vi "Beampointing_Multi_Pico3_upstairs01.vi"() -> ()   [LabVIEW 2020]
uses:
  Shared/GUI_Template/GUI_master/tcp_new_data_event.ctl
  Shared/GUI_Template/GUI_master/tcp new data cluster.ctl
  Ctrs/beam detection.ctl
  GUI_Beampointing_single_TRA/Ctrs/move.ctl
  General GUIs/Device GUIs/GUI_Cameras/Controls/Crosshair type def.ctl
  <vilib>/Utility/error.llb/DialogType.ctl
  <vilib>/Utility/file.llb/Read From Spreadsheet File (string).vi
  <userlib>/_OpenG.lib/array/array.llb/Filter 1D Array with Scalar (String)__ogtk.vi
  <userlib>/_OpenG.lib/array/array.llb/Filter 1D Array (String)__ogtk.vi
  <vilib>/Utility/file.llb/Write To Spreadsheet File (string).vi
  <vilib>/Analysis/NI_AALBase.lvlib
panel:
  out "x-y*floor(x/y)":dbl
  out "error out":errorcluster
  out "config path":string
  out "Array 3":bool[](array[boolean])
  out "Array 2":u16[](array[numeric])
  out "Array":u16[](array[numeric])
  out "Moving Y":string
  out "Moving X":string
  out "particles":T1(array[cluster])
  out "millisecond timer value":u32
  out "appended path":path
  out "millisecond timer 2":u32
  in  "GUIdevice 98":string="PicoPad4"
  in  "Position.Axis 111::98":dbl=77.0 caption="Motor Axis 1" min=-30000.0 max=30000.0 format="%#_6f"
  in  "Position.Axis 112::98":dbl=77.0 caption="Motor Axis 1" min=-20000.0 max=20000.0 format="%#_6f"
  in  "Position.Axis 113::98":dbl=77.0 caption="Motor Axis 1" min=-20000.0 max=20000.0 format="%#_6f"
  in  "Position.Axis 121::98":dbl=77.0 caption="Motor Axis 1" min=-999999.0 max=999999.0 format="%#_6f"
  in  "Position.Axis 122::98":dbl=77.0 caption="Motor Axis 1" min=-999999.0 max=999999.0 format="%#_6f"
  in  "Position.Axis 123::98":dbl=77.0 caption="Motor Axis 1" min=-999999.0 max=999999.0 format="%#_6f"
  in  "Position.Axis 131::98":dbl=77.0 caption="Motor Axis 1" min=-999999.0 max=999999.0 format="%#_6f"
  in  "Position.Axis 132::98":dbl=77.0 caption="Motor Axis 1" min=-999999.0 max=999999.0 format="%#_6f"
  in  "Position.Axis 133::98":dbl=77.0 caption="Motor Axis 1" min=-999999.0 max=999999.0 format="%#_6f"
  in  "Position.Axis 141::98":dbl=77.0 caption="Motor Axis 1" min=-999999.0 max=999999.0 format="%#_6f"
  in  "Position.Axis 142::98":dbl=77.0 caption="Motor Axis 1" min=-999999.0 max=999999.0 format="%#_6f"
  in  "Position.Axis 143::98":dbl=77.0 caption="Motor Axis 1" min=-999999.0 max=999999.0 format="%#_6f"
  in  "Position.Axis 211::98":dbl=77.0 caption="Motor Axis 1" min=-999999.0 max=999999.0 format="%#_6f"
  in  "Position.Axis 212::98":dbl=77.0 caption="Motor Axis 1" min=-999999.0 max=999999.0 format="%#_6f"
  in  "Position.Axis 213::98":dbl=77.0 caption="Motor Axis 1" min=-999999.0 max=999999.0 format="%#_6f"
  in  "Position.Axis 221::98":dbl=77.0 caption="Motor Axis 1" min=-999999.0 max=999999.0 format="%#_6f"
  in  "Position.Axis 222::98":dbl=77.0 caption="Motor Axis 1" min=-999999.0 max=999999.0 format="%#_6f"
  in  "Position.Axis 223::98":dbl=77.0 caption="Motor Axis 1" min=-999999.0 max=999999.0 format="%#_6f"
  in  "Position.Axis 231::98":dbl=77.0 caption="Motor Axis 1" min=-999999.0 max=999999.0 format="%#_6f"
  in  "Position.Axis 232::98":dbl=77.0 caption="Motor Axis 1" min=-999999.0 max=999999.0 format="%#_6f"
  in  "Position.Axis 233::98":dbl=77.0 caption="Motor Axis 1" min=-999999.0 max=999999.0 format="%#_6f"
  in  "Position.Axis 241::98":dbl=77.0 caption="Motor Axis 1" min=-999999.0 max=999999.0 format="%#_6f"
  in  "Position.Axis 242::98":dbl=77.0 caption="Motor Axis 1" min=-999999.0 max=999999.0 format="%#_6f"
  in  "Position.Axis 243::98":dbl=77.0 caption="Motor Axis 1" min=-999999.0 max=999999.0 format="%#_6f"
  in  "Position.Axis 311::98":dbl=77.0 caption="Motor Axis 1" min=-999999.0 max=999999.0 format="%#_6f"
  in  "Position.Axis 312::98":dbl=77.0 caption="Motor Axis 1" min=-999999.0 max=999999.0 format="%#_6f"
  in  "Position.Axis 313::98":dbl=77.0 caption="Motor Axis 1" min=-999999.0 max=999999.0 format="%#_6f"
  in  "Position.Axis 321::98":dbl=77.0 caption="Motor Axis 1" min=-999999.0 max=999999.0 format="%#_6f"
  in  "Position.Axis 322::98":dbl=77.0 caption="Motor Axis 1" min=-999999.0 max=999999.0 format="%#_6f"
  in  "Position.Axis 323::98":dbl=77.0 caption="Motor Axis 1" min=-999999.0 max=999999.0 format="%#_6f"
  in  "Position.Axis 331::98":dbl=77.0 caption="Motor Axis 1" min=-999999.0 max=999999.0 format="%#_6f"
  in  "Position.Axis 332::98":dbl=77.0 caption="Motor Axis 1" min=-999999.0 max=999999.0 format="%#_6f"
  in  "Position.Axis 333::98":dbl=77.0 caption="Motor Axis 1" min=-999999.0 max=999999.0 format="%#_6f"
  in  "Position.Axis 341::98":dbl=77.0 caption="Motor Axis 1" min=-999999.0 max=999999.0 format="%#_6f"
  in  "Position.Axis 342::98":dbl=77.0 caption="Motor Axis 1" min=-999999.0 max=999999.0 format="%#_6f"
  in  "Position.Axis 343::98":dbl=77.0 caption="Motor Axis 1" min=-999999.0 max=999999.0 format="%#_6f"
  in  "Position.Axis 411::98":dbl=77.0 caption="Motor Axis 1" min=-999999.0 max=999999.0 format="%#_6f"
  in  "Position.Axis 412::98":dbl=77.0 caption="Motor Axis 1" min=-999999.0 max=999999.0 format="%#_6f"
  in  "Position.Axis 413::98":dbl=77.0 caption="Motor Axis 1" min=-999999.0 max=999999.0 format="%#_6f"
  in  "Position.Axis 421::98":dbl=77.0 caption="Motor Axis 1" min=-999999.0 max=999999.0 format="%#_6f"
  in  "Position.Axis 422::98":dbl=77.0 caption="Motor Axis 1" min=-999999.0 max=999999.0 format="%#_6f"
  in  "Position.Axis 423::98":dbl=77.0 caption="Motor Axis 1" min=-999999.0 max=999999.0 format="%#_6f"
  in  "Position.Axis 431::98":dbl=77.0 caption="Motor Axis 1" min=-999999.0 max=999999.0 format="%#_6f"
  in  "Position.Axis 432::98":dbl=77.0 caption="Motor Axis 1" min=-999999.0 max=999999.0 format="%#_6f"
  in  "Position.Axis 433::98":dbl=77.0 caption="Motor Axis 1" min=-999999.0 max=999999.0 format="%#_6f"
  in  "Position.Axis 441::98":dbl=77.0 caption="Motor Axis 1" min=-999999.0 max=999999.0 format="%#_6f"
  in  "Position.Axis 442::98":dbl=77.0 caption="Motor Axis 1" min=-999999.0 max=999999.0 format="%#_6f"
  in  "Position.Axis 443::98":dbl=77.0 caption="Motor Axis 1" min=-999999.0 max=999999.0 format="%#_6f"
  in  "Position.Axis 511::98":dbl=77.0 caption="Motor Axis 1" min=-999999.0 max=999999.0 format="%#_6f"
  in  "Position.Axis 512::98":dbl=77.0 caption="Motor Axis 1" min=-999999.0 max=999999.0 format="%#_6f"
  in  "Position.Axis 513::98":dbl=77.0 caption="Motor Axis 1" min=-999999.0 max=999999.0 format="%#_6f"
  in  "Position.Axis 521::98":dbl=77.0 caption="Motor Axis 1" min=-999999.0 max=999999.0 format="%#_6f"
  in  "Position.Axis 522::98":dbl=77.0 caption="Motor Axis 1" min=-999999.0 max=999999.0 format="%#_6f"
  in  "Position.Axis 523::98":dbl=77.0 caption="Motor Axis 1" min=-999999.0 max=999999.0 format="%#_6f"
  in  "Position.Axis 531::98":dbl=77.0 caption="Motor Axis 1" min=-999999.0 max=999999.0 format="%#_6f"
  in  "Position.Axis 532::98":dbl=77.0 caption="Motor Axis 1" min=-999999.0 max=999999.0 format="%#_6f"
  in  "Position.Axis 533::98":dbl=77.0 caption="Motor Axis 1" min=-999999.0 max=999999.0 format="%#_6f"
  in  "Position.Axis 541::98":dbl=77.0 caption="Motor Axis 1" min=-999999.0 max=999999.0 format="%#_6f"
  in  "Position.Axis 542::98":dbl=77.0 caption="Motor Axis 1" min=-999999.0 max=999999.0 format="%#_6f"
  in  "Position.Axis 543::98":dbl=77.0 caption="Motor Axis 1" min=-999999.0 max=999999.0 format="%#_6f"
  in  "Numeric":dbl
  out "Current State":string
  in  "output cluster 2":T5 {"detection para"."smal para"."Measurement Parameter" items=["Center of Mass X", "Center of Mass Y", "First Pixel X", "First Pixel Y", "Bounding Rect Left", "Bounding Rect Top", "Bounding Rect Right", "Bounding Rect Bottom", "Max Feret Diameter Start X", "Max Feret Diameter Start Y", "Max Feret Diameter End X", "Max Feret Diameter End Y", "Max Horiz. Segment Length Left", "Max Horiz. Segment Length Right", "Max Horiz. Segment Length Row", "-", "Bounding Rect Width", "Bounding Rect Height", "Bounding Rect Diagonal", "Perimeter", "Convex Hull Perimeter", "Holes' Perimeter", "Max Feret Diameter", "Equivalent Ellipse Major Axis", "Equivalent Ellipse Minor Axis", "Equivalent Ellipse Minor Axis (Feret)", "Equivalent Rect Long Side", "Equivalent Rect Short Side", "Equivalent Rect Diagonal", "Equivalent Rect Short Side (Feret)", "Average Horiz. Segment Length", "Average Vert. Segment Length", "Hydraulic Radius", "Waddel Disk Diameter", "-", "Area", "Holes' Area", "Particle & Holes' Area", "Convex Hull Area", "Image Area", "-", "Number of Holes", "Number of Horiz. Segments", "Number of Vert. Segments", "-", "Orientation", "Max Feret Diameter Orientation", "-", "% Area/Image Area", "% Area/(Particle & Holes' Area)", "Ratio of Equivalent Ellipse Axes", "Ratio of Equivalent Rect Sides", "-", "Elongation Factor", "Compactness Factor", "Heywood Circularity Factor", "Type Factor", "-", "Sum X", "Sum Y", "Sum XX", "Sum XY", "Sum YY", "Sum XXX", "Sum XXY", "Sum XYY", "Sum YYY", "-", "Moment of Inertia XX", "Moment of Inertia XY", "Moment of Inertia YY", "Moment of Inertia XXX", "Moment of Inertia XXY", "Moment of Inertia XYY", "Moment of Inertia YYY", "Norm. Moment of Inertia XX", "Norm. Moment of Inertia XY", "Norm. Moment of Inertia YY", "Norm. Moment of Inertia XXX", "Norm. Moment of Inertia XXY", "Norm. Moment of Inertia XYY", "Norm. Moment of Inertia YYY", "Hu Moment 1", "Hu Moment 2", "Hu Moment 3", "Hu Moment 4", "Hu Moment 5", "Hu Moment 6", "Hu Moment 7"]; "detection para"."smal para"."Range Lower Value" format="%.2f"; "detection para"."smal para"."Range Upper Value" format="%.2f"; "detection para"."detection method" items=["clustering", "entropy", "metric", "moments", "inter-class variance"]; "detection para"."Filter" items=["No Filter", "Median Filter", "Low Pass Filter"]}
  out "CCDs":string[](array[string])
  in  "GUIdevice 12":string
  in  "GUIdevice 11":string
  in  "GUIdevice 10":string
  in  "GUIdevice 9":string
  out "error out 2":errorcluster
  in  "active cams":string[](array[string])
  in  "Motor Y":dbl[][](array[numeric])
  in  "Motor X":dbl[][](array[numeric])
  out "Names":string[](array[string])
  in  "Offset X stats":dbl[][](array[numeric])
  in  "Offset Y stats":dbl[][](array[numeric])
  out "Box":T6(array[cluster])
  in  "Tab Control 2":enum32{"Config ", "Main", "History"}(tab)=enum."Main"
  out "Waveform Chart":u32(graph)
  in  "associated motors":T7
  out "Cameras":T8
  out "Status":cluster{i32, i32, "Centroid X":dbl[][]}(graph)
  in  "Exposure:12":dbl=0.095 min=0.0001 max=1.0 format="%#_6f"
  in  "Triggerdelay::12":dbl=0.003 min=0.0 max=0.09 format="%#_6f"
  in  "Exposure::11":dbl=0.095 min=0.0001 max=1.0 format="%#_6f"
  in  "Triggerdelay::11":dbl=0.003 min=0.0 max=0.09 format="%#_6f"
  in  "Exposure::10":dbl=0.095 min=0.0001 max=1.0 format="%#_6f"
  in  "Triggerdelay::10":dbl=0.003 min=0.0 max=0.09 format="%#_6f"
  in  "Exposure::9":dbl=0.095 min=0.0001 max=1.0 format="%#_6f"
  in  "Triggerdelay::9":dbl=0.003 min=0.0 max=0.09 format="%#_6f"
  in  "Trigger::9":bool
  in  "Trigger::10":bool caption="Trigger:10"
  in  "Trigger::11":bool
  in  "Trigger::12":bool
  in  "Target.Y::9":dbl=45.0 caption="T9y" min=0.0 max=2000.0 format="%#_6f"
  in  "Target.X::9":dbl=47.0 caption="Tx9" min=0.0 max=2000.0 format="%#_6f"
  in  "Target.Y::10":dbl=45.0 caption="T10y" min=0.0 max=2000.0 format="%#_6f"
  in  "Target.X::10":dbl=47.0 caption="T10x" min=0.0 max=2000.0 format="%#_6f"
  in  "Target.Y::11":dbl=45.0 caption="T11y" min=0.0 max=2000.0 format="%#_6f"
  in  "Target.X::11":dbl=47.0 caption="T11x" min=0.0 max=2000.0 format="%#_6f"
  in  "Target.Y::12":dbl=45.0 caption="T12y" min=0.0 max=2000.0 format="%#_6f"
  in  "Target.X::12":dbl=47.0 caption="T12x" min=0.0 max=2000.0 format="%#_6f"
  in  "Exposure::8":dbl=0.095 min=0.0001 max=1.0 format="%#_6f"
  in  "Triggerdelay::8":dbl=0.003 min=0.0 max=0.09 format="%#_6f"
  in  "Trigger::8":bool
  in  "Target.Y::8":dbl=45.0 caption="T8y" min=0.0 max=2000.0 format="%#_6f"
  in  "Target.X::8":dbl=47.0 caption="T8x" min=0.0 max=2000.0 format="%#_6f"
  in  "Target.Y::7":dbl=45.0 caption="T7x" min=0.0 max=2000.0 format="%#_6f"
  in  "Target.X::7":dbl=47.0 caption="T7y" min=0.0 max=2000.0 format="%#_6f"
  in  "Target.Y::6":dbl=45.0 caption="T6y" min=1.0 max=600.0 format="%#_6f"
  in  "Target.X::6":dbl=47.0 caption="T6x" min=1.0 max=800.0 format="%#_6f"
  in  "Target.Y::5":dbl=45.0 caption="T5y" min=0.0 max=2000.0 format="%#_6f"
  in  "Target.X::5":dbl=47.0 caption="T5x" min=0.0 max=2000.0 format="%#_6f"
  in  "Target.Y::4":dbl=45.0 caption="T4y" min=1.0 max=600.0 format="%#_6f"
  in  "Target.X::4":dbl=47.0 caption="T4x" min=1.0 max=800.0 format="%#_6f"
  in  "Target.Y::3":dbl=163.0 caption="T3y" min=0.0 max=2000.0 format="%#_6f"
  in  "Target.X::3":dbl=152.0 caption="T3x" min=0.0 max=2000.0 format="%#_6f"
  in  "Target.Y::2":dbl=74.0 caption="T2y" min=1.0 max=600.0 format="%#_6f"
  in  "Target.X::2":dbl=75.0 caption="T2x" min=1.0 max=800.0 format="%#_6f"
  in  "Target.Y::1":dbl=61.0 caption="T1y" min=1.0 max=600.0 format="%#_6f"
  in  "Target.X::1":dbl=77.0 caption="T1x" min=1.0 max=800.0 format="%#_6f"
  in  "Exposure::7":dbl=0.095 min=0.0001 max=1.0 format="%#_6f"
  in  "Triggerdelay::7":dbl=0.003 min=0.0 max=0.09 format="%#_6f"
  in  "Trigger::7":bool
  in  "Exposure::6":dbl=0.095 min=0.0001 max=1.0 format="%#_6f"
  in  "Triggerdelay::6":dbl=0.003 min=0.0 max=0.09 format="%#_6f"
  in  "Trigger::6":bool
  in  "Exposure::5":dbl=0.095 min=1e-05 max=2.0 format="%#_6f"
  in  "Triggerdelay::5":dbl=0.003 min=0.0 max=100000.0 format="%#_6f"
  in  "Trigger::5":bool
  in  "Exposure::4":dbl=0.095 min=0.0001 max=1.0 format="%#_6f"
  in  "Triggerdelay::4":dbl=0.003 min=0.0 max=0.09 format="%#_6f"
  in  "Trigger::4":bool
  in  "Exposure::3":dbl=0.095 min=1e-05 max=2.0 format="%#_6f"
  in  "Triggerdelay::3":dbl=0.003 min=0.0 max=0.09 format="%#_6f"
  in  "Trigger::3":bool
  in  "Exposure::2":dbl=0.095 min=0.0001 max=1.0 format="%#_6f"
  in  "Triggerdelay::2":dbl=0.003 min=0.0 max=0.09 format="%#_6f"
  in  "Trigger::2":bool
  out "image::1":T9(plugin-control) caption="regen-out-cam"
  out "image::2":T9(plugin-control) caption="xpw-cam"
  out "image::3":T9(plugin-control) caption="xpw-out-cam"
  out "image::4":T9(plugin-control) caption="amp0-out-cam"
  out "image::5":T9(plugin-control) caption="preamp-in-cam"
  out "image::6":T9(plugin-control) caption="preamp-2nd-pass-cam"
  out "image::7":T9(plugin-control) caption="compressor-in-cam"
  out "image::8":T9(plugin-control) caption="compressor-out-cam"
  in  "Exposure::1":dbl=0.095 caption="exposure" min=0.0001 max=1.0 format="%#_6f"
  in  "Triggerdelay::1":dbl=0.003 caption="trig delay" min=0.0 max=0.09 format="%#_6f"
  in  "Trigger::1":bool
  in  "UDP error message":string
  out "required Y":bool[](array[boolean])
  out "required X":bool[](array[boolean])
  out "detected":bool[](array[boolean])
  out "name array":string[](array[string])
  out "image::9":T9(plugin-control)
  out "image::10":T9(plugin-control)
  out "image::11":T9(plugin-control)
  out "image::12":T9(plugin-control)
  out "speedmode X":bool[](array[boolean])
  out "speedmode Y":bool[](array[boolean])
  out "CCD 9":cluster{timestamp[], dbl[]}[](graph)
  out "CCD 10":cluster{timestamp[], dbl[]}[](graph)
  out "CCD 11":cluster{timestamp[], dbl[]}[](graph)
  out "CCD 12":cluster{timestamp[], dbl[]}[](graph)
  out "CCD 5":cluster{timestamp[], dbl[]}[](graph)
  out "CCD 6":cluster{timestamp[], dbl[]}[](graph)
  out "CCD 7":cluster{timestamp[], dbl[]}[](graph)
  out "CCD 8":cluster{timestamp[], dbl[]}[](graph)
  out "CCD 2":cluster{timestamp[], dbl[]}[](graph)
  out "CCD 1":cluster{timestamp[], dbl[]}[](graph)
  out "CCD 3":cluster{timestamp[], dbl[]}[](graph)
  out "CCD 4":cluster{timestamp[], dbl[]}[](graph)
  out "History index":i32
  in  "History Size":i32=500
  out "Particle Reports (Pixels)":T10(array[cluster])
  in  "Feedback Global":bool
  in  "detection para":T3[](array[typedef])=[{"Filter"=1, "Filter Para"={"X Size"=5, "Y Size"=5, "% Tolerance"=1}, "detection method"=4, "smal para"=[{"Measurement Parameter"=35, "Range Lower Value"=0.0, "Range Upper Value"=0.0, "Range"=TRUE, "Measurement Type"=FALSE}], "Remove small Objects"=TRUE, "Restrict to round Objects"=FALSE}, {"Filter"=1, "Filter Para"={"X Size"=5, "Y Size"=5, "% Tolerance"=1}, "detection method"=4, "smal para"=[{"Measurement Parameter"=35, "Range Lower Value"=0.0, "Range Upper Value"=500.0, "Range"=FALSE, "Measurement Type"=FALSE}], "Remove small Objects"=TRUE, "Restrict to round Objects"=FALSE}, {"Filter"=1, "Filter Para"={"X Size"=5, "Y Size"=5, "% Tolerance"=1}, "detection method"=4, "smal para"=[{"Measurement Parameter"=35, "Range Lower Value"=0.0, "Range Upper Value"=500.0, "Range"=TRUE, "Measurement Type"=FALSE}], "Remove small Objects"=TRUE, "Restrict to round Objects"=FALSE}, {"Filter"=1, "Filter Para"={"X Size"=5, "Y Size"=5, "% Tolerance"=1}, "detection method"=4, "smal para"=[{"Measurement Parameter"=35, "Range Lower Value"=0.0, "Range Upper Value"=500.0, "Range"=TRUE, "Measurement Type"=FALSE}], "Remove small Objects"=TRUE, "Restrict to round Objects"=FALSE}, {"Filter"=1, "Filter Para"={"X Size"=5, "Y Size"=5, "% Tolerance"=1}, "detection method"=4, "smal para"=[{"Measurement Parameter"=35, "Range Lower Value"=0.0, "Range Upper Value"=500.0, "Range"=TRUE, "Measurement Type"=FALSE}], "Remove small Objects"=TRUE, "Restrict to round Objects"=FALSE}, {"Filter"=1, "Filter Para"={"X Size"=5, "Y Size"=5, "% Tolerance"=1}, "detection method"=4, "smal para"=[{"Measurement Parameter"=35, "Range Lower Value"=0.0, "Range Upper Value"=500.0, "Range"=TRUE, "Measurement Type"=FALSE}], "Remove small Objects"=TRUE, "Restrict to round Objects"=FALSE}, {"Filter"=1, "Filter Para"={"X Size"=5, "Y Size"=5, "% Tolerance"=1}, "detection method"=4, "smal para"=[{"Measurement Parameter"=35, "Range Lower Value"=0.0, "Range Upper Value"=500.0, "Range"=TRUE, "Measurement Type"=FALSE}], "Remove small Objects"=TRUE, "Restrict to round Objects"=FALSE}, {"Filter"=1, "Filter Para"={"X Size"=5, "Y Size"=5, "% Tolerance"=1}, "detection method"=3, "smal para"=[{"Measurement Parameter"=35, "Range Lower Value"=0.0, "Range Upper Value"=0.0, "Range"=FALSE, "Measurement Type"=FALSE}], "Remove small Objects"=TRUE, "Restrict to round Objects"=FALSE}, {"Filter"=1, "Filter Para"={"X Size"=5, "Y Size"=5, "% Tolerance"=1}, "detection method"=4, "smal para"=[{"Measurement Parameter"=35, "Range Lower Value"=0.0, "Range Upper Value"=0.0, "Range"=FALSE, "Measurement Type"=FALSE}], "Remove small Objects"=TRUE, "Restrict to round Objects"=FALSE}, {"Filter"=1, "Filter Para"={"X Size"=5, "Y Size"=5, "% Tolerance"=1}, "detection method"=4, "smal para"=[{"Measurement Parameter"=35, "Range Lower Value"=0.0, "Range Upper Value"=500.0, "Range"=TRUE, "Measurement Type"=FALSE}], "Remove small Objects"=TRUE, "Restrict to round Objects"=FALSE}, {"Filter"=1, "Filter Para"={"X Size"=5, "Y Size"=5, "% Tolerance"=1}, "detection method"=4, "smal para"=[{"Measurement Parameter"=35, "Range Lower Value"=0.0, "Range Upper Value"=500.0, "Range"=TRUE, "Measurement Type"=FALSE}], "Remove small Objects"=TRUE, "Restrict to round Objects"=FALSE}, {"Filter"=1, "Filter Para"={"X Size"=5, "Y Size"=5, "% Tolerance"=1}, "detection method"=4, "smal para"=[{"Measurement Parameter"=35, "Range Lower Value"=0.0, "Range Upper Value"=500.0, "Range"=TRUE, "Measurement Type"=FALSE}], "Remove small Objects"=TRUE, "Restrict to round Objects"=FALSE}] {"smal para"."Measurement Parameter" items=["Center of Mass X", "Center of Mass Y", "First Pixel X", "First Pixel Y", "Bounding Rect Left", "Bounding Rect Top", "Bounding Rect Right", "Bounding Rect Bottom", "Max Feret Diameter Start X", "Max Feret Diameter Start Y", "Max Feret Diameter End X", "Max Feret Diameter End Y", "Max Horiz. Segment Length Left", "Max Horiz. Segment Length Right", "Max Horiz. Segment Length Row", "-", "Bounding Rect Width", "Bounding Rect Height", "Bounding Rect Diagonal", "Perimeter", "Convex Hull Perimeter", "Holes' Perimeter", "Max Feret Diameter", "Equivalent Ellipse Major Axis", "Equivalent Ellipse Minor Axis", "Equivalent Ellipse Minor Axis (Feret)", "Equivalent Rect Long Side", "Equivalent Rect Short Side", "Equivalent Rect Diagonal", "Equivalent Rect Short Side (Feret)", "Average Horiz. Segment Length", "Average Vert. Segment Length", "Hydraulic Radius", "Waddel Disk Diameter", "-", "Area", "Holes' Area", "Particle & Holes' Area", "Convex Hull Area", "Image Area", "-", "Number of Holes", "Number of Horiz. Segments", "Number of Vert. Segments", "-", "Orientation", "Max Feret Diameter Orientation", "-", "% Area/Image Area", "% Area/(Particle & Holes' Area)", "Ratio of Equivalent Ellipse Axes", "Ratio of Equivalent Rect Sides", "-", "Elongation Factor", "Compactness Factor", "Heywood Circularity Factor", "Type Factor", "-", "Sum X", "Sum Y", "Sum XX", "Sum XY", "Sum YY", "Sum XXX", "Sum XXY", "Sum XYY", "Sum YYY", "-", "Moment of Inertia XX", "Moment of Inertia XY", "Moment of Inertia YY", "Moment of Inertia XXX", "Moment of Inertia XXY", "Moment of Inertia XYY", "Moment of Inertia YYY", "Norm. Moment of Inertia XX", "Norm. Moment of Inertia XY", "Norm. Moment of Inertia YY", "Norm. Moment of Inertia XXX", "Norm. Moment of Inertia XXY", "Norm. Moment of Inertia XYY", "Norm. Moment of Inertia YYY", "Hu Moment 1", "Hu Moment 2", "Hu Moment 3", "Hu Moment 4", "Hu Moment 5", "Hu Moment 6", "Hu Moment 7"]; "smal para"."Range Lower Value" format="%.2f"; "smal para"."Range Upper Value" format="%.2f"; "detection method" items=["clustering", "entropy", "metric", "moments", "inter-class variance"]; "Filter" items=["No Filter", "Median Filter", "Low Pass Filter"]}
  in  "GUIdevice 8":string="B5_CompressorOut"
  in  "Tab Control":T11(tab)
  in  "Center":bool
  in  "Save Stats":bool
  in  "Save Config":bool
  in  "Load Config":bool
  in  "update speed [ms]":i32=5000
  in  "Img to avg":i32=3 min=3 max=200
  in  "Reset History":bool
  in  "save path":path=path "W:/BP_DATA"
  in  "autodetect":bool
  in  "Detection Rate":dbl=0.8 min=0.001 max=1.0
  in  "new tdms":bool
  in  "Speedmode @":dbl=3.0 min=1.0 max=20.0
  in  "Align":bool
  in  "deivice ini":bool
  in  "beam detection para":T3={"Filter"=1, "Filter Para"={"X Size"=5, "Y Size"=5, "% Tolerance"=1}, "detection method"=4, "smal para"=[{"Measurement Parameter"=35, "Range Lower Value"=0.0, "Range Upper Value"=500.0, "Range"=FALSE, "Measurement Type"=FALSE}], "Remove small Objects"=TRUE, "Restrict to round Objects"=FALSE} {"smal para"."Measurement Parameter" items=["Center of Mass X", "Center of Mass Y", "First Pixel X", "First Pixel Y", "Bounding Rect Left", "Bounding Rect Top", "Bounding Rect Right", "Bounding Rect Bottom", "Max Feret Diameter Start X", "Max Feret Diameter Start Y", "Max Feret Diameter End X", "Max Feret Diameter End Y", "Max Horiz. Segment Length Left", "Max Horiz. Segment Length Right", "Max Horiz. Segment Length Row", "-", "Bounding Rect Width", "Bounding Rect Height", "Bounding Rect Diagonal", "Perimeter", "Convex Hull Perimeter", "Holes' Perimeter", "Max Feret Diameter", "Equivalent Ellipse Major Axis", "Equivalent Ellipse Minor Axis", "Equivalent Ellipse Minor Axis (Feret)", "Equivalent Rect Long Side", "Equivalent Rect Short Side", "Equivalent Rect Diagonal", "Equivalent Rect Short Side (Feret)", "Average Horiz. Segment Length", "Average Vert. Segment Length", "Hydraulic Radius", "Waddel Disk Diameter", "-", "Area", "Holes' Area", "Particle & Holes' Area", "Convex Hull Area", "Image Area", "-", "Number of Holes", "Number of Horiz. Segments", "Number of Vert. Segments", "-", "Orientation", "Max Feret Diameter Orientation", "-", "% Area/Image Area", "% Area/(Particle & Holes' Area)", "Ratio of Equivalent Ellipse Axes", "Ratio of Equivalent Rect Sides", "-", "Elongation Factor", "Compactness Factor", "Heywood Circularity Factor", "Type Factor", "-", "Sum X", "Sum Y", "Sum XX", "Sum XY", "Sum YY", "Sum XXX", "Sum XXY", "Sum XYY", "Sum YYY", "-", "Moment of Inertia XX", "Moment of Inertia XY", "Moment of Inertia YY", "Moment of Inertia XXX", "Moment of Inertia XXY", "Moment of Inertia XYY", "Moment of Inertia YYY", "Norm. Moment of Inertia XX", "Norm. Moment of Inertia XY", "Norm. Moment of Inertia YY", "Norm. Moment of Inertia XXX", "Norm. Moment of Inertia XXY", "Norm. Moment of Inertia XYY", "Norm. Moment of Inertia YYY", "Hu Moment 1", "Hu Moment 2", "Hu Moment 3", "Hu Moment 4", "Hu Moment 5", "Hu Moment 6", "Hu Moment 7"]; "smal para"."Range Lower Value" format="%.2f"; "smal para"."Range Upper Value" format="%.2f"; "detection method" items=["clustering", "entropy", "metric", "moments", "inter-class variance"]; "Filter" items=["No Filter", "Median Filter", "Low Pass Filter"]}
  in  "move config":T2={"Tolerance [%]"=0.1, "Stepsize"=0.0001, "Invert Axis"=TRUE, "Invert Direction X"=FALSE, "Invert Direction Y"=TRUE, "enable feedback"=FALSE, "Set Centriod Target"=FALSE}
  in  "ActiveMotor":u16(ring)=7 items=["preamp-in", "preamp-1st-pass", "xpw-cam", "L1_TelInpNear", "A", "B", "a", "D", "amp0-in", "TSa", "regen-out", "xpw-out", "Focuscam", "Mirrorcam", "preamp-3rd-pass", "", "", "", "", ""]
  in  "ActiveMotorName::99":string
  in  "RelativeMove.Axis 1.CCW::99":bool caption="RelativeMove.Axis 1.CCW::1"
  in  "RelativeMove.Axis 1.CW::99":bool caption="RelativeMove.Axis 1.CW::1"
  in  "RelativeMove.Axis 2.CCW::99":bool caption="RelativeMove.Axis. 2.CCW::1"
  in  "RelativeMove.Axis 2.CW::99":bool caption="RelativeMove.Axis 2.CW::1"
  in  "RelativeSettings.Axis 1.Position::99":dbl caption="Axis 1 Position" min=-999999.0 max=999999.0 format="%_4p"
  in  "RelativeSettings.Axis 2.Position::99":dbl caption="Axis 2 Position" min=-999999.0 max=999999.0 format="%_4p"
  in  "RelativeSettings.Axis 2.StepSize::99":dbl=50.0 caption="Axis 2 StepSize" min=0.0 max=999999.0 format="%_4p"
  in  "RelativeSettings.Axis 1.StepSize::99":dbl=50.0 caption="Axis 1 Stepsize" min=0.0 max=999999.0 format="%_4p"
  out "Arguments Y":string
  in  "active axis refs 2":T12(array[cluster])
  in  "active Axis ref":cluster{"Ref X":refnum<vi>, "Ref Y":refnum<vi>}
  in  "CCDs":u16(ring) items=["regen-out-cam", "xpw-cam", "xpw-out-cam", "amp0-out-cam", "preamp-in-cam", "preamp-2nd-pass-cam", "compressor-in-cam", "compressor-out-cam", "", "", "", ""]
  out "motor refs":refnum<vi>[](array[refnum])
  in  "Position.Axis 511::99":dbl=77.0 caption="Motor Axis 1" min=-999999.0 max=999999.0 format="%#_6f"
  in  "Position.Axis 512::99":dbl=77.0 caption="Motor Axis 1" min=-999999.0 max=999999.0 format="%#_6f"
  in  "Position.Axis 513::99":dbl=77.0 caption="Motor Axis 1" min=-999999.0 max=999999.0 format="%#_6f"
  in  "Position.Axis 521::99":dbl=77.0 caption="Motor Axis 1" min=-999999.0 max=999999.0 format="%#_6f"
  in  "Position.Axis 522::99":dbl=77.0 caption="Motor Axis 1" min=-999999.0 max=999999.0 format="%#_6f"
  in  "Position.Axis 523::99":dbl=77.0 caption="Motor Axis 1" min=-999999.0 max=999999.0 format="%#_6f"
  in  "Position.Axis 531::99":dbl=77.0 caption="Motor Axis 1" min=-999999.0 max=999999.0 format="%#_6f"
  in  "Position.Axis 532::99":dbl=77.0 caption="Motor Axis 1" min=-999999.0 max=999999.0 format="%#_6f"
  in  "Position.Axis 533::99":dbl=77.0 caption="Motor Axis 1" min=-999999.0 max=999999.0 format="%#_6f"
  in  "Position.Axis 541::99":dbl=77.0 caption="Motor Axis 1" min=-999999.0 max=999999.0 format="%#_6f"
  in  "Position.Axis 542::99":dbl=77.0 caption="Motor Axis 1" min=-999999.0 max=999999.0 format="%#_6f"
  in  "Position.Axis 543::99":dbl=77.0 caption="Motor Axis 1" min=-999999.0 max=999999.0 format="%#_6f"
  in  "Position.Axis 411::99":dbl=77.0 caption="Motor Axis 1" min=-999999.0 max=999999.0 format="%#_6f"
  in  "Position.Axis 412::99":dbl=77.0 caption="Motor Axis 1" min=-999999.0 max=999999.0 format="%#_6f"
  in  "Position.Axis 413::99":dbl=77.0 caption="Motor Axis 1" min=-999999.0 max=999999.0 format="%#_6f"
  in  "Position.Axis 421::99":dbl=77.0 caption="Motor Axis 1" min=-999999.0 max=999999.0 format="%#_6f"
  in  "Position.Axis 422::99":dbl=77.0 caption="Motor Axis 1" min=-999999.0 max=999999.0 format="%#_6f"
  in  "Position.Axis 423::99":dbl=77.0 caption="Motor Axis 1" min=-999999.0 max=999999.0 format="%#_6f"
  in  "Position.Axis 431::99":dbl=77.0 caption="Motor Axis 1" min=-999999.0 max=999999.0 format="%#_6f"
  in  "Position.Axis 432::99":dbl=77.0 caption="Motor Axis 1" min=-999999.0 max=999999.0 format="%#_6f"
  in  "Position.Axis 433::99":dbl=77.0 caption="Motor Axis 1" min=-999999.0 max=999999.0 format="%#_6f"
  in  "Position.Axis 441::99":dbl=77.0 caption="Motor Axis 1" min=-999999.0 max=999999.0 format="%#_6f"
  in  "Position.Axis 442::99":dbl=77.0 caption="Motor Axis 1" min=-999999.0 max=999999.0 format="%#_6f"
  in  "Position.Axis 443::99":dbl=77.0 caption="Motor Axis 1" min=-999999.0 max=999999.0 format="%#_6f"
  in  "Position.Axis 311::99":dbl=77.0 caption="Motor Axis 1" min=-999999.0 max=999999.0 format="%#_6f"
  in  "Position.Axis 312::99":dbl=77.0 caption="Motor Axis 1" min=-999999.0 max=999999.0 format="%#_6f"
  in  "Position.Axis 313::99":dbl=77.0 caption="Motor Axis 1" min=-999999.0 max=999999.0 format="%#_6f"
  in  "Position.Axis 321::99":dbl=77.0 caption="Motor Axis 1" min=-999999.0 max=999999.0 format="%#_6f"
  in  "Position.Axis 322::99":dbl=77.0 caption="Motor Axis 1" min=-999999.0 max=999999.0 format="%#_6f"
  in  "Position.Axis 323::99":dbl=77.0 caption="Motor Axis 1" min=-999999.0 max=999999.0 format="%#_6f"
  in  "Position.Axis 331::99":dbl=77.0 caption="Motor Axis 1" min=-999999.0 max=999999.0 format="%#_6f"
  in  "Position.Axis 332::99":dbl=77.0 caption="Motor Axis 1" min=-999999.0 max=999999.0 format="%#_6f"
  in  "Position.Axis 333::99":dbl=77.0 caption="Motor Axis 1" min=-999999.0 max=999999.0 format="%#_6f"
  in  "Position.Axis 341::99":dbl=77.0 caption="Motor Axis 1" min=-999999.0 max=999999.0 format="%#_6f"
  in  "Position.Axis 342::99":dbl=77.0 caption="Motor Axis 1" min=-999999.0 max=999999.0 format="%#_6f"
  in  "Position.Axis 343::99":dbl=77.0 caption="Motor Axis 1" min=-999999.0 max=999999.0 format="%#_6f"
  in  "Position.Axis 241::99":dbl=77.0 caption="Motor Axis 1" min=-999999.0 max=999999.0 format="%#_6f"
  in  "Position.Axis 242::99":dbl=77.0 caption="Motor Axis 1" min=-999999.0 max=999999.0 format="%#_6f"
  in  "Position.Axis 243::99":dbl=77.0 caption="Motor Axis 1" min=-999999.0 max=999999.0 format="%#_6f"
  in  "Position.Axis 231::99":dbl=77.0 caption="Motor Axis 1" min=-999999.0 max=999999.0 format="%#_6f"
  in  "Position.Axis 232::99":dbl=77.0 caption="Motor Axis 1" min=-999999.0 max=999999.0 format="%#_6f"
  in  "Position.Axis 233::99":dbl=77.0 caption="Motor Axis 1" min=-999999.0 max=999999.0 format="%#_6f"
  in  "Position.Axis 221::99":dbl=77.0 caption="Motor Axis 1" min=-999999.0 max=999999.0 format="%#_6f"
  in  "Position.Axis 222::99":dbl=77.0 caption="Motor Axis 1" min=-999999.0 max=999999.0 format="%#_6f"
  in  "Position.Axis 223::99":dbl=77.0 caption="Motor Axis 1" min=-999999.0 max=999999.0 format="%#_6f"
  in  "Position.Axis 211::99":dbl=77.0 caption="Motor Axis 1" min=-999999.0 max=999999.0 format="%#_6f"
  in  "Position.Axis 212::99":dbl=77.0 caption="Motor Axis 1" min=-999999.0 max=999999.0 format="%#_6f"
  in  "Position.Axis 213::99":dbl=77.0 caption="Motor Axis 1" min=-999999.0 max=999999.0 format="%#_6f"
  in  "Position.Axis 141::99":dbl=77.0 caption="Motor Axis 1" min=-999999.0 max=999999.0 format="%#_6f"
  in  "Position.Axis 142::99":dbl=77.0 caption="Motor Axis 1" min=-999999.0 max=999999.0 format="%#_6f"
  in  "Position.Axis 143::99":dbl=77.0 caption="Motor Axis 1" min=-999999.0 max=999999.0 format="%#_6f"
  in  "Position.Axis 131::99":dbl=77.0 caption="Motor Axis 1" min=-999999.0 max=999999.0 format="%#_6f"
  in  "Position.Axis 132::99":dbl=77.0 caption="Motor Axis 1" min=-999999.0 max=999999.0 format="%#_6f"
  in  "Position.Axis 133::99":dbl=77.0 caption="Motor Axis 1" min=-999999.0 max=999999.0 format="%#_6f"
  in  "Position.Axis 121::99":dbl=77.0 caption="Motor Axis 1" min=-999999.0 max=999999.0 format="%#_6f"
  in  "Position.Axis 122::99":dbl=77.0 caption="Motor Axis 1" min=-999999.0 max=999999.0 format="%#_6f"
  in  "Position.Axis 123::99":dbl=77.0 caption="Motor Axis 1" min=-999999.0 max=999999.0 format="%#_6f"
  in  "Position.Axis 113::99":dbl=77.0 caption="Motor Axis 1" min=-999999.0 max=999999.0 format="%#_6f"
  in  "Position.Axis 112::99":dbl=77.0 caption="Motor Axis 1" min=-999999.0 max=999999.0 format="%#_6f"
  in  "Position.Axis 111::99":dbl=77.0 caption="Motor Axis 1" min=-999999.0 max=999999.0 format="%#_6f"
  out "Arguments X":string
  in  "GUIdevice 99":string="253-picopad"
  in  "move properties":T2[](array[typedef])=[{"Tolerance [%]"=0.1, "Stepsize"=0.0001, "Invert Axis"=TRUE, "Invert Direction X"=FALSE, "Invert Direction Y"=TRUE, "enable feedback"=FALSE, "Set Centriod Target"=FALSE}, {"Tolerance [%]"=0.1, "Stepsize"=0.0001, "Invert Axis"=TRUE, "Invert Direction X"=FALSE, "Invert Direction Y"=TRUE, "enable feedback"=FALSE, "Set Centriod Target"=FALSE}, {"Tolerance [%]"=0.1, "Stepsize"=0.0001, "Invert Axis"=TRUE, "Invert Direction X"=FALSE, "Invert Direction Y"=TRUE, "enable feedback"=FALSE, "Set Centriod Target"=FALSE}, {"Tolerance [%]"=0.1, "Stepsize"=0.0001, "Invert Axis"=TRUE, "Invert Direction X"=FALSE, "Invert Direction Y"=TRUE, "enable feedback"=FALSE, "Set Centriod Target"=FALSE}, {"Tolerance [%]"=0.1, "Stepsize"=0.0001, "Invert Axis"=TRUE, "Invert Direction X"=FALSE, "Invert Direction Y"=TRUE, "enable feedback"=FALSE, "Set Centriod Target"=FALSE}, {"Tolerance [%]"=0.1, "Stepsize"=0.0001, "Invert Axis"=TRUE, "Invert Direction X"=FALSE, "Invert Direction Y"=TRUE, "enable feedback"=FALSE, "Set Centriod Target"=FALSE}, {"Tolerance [%]"=0.1, "Stepsize"=0.0001, "Invert Axis"=TRUE, "Invert Direction X"=FALSE, "Invert Direction Y"=TRUE, "enable feedback"=FALSE, "Set Centriod Target"=FALSE}, {"Tolerance [%]"=0.1, "Stepsize"=0.0001, "Invert Axis"=TRUE, "Invert Direction X"=FALSE, "Invert Direction Y"=TRUE, "enable feedback"=FALSE, "Set Centriod Target"=FALSE}, {"Tolerance [%]"=0.1, "Stepsize"=0.0001, "Invert Axis"=TRUE, "Invert Direction X"=FALSE, "Invert Direction Y"=TRUE, "enable feedback"=FALSE, "Set Centriod Target"=FALSE}, {"Tolerance [%]"=0.1, "Stepsize"=0.0001, "Invert Axis"=TRUE, "Invert Direction X"=FALSE, "Invert Direction Y"=TRUE, "enable feedback"=FALSE, "Set Centriod Target"=FALSE}, {"Tolerance [%]"=0.1, "Stepsize"=0.0001, "Invert Axis"=TRUE, "Invert Direction X"=FALSE, "Invert Direction Y"=TRUE, "enable feedback"=FALSE, "Set Centriod Target"=FALSE}, {"Tolerance [%]"=0.1, "Stepsize"=0.0001, "Invert Axis"=TRUE, "Invert Direction X"=FALSE, "Invert Direction Y"=TRUE, "enable feedback"=FALSE, "Set Centriod Target"=FALSE}, {"Tolerance [%]"=0.1, "Stepsize"=0.0001, "Invert Axis"=TRUE, "Invert Direction X"=FALSE, "Invert Direction Y"=TRUE, "enable feedback"=FALSE, "Set Centriod Target"=FALSE}]
  in  "Time":timestamp[][](array[timestamp])
  in  "Mean Size":dbl[][](array[numeric])
  in  "Size":dbl[][](array[numeric])
  in  "active CCDs":i32(listbox)=1
  in  "Offset Y":dbl[][](array[numeric])
  in  "Offset X":dbl[][](array[numeric])
  in  "Mean Centroid X":dbl[][](array[numeric])
  in  "Mean Centroid Y":dbl[][](array[numeric])
  in  "Centroid Y":dbl[][](array[numeric])
  in  "Centroid X":dbl[][](array[numeric])
  in  "GUIdevice 7":string="B2_TelLens1"
  in  "GUIdevice 6":string="B1_TelInput"
  in  "GUIdevice 5":string="L8_M10Leak"
  in  "GUIdevice 4":string="L7_TREXPass4"
  in  "GUIdevice 3":string="L6_TREXpass3"
  in  "GUIdevice 2":string="L5_TREXPass2"
  in  "insert tag":bool=TRUE
  in  "stop":bool
  in  "GUIdevice 1":string="L4_TREXpass1"
  out "tcp data event":T13
  out "error IO 2":errorcluster
  # "x [Tolerance]"
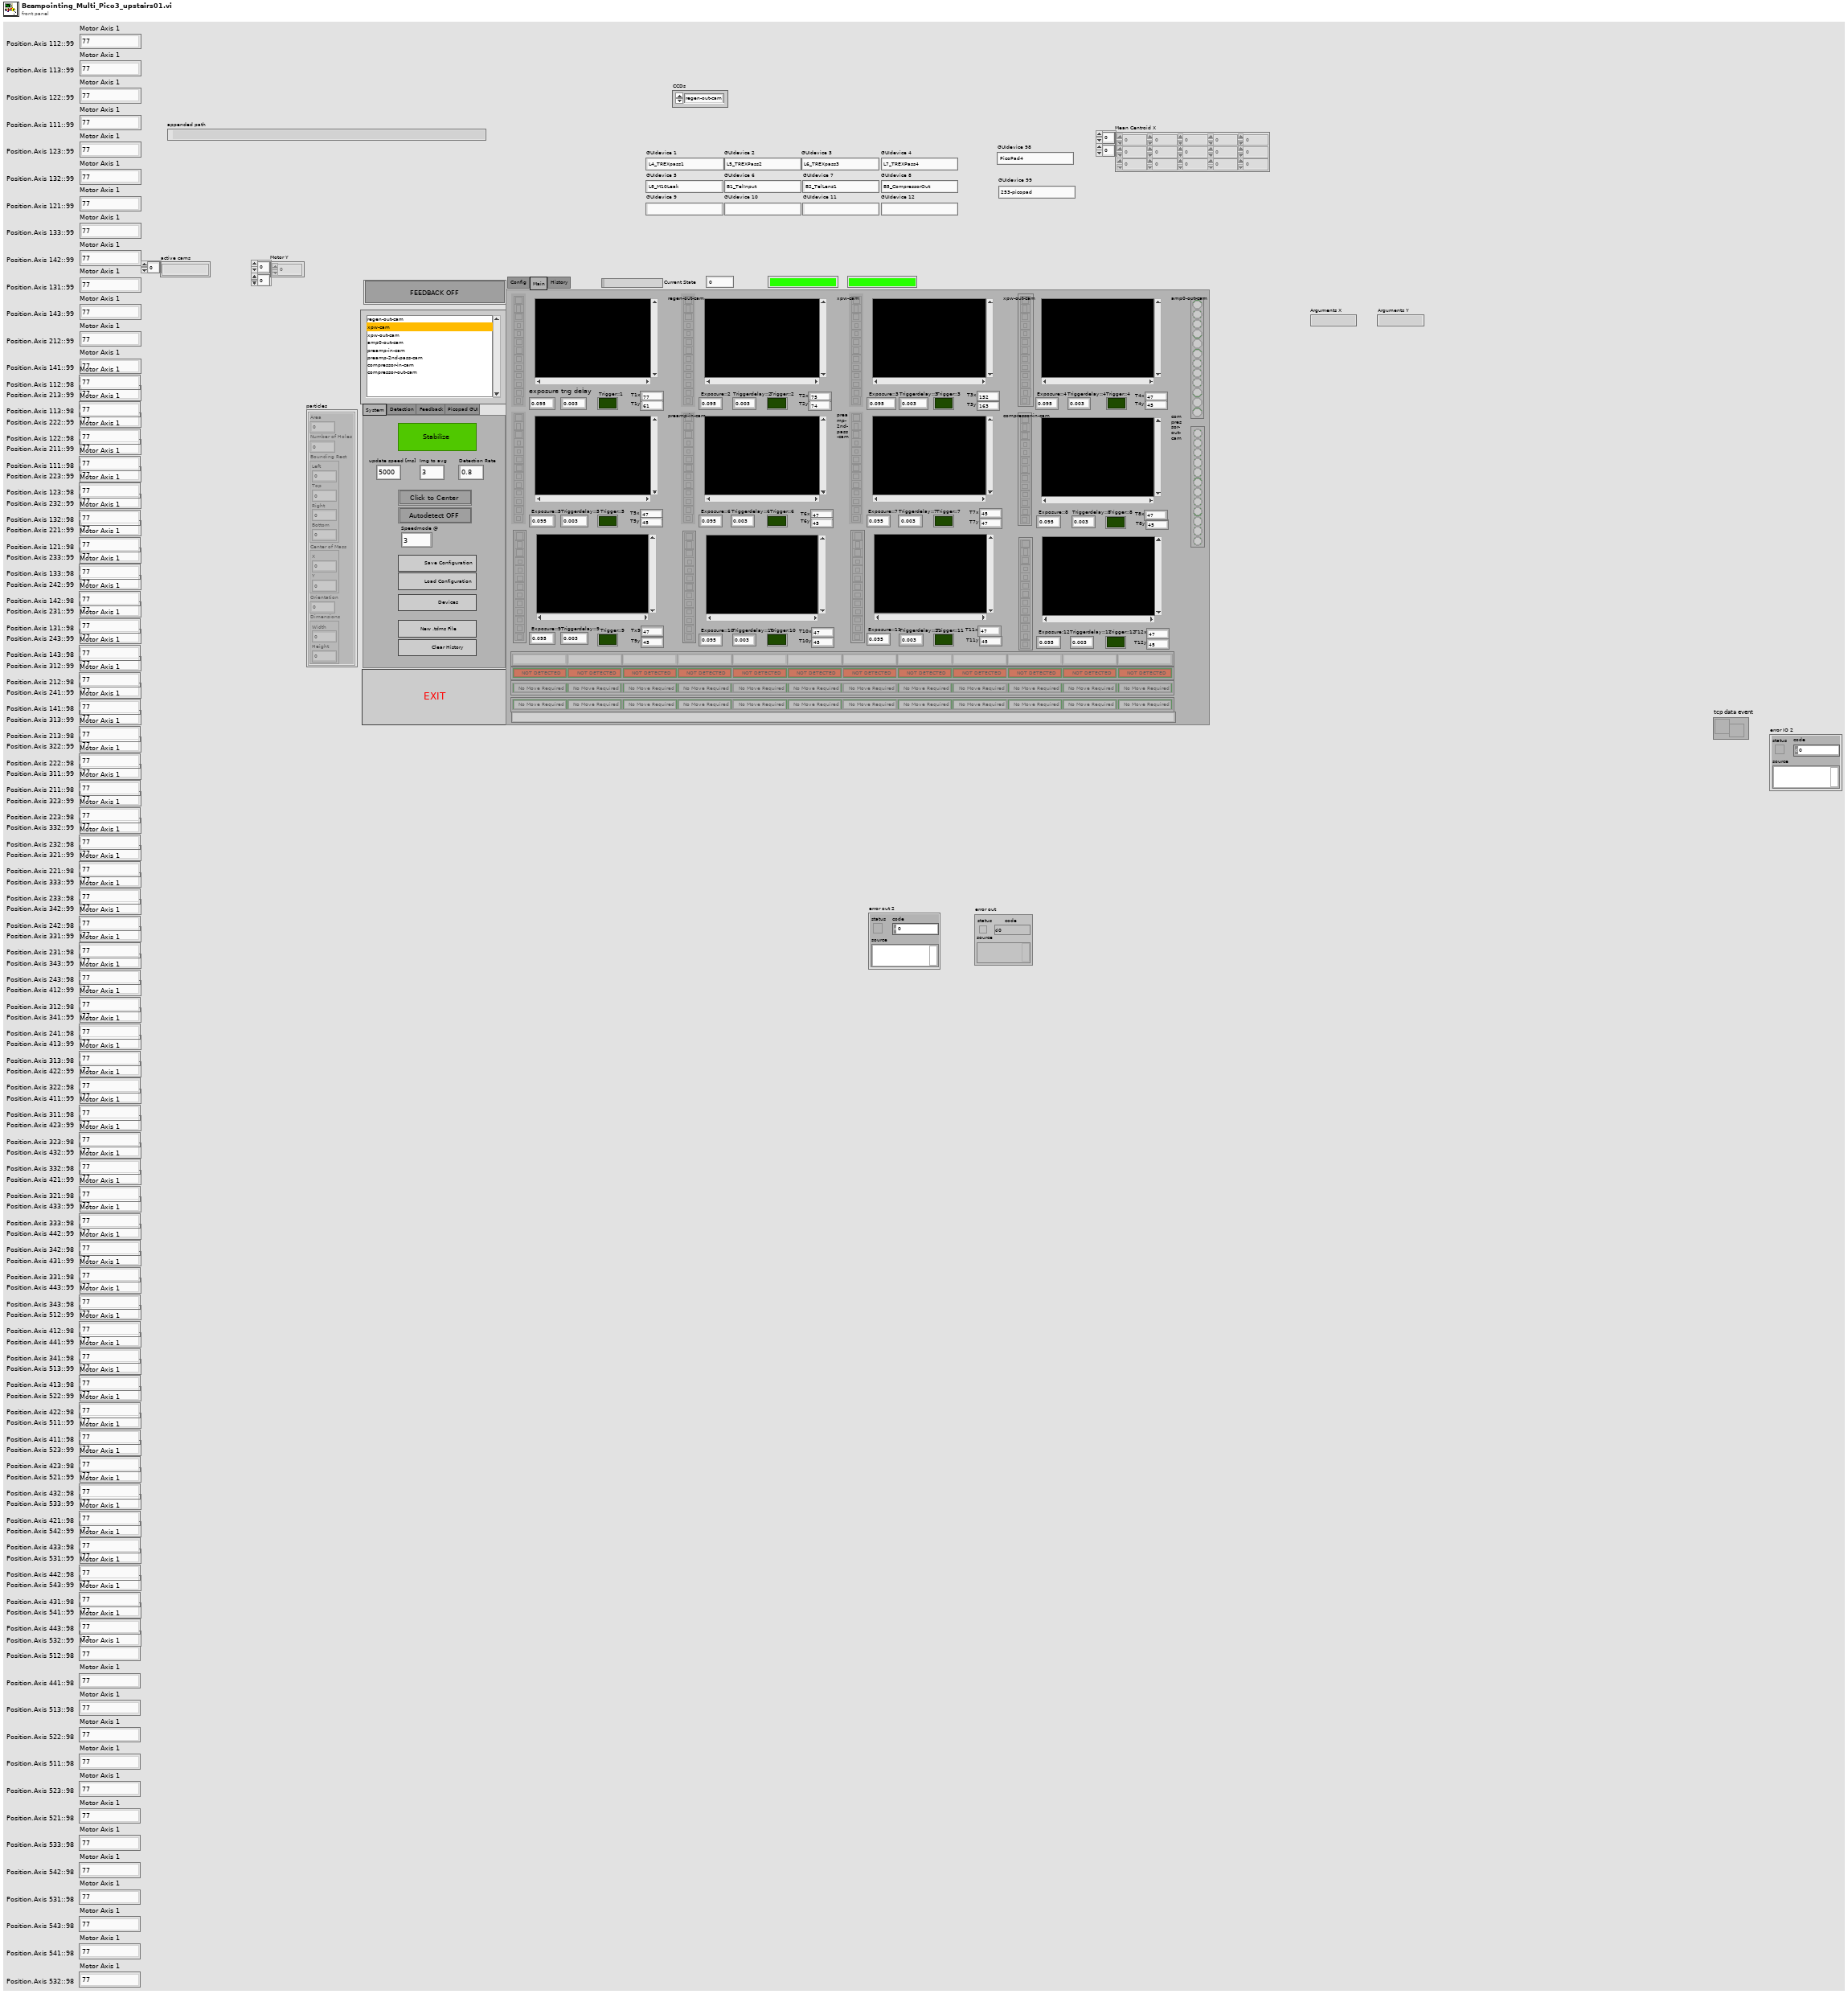
[diagram p1: front panel]
types:
  T1 = cluster{"Area":dbl, "Number of Holes":dbl, "Bounding Rect":cluster{"Left":dbl, "Top":dbl, "Right":dbl, "Bottom":dbl}, "Center of Mass":cluster{"X":dbl, "Y":dbl}, "Orientation":dbl, "Dimensions":cluster{"Width":dbl, "Height":dbl}}[]
  T2 = typedef "move.ctl" = cluster{"Tolerance [%]":dbl, "Stepsize":dbl, "Invert Axis":bool, "Invert Direction X":bool, "Invert Direction Y":bool, "enable feedback":bool, "Set Centriod Target":bool}
  T3 = typedef "beam detection.ctl" = cluster{"Filter":u16, "Filter Para":cluster{"X Size":i32, "Y Size":i32, "% Tolerance":i32}, "detection method":i32, "smal para":cluster{"Measurement Parameter":T4, "Range Lower Value":dbl, "Range Upper Value":dbl, "Range":bool, "Measurement Type":bool}[], "Remove small Objects":bool, "Restrict to round Objects":bool}
  T4 = typedef "Particle Parameters" = i32
  T5 = cluster{"CCDs":string[], "move properties":T2[], "detection para":T3[], "thresholds":cluster{"Lower value":sgl, "Upper value":sgl}[], "Value":cluster{"Motor CCD 1":u16, "Motor CCD 2":u16, "Motor CCD 3":u16, "Motor CCD 4":u16, "Motor CCD 5":u16, "Motor CCD 6":u16, "Motor CCD 7":u16, "Motor CCD 8":u16, "Motor CCD 9":u16, "Motor CCD 10":u16, "Motor CCD 11":u16, "Motor CCD 12":u16}}
  T6 = cluster{"Left":dbl, "Top":dbl, "Right":dbl, "Bottom":dbl}[]
  T7 = cluster{"Motor CCD 1":u16, "Motor CCD 2":u16, "Motor CCD 3":u16, "Motor CCD 4":u16, "Motor CCD 5":u16, "Motor CCD 6":u16, "Motor CCD 7":u16, "Motor CCD 8":u16, "Motor CCD 9":u16, "Motor CCD 10":u16, "Motor CCD 11":u16, "Motor CCD 12":u16}
  T8 = cluster{"[0]":string, "[1]":string, "[2]":string, "[3]":string, "[4]":string, "[5]":string, "[6]":string, "[7]":string, "[8]":string, "[8] 2":string, "[8] 3":string, "[8] 4":string}
  T9 = typedef "IMAQ Image.ctl" = refnum<image>
  T10 = cluster{"Area":dbl, "Number of Holes":dbl, "Bounding Rect":cluster{"Left":dbl, "Top":dbl, "Right":dbl, "Bottom":dbl}, "Center of Mass":cluster{"X":dbl, "Y":dbl}, "Orientation":dbl, "Dimensions":cluster{"Width":dbl, "Height":dbl}}[][]
  T11 = enum32{"System", "Detection", "Feedback", "Picopad GUI"}
  T12 = cluster{"Ref X":refnum<vi>, "Ref Y":refnum<vi>}[]
  T13 = typedef "tcp_new_data_event.ctl" = refnum<user-event>
  T14 = typedef "Crosshair type def.ctl" = cluster{"Draw":bool, "Target":cluster{"x":dbl, "y":dbl}, "Size":cluster{"x":dbl, "y":dbl}, "Angle":dbl, "Color":u32, "Thickness":u8, "CrosshairLabel":string}
  T15 = typedef "tcp new data cluster.ctl" = cluster{"EventEnum":enum16{"new data", "connection status update"}, "Device name":string}
  T16 = cluster{"Left":i32, "Top":i32, "Right":i32, "Bottom":i32}
  T17 = enum32{"invalid app kind", "Development System", "Run Time System", "Student Edition", "Embedded LabVIEW", "Evaluation", "Custom"}
  T18 = enum16{"open", "open or create", "create or replace", "create", "open (read-only)"}
  T19 = enum32{"Invalid", "Standard", "Closed", "Hidden", "Minimized", "Maximized"}
  T20 = enum16{"open", "replace", "create", "open or create", "replace or create", "replace or create with confirmation"}
  T21 = typedef "Image Type" = u32
  T22 = cluster{"[0]":string, "[1]":string, "[2]":string, "[3]":string, "[4]":string, "[5]":string, "[6]":string, "[7]":string, "[8]":string, "[9]":string, "[10]":string, "[11]":string}
  T23 = cluster{"Target.X::1":refnum<vi>, "Target.Y::1":refnum<vi>}
  T24 = cluster{"Target.X::2":refnum<vi>, "Target.Y::2":refnum<vi>}
  T25 = cluster{"Target.X::3":refnum<vi>, "Target.Y::3":refnum<vi>}
  T26 = cluster{"Target.X::4":refnum<vi>, "Target.Y::4":refnum<vi>}
  T27 = cluster{"Target.X::5":refnum<vi>, "Target.Y::5":refnum<vi>}
  T28 = cluster{"Target.X::6":refnum<vi>, "Target.Y::6":refnum<vi>}
  T29 = cluster{"Target.X::7":refnum<vi>, "Target.Y::7":refnum<vi>}
  T30 = cluster{"Target.X::8":refnum<vi>, "Target.Y::8":refnum<vi>}
  T31 = cluster{"Target.X::12":refnum<vi>, "Target.Y::12":refnum<vi>}
  T32 = cluster{"Target.X::9":refnum<vi>, "Target.Y::9":refnum<vi>}
  T33 = cluster{"Target.X::10":refnum<vi>, "Target.Y::10":refnum<vi>}
  T34 = cluster{"Target.X::11":refnum<vi>, "Target.Y::11":refnum<vi>}
  T35 = cluster{"Target.X::12":refnum<vi>, "Target.Y::12":refnum<vi>}[]
  T36 = cluster{"Left":dbl, "Top":dbl, "Right":dbl, "Bottom":dbl}
  T37 = cluster{"Core":cluster{"Current VI Reference":refnum<vi>, "Close Panel on Exit?":bool}, "detection para":T3[], "thresholds":cluster{"Lower value":sgl, "Upper value":sgl}[], "Centroid X":dbl[][], "Centroid Y":dbl[][], "img to avg":i32, "Mean Centroid X":dbl[][], "Mean Centroid Y":dbl[][], "Offset X":dbl[][], "Offset Y":dbl[][], "Offset X stats ":dbl[][], "Offset Y stats ":dbl[][], "Size":dbl[][], "Mean Size":dbl[][], "Time":timestamp[][], "move properties":T2[], "active axis refs 2":cluster{"Ref X":refnum<vi>, "Ref Y":refnum<vi>}[], "active ccd":i32, "Feedback global":bool, "Motor X":dbl[][], "Motor Y":dbl[][], "active cams":string[], "Data Value Reference out":refnum<k34>, "detected":bool[], "speedmode X":bool[], "speedmode Y":bool[]}
  T38 = typedef "DialogType.ctl" = u16
  T39 = cluster{"Current VI Reference":refnum<vi>, "Close Panel on Exit?":bool}
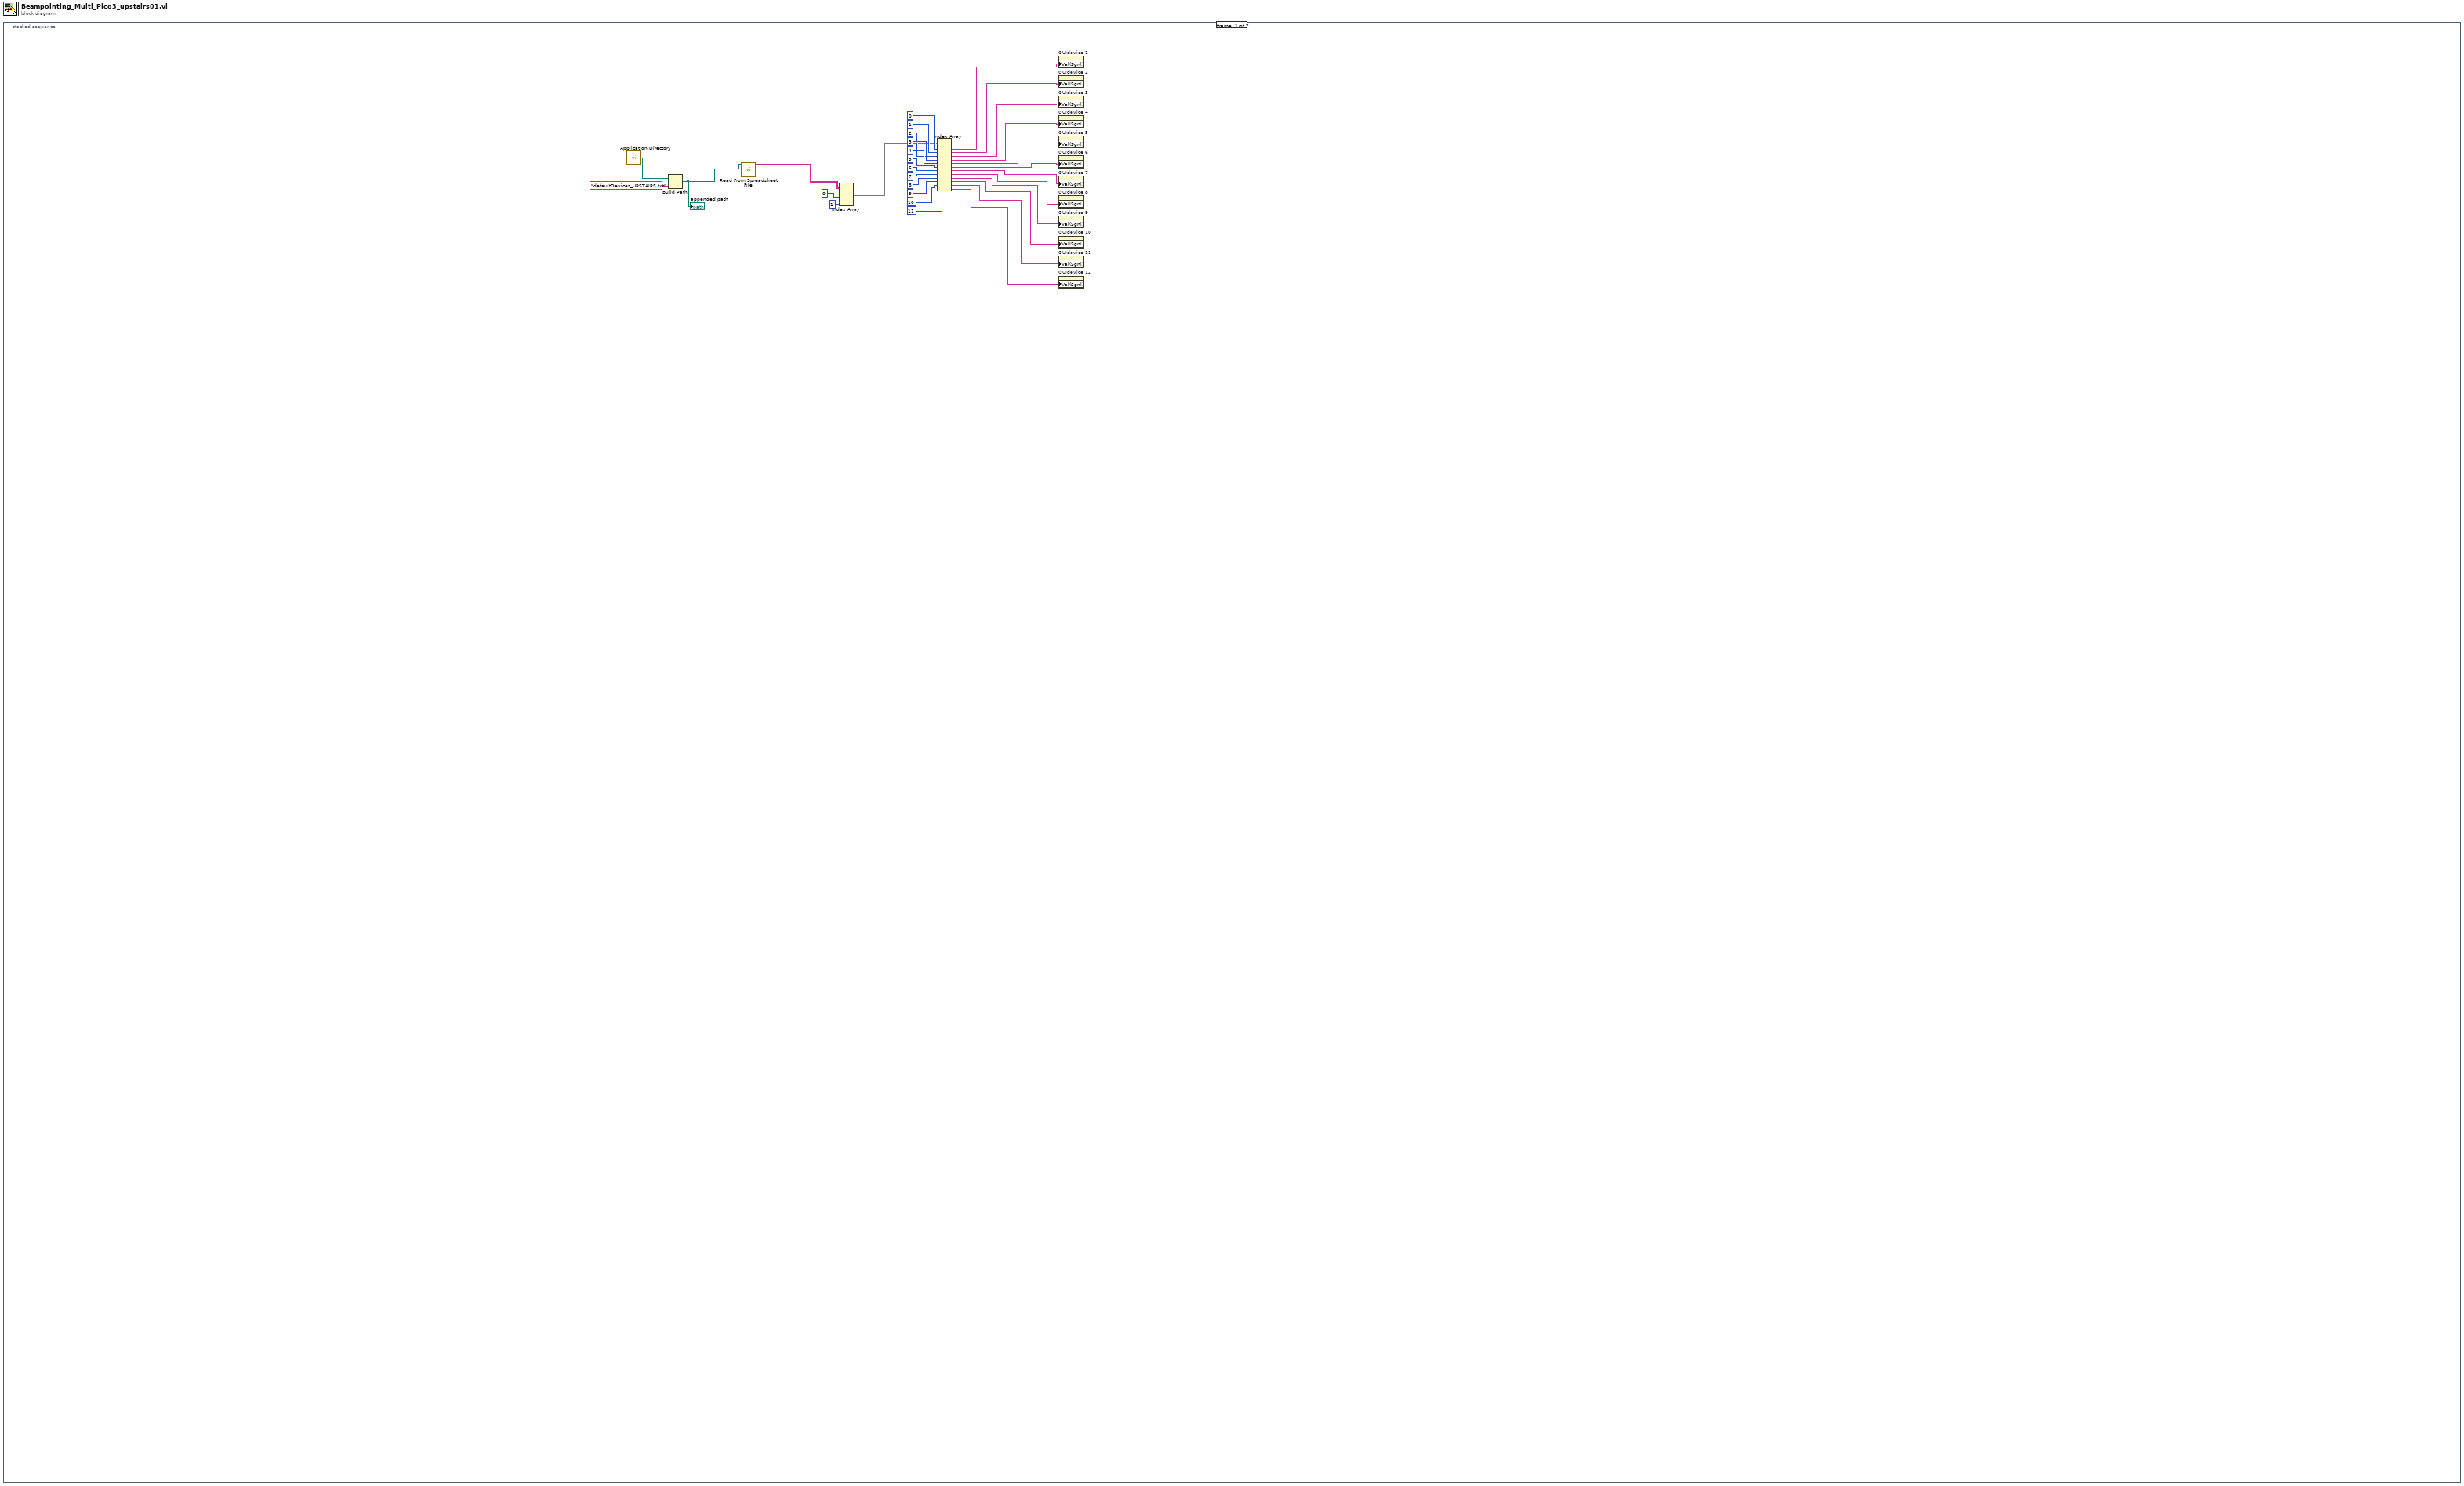
[diagram p0: block diagram]
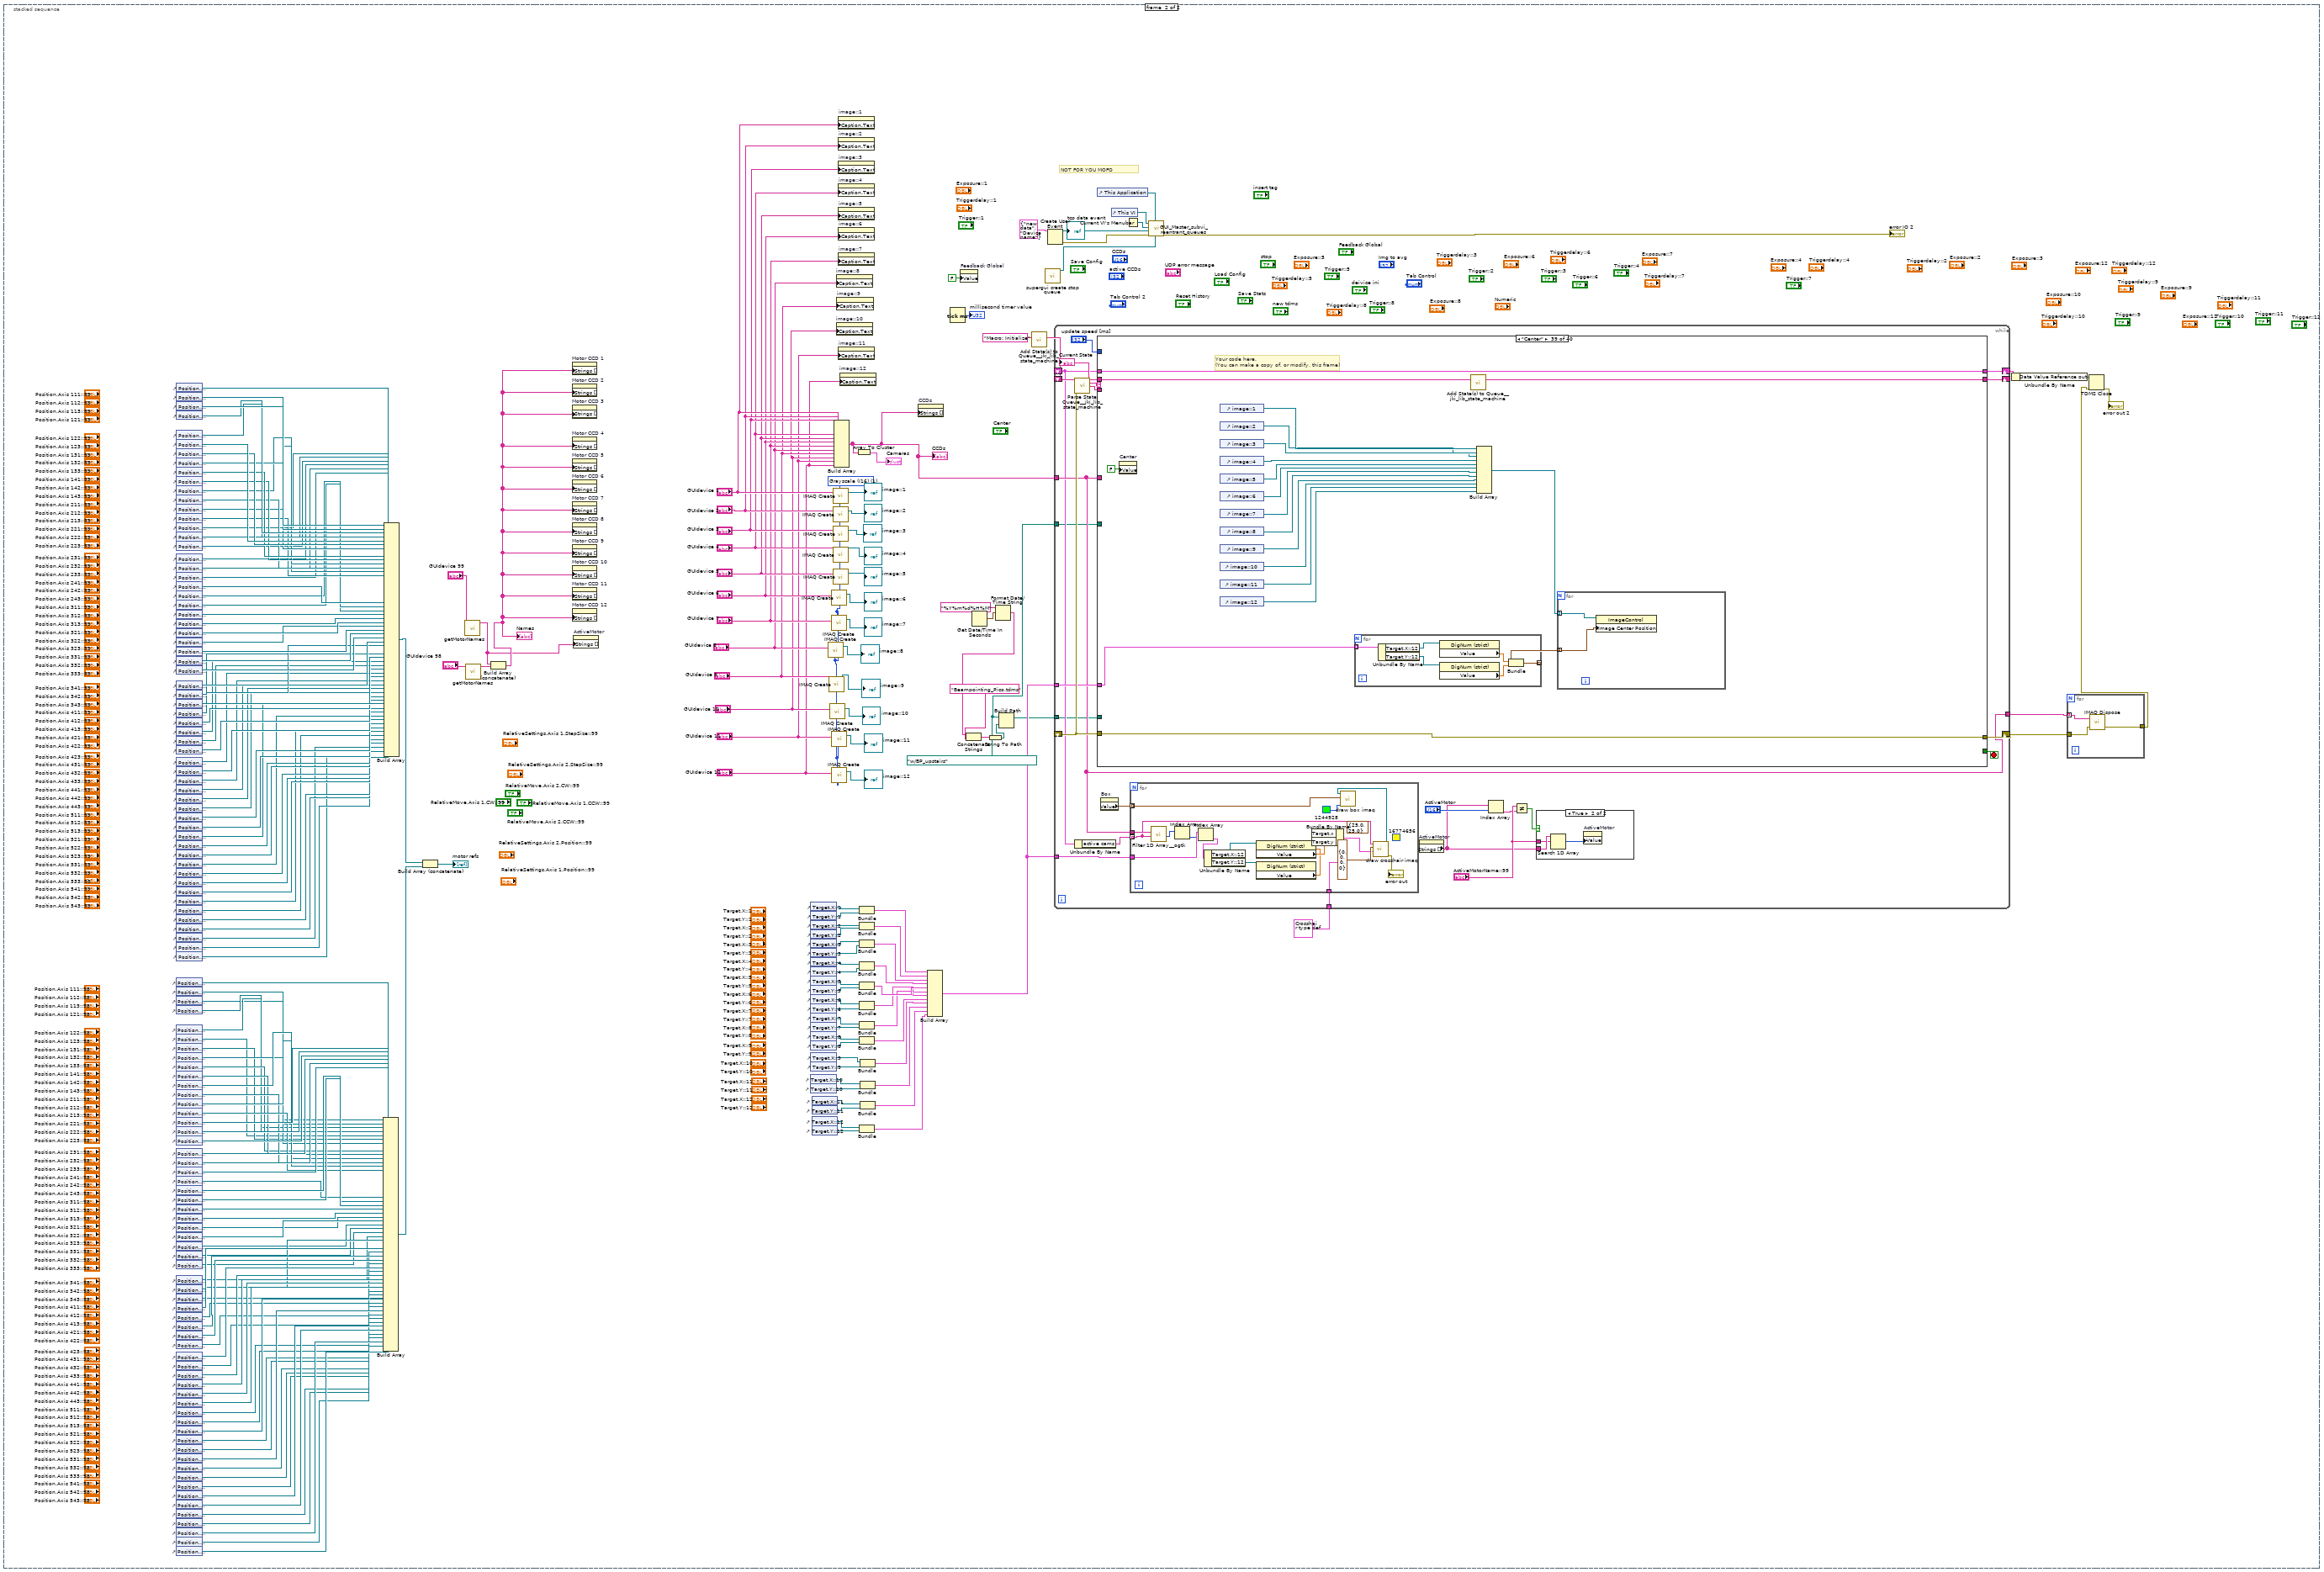
[diagram p2: hidden frame]
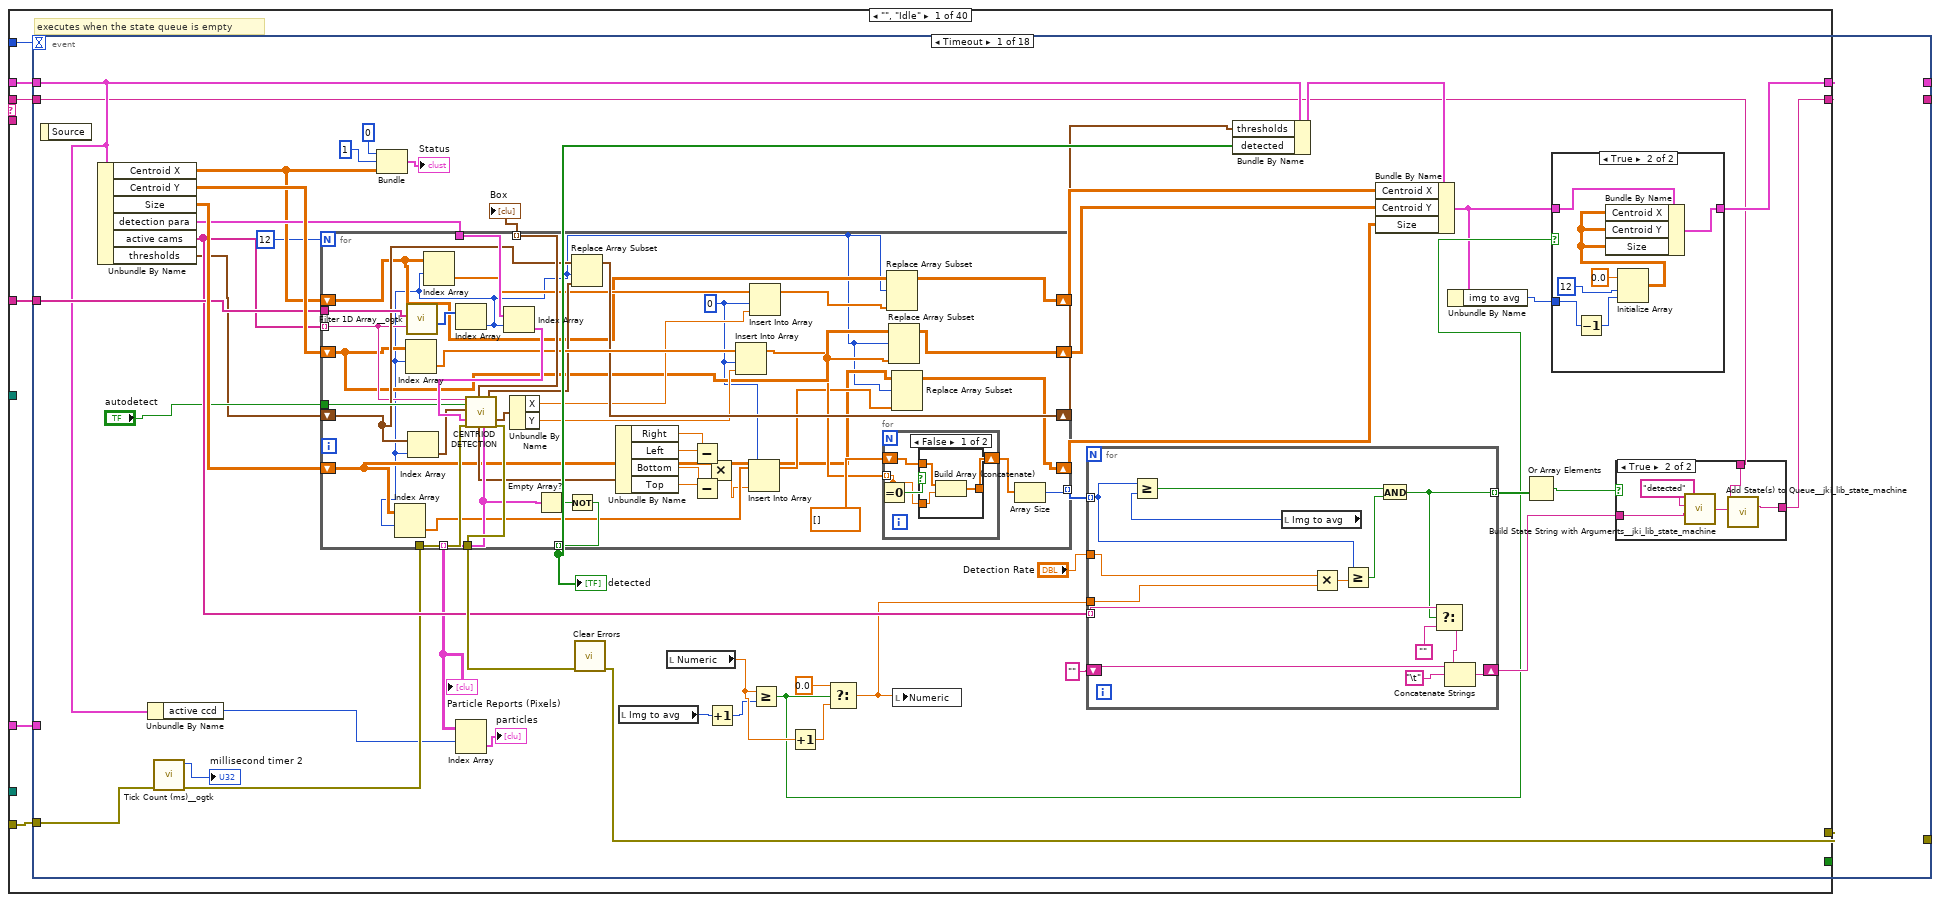
[diagram p4: hidden frame]
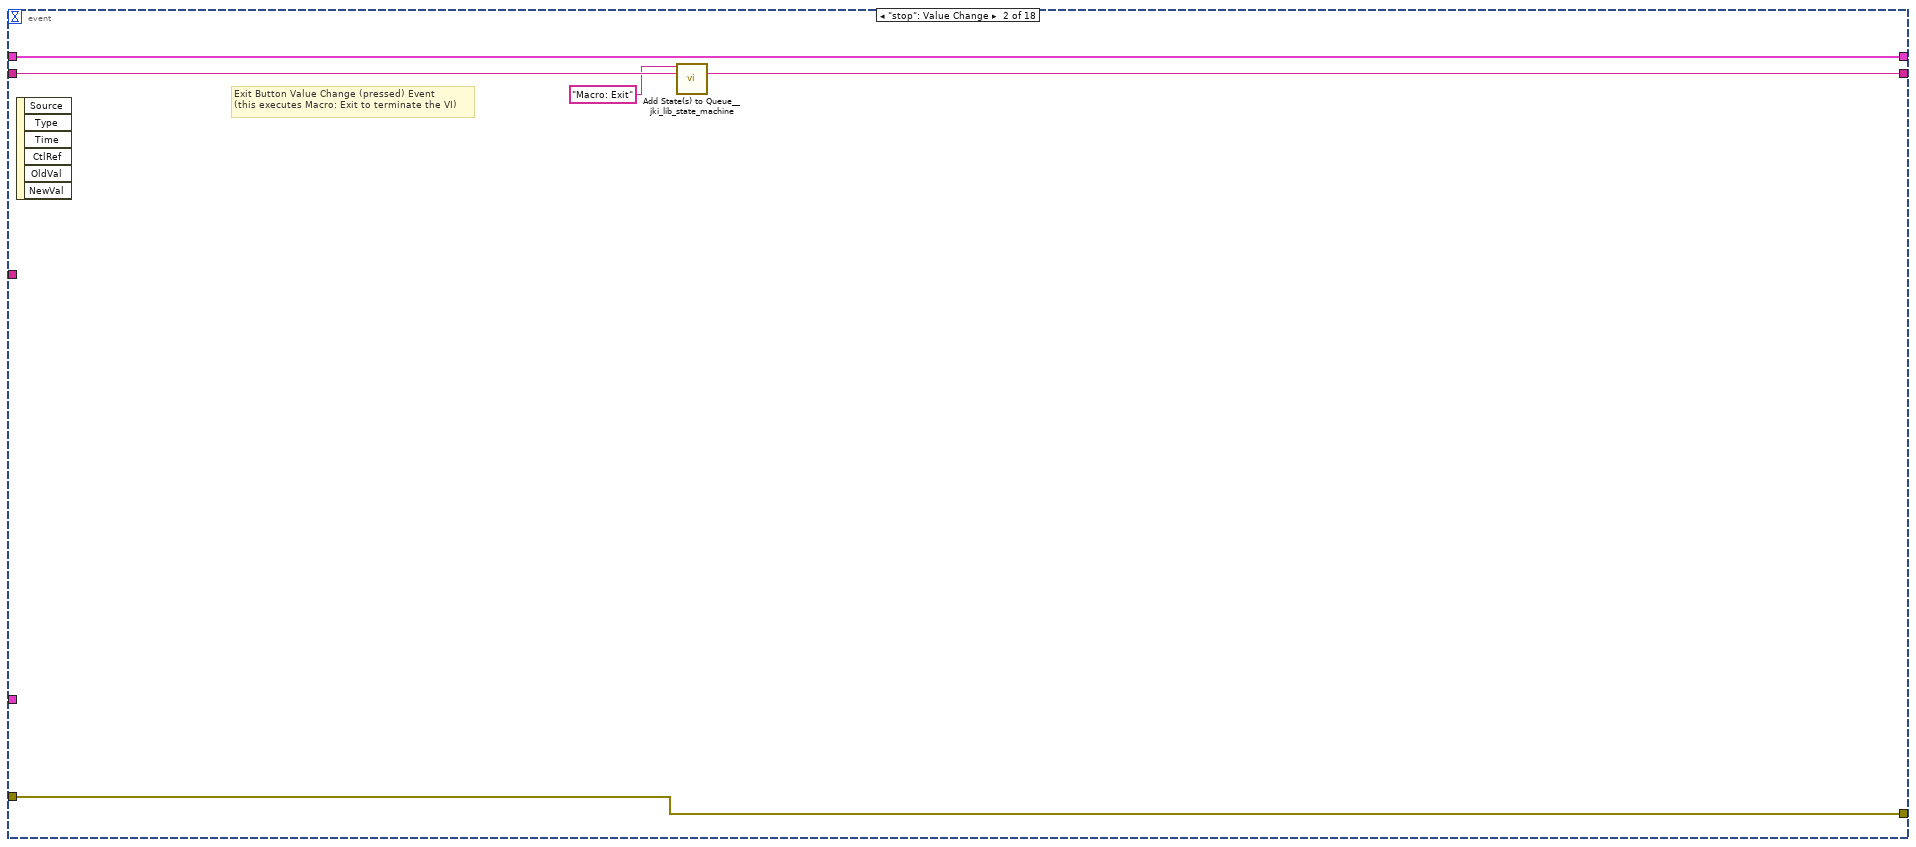
[diagram p8: hidden frame]
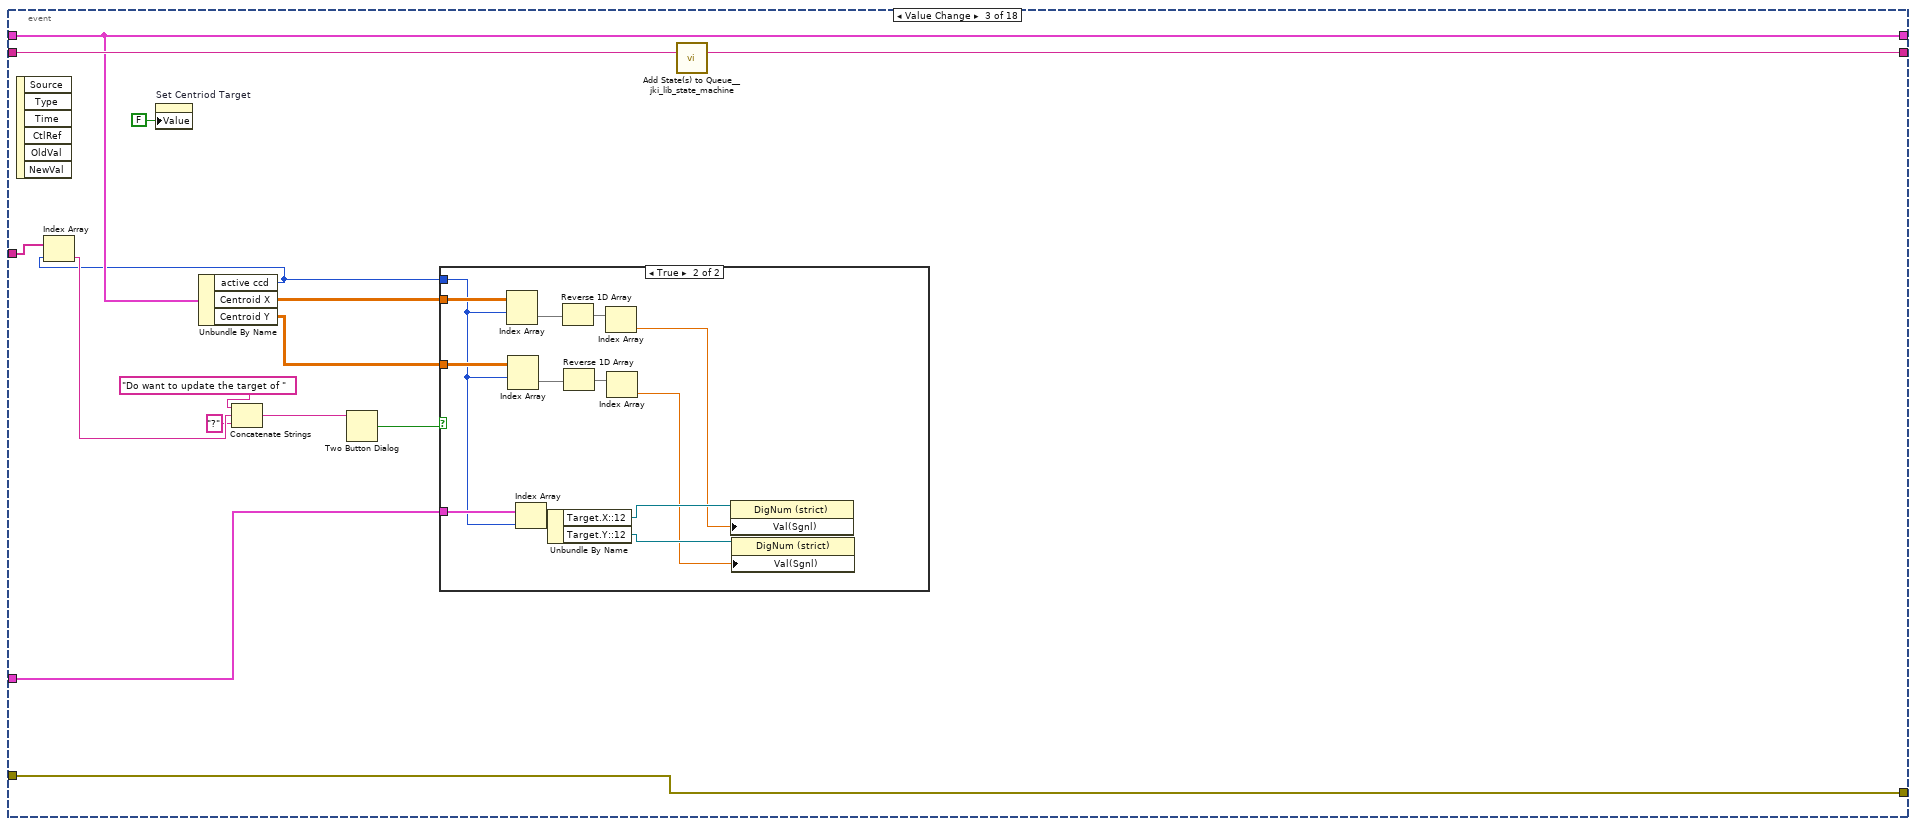
[diagram p9: hidden frame]
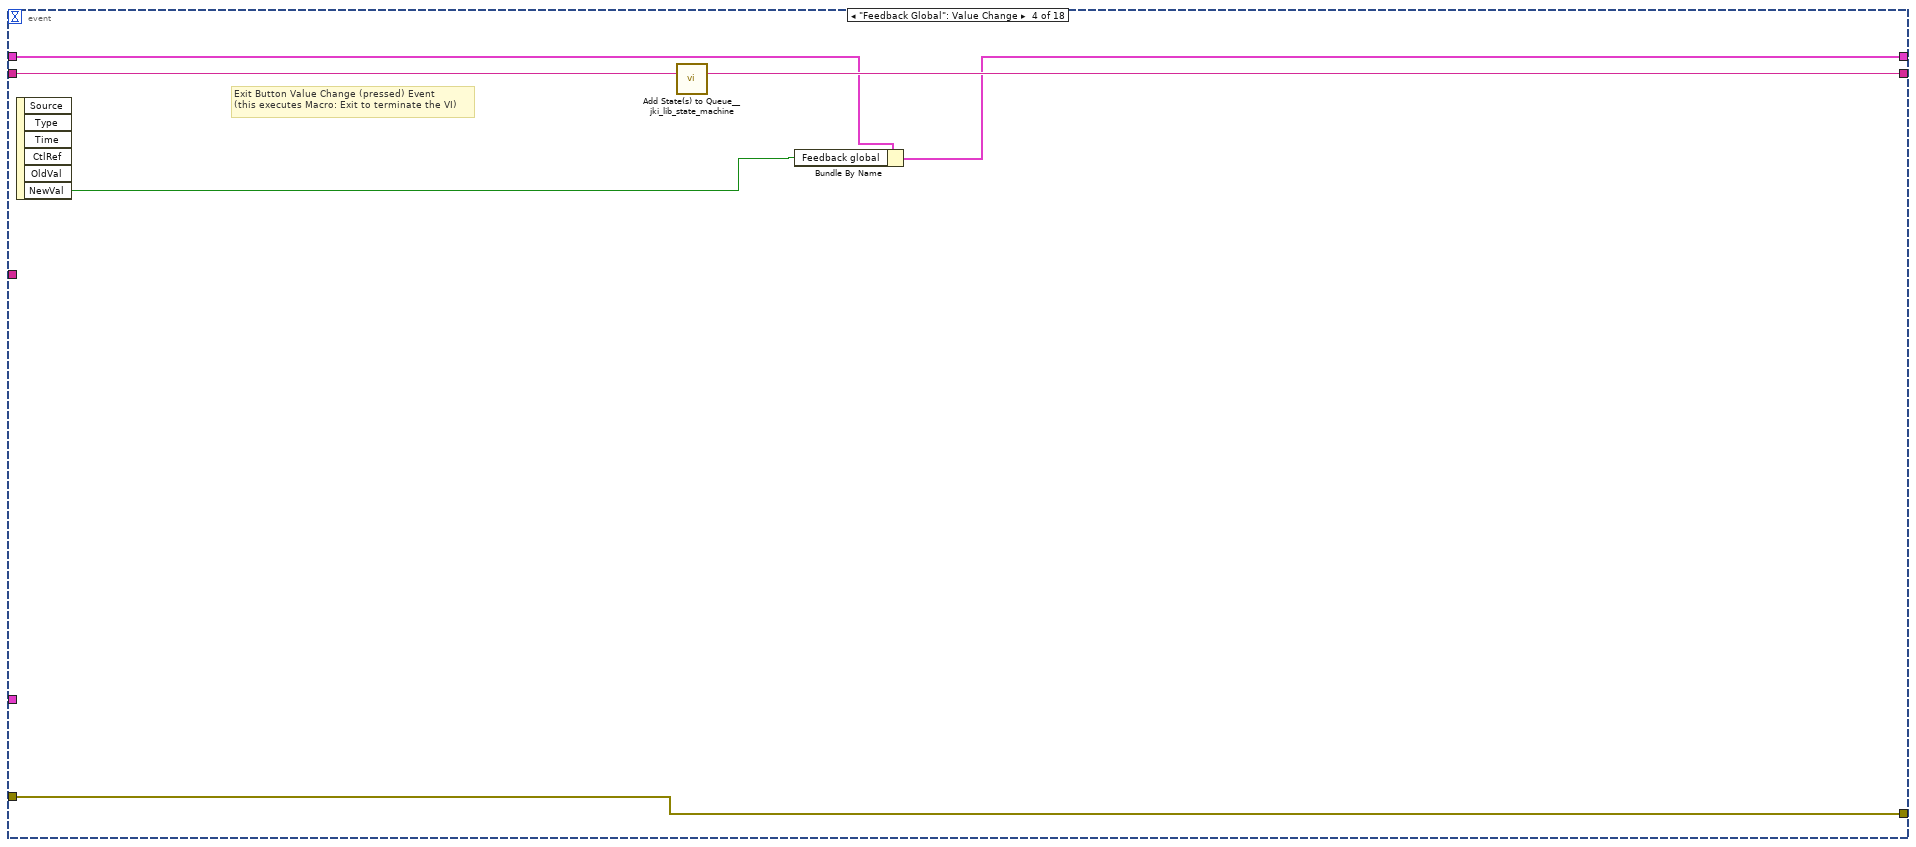
[diagram p11: hidden frame]
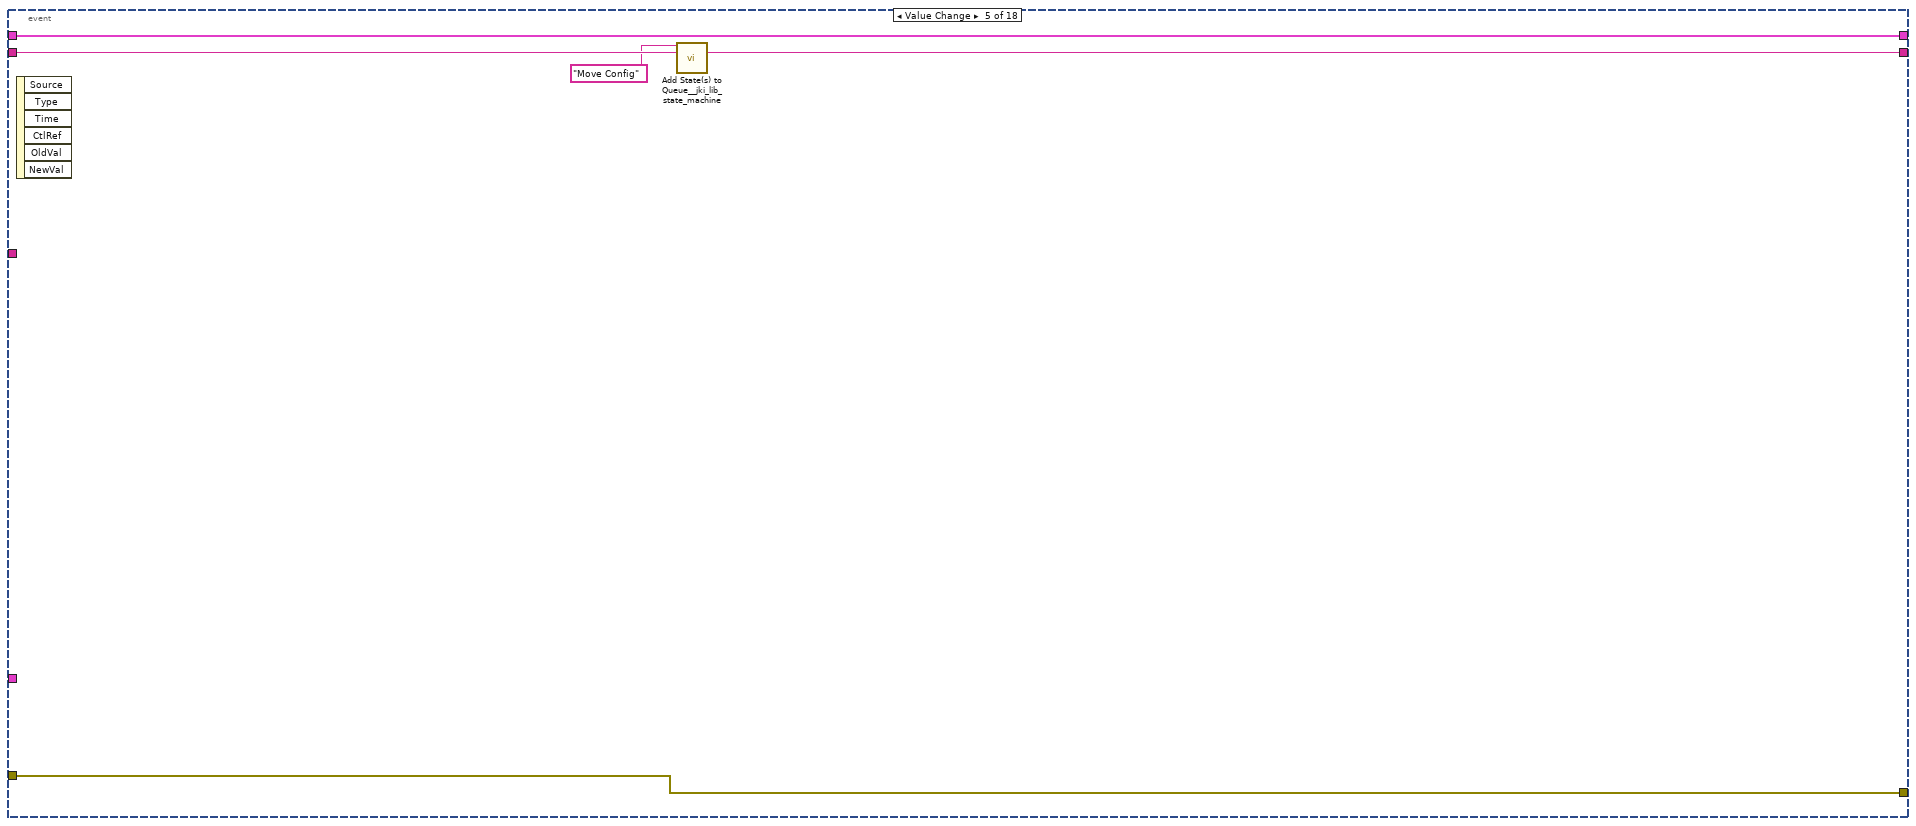
[diagram p12: hidden frame]
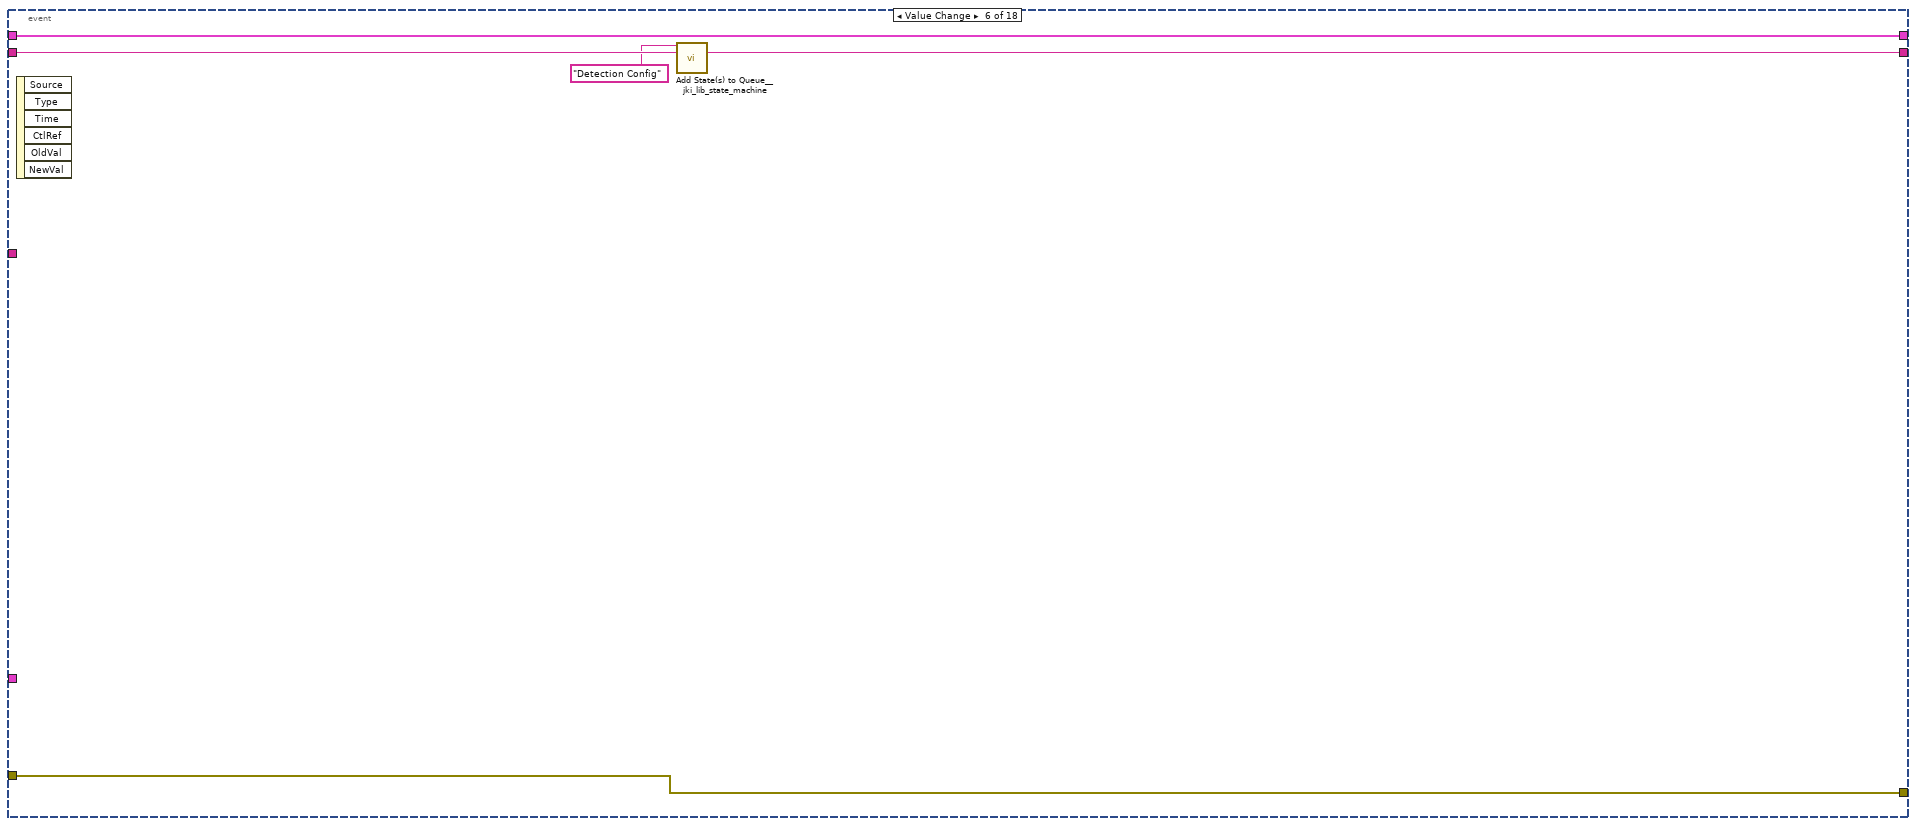
[diagram p13: hidden frame]
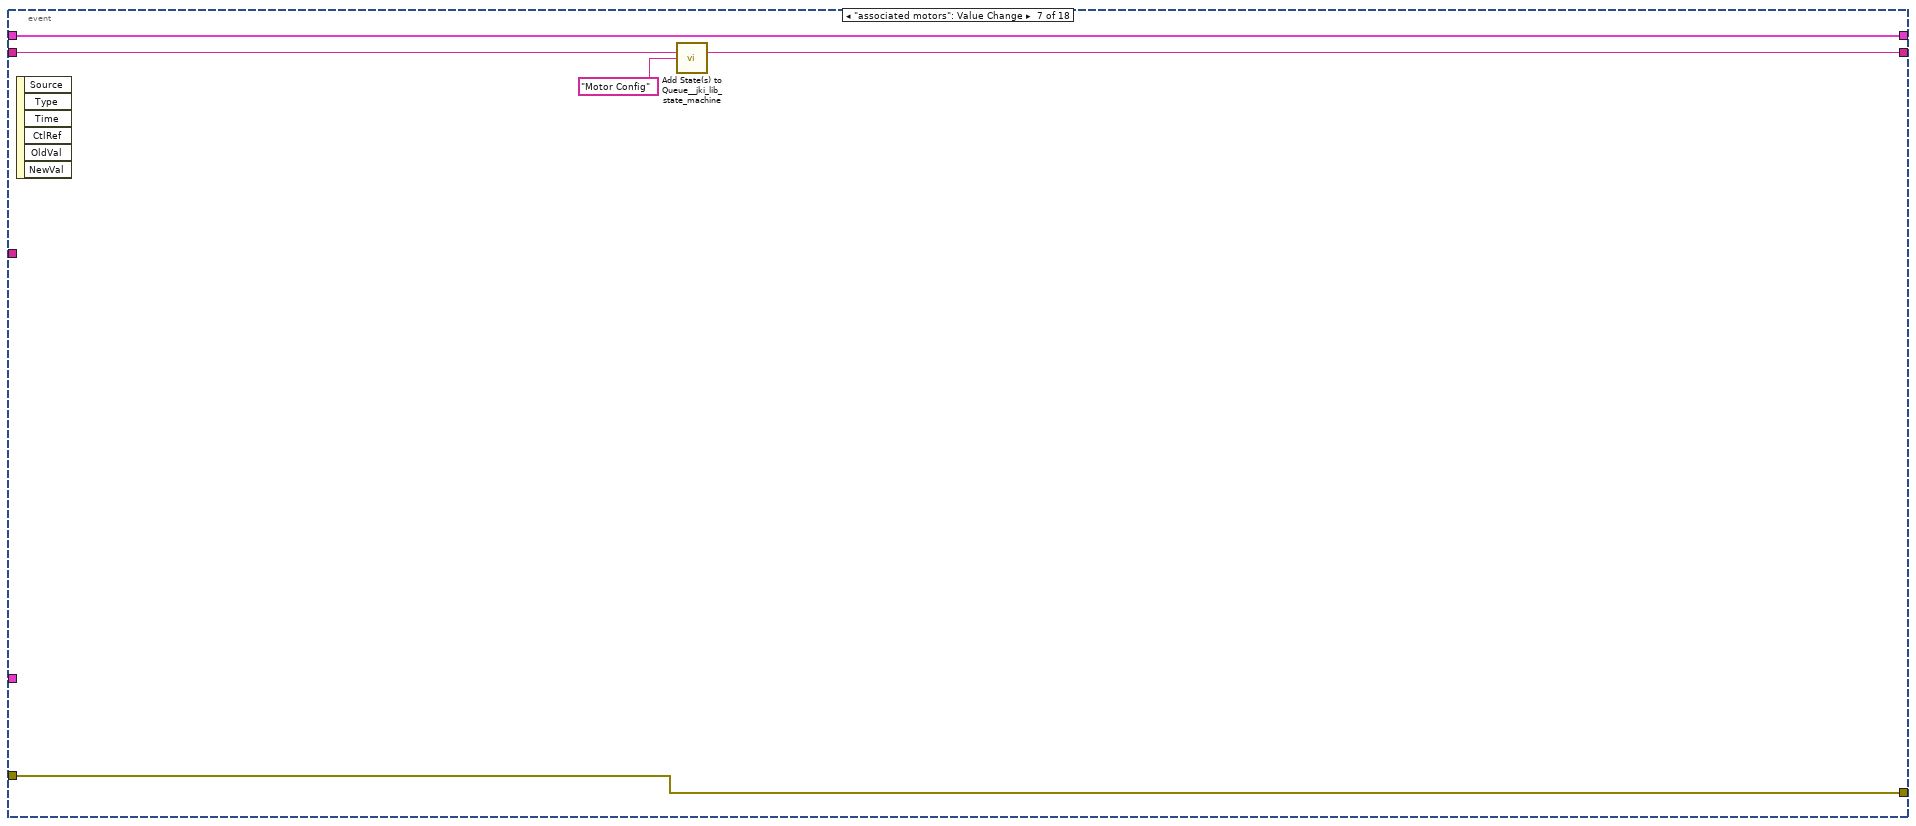
[diagram p14: hidden frame]
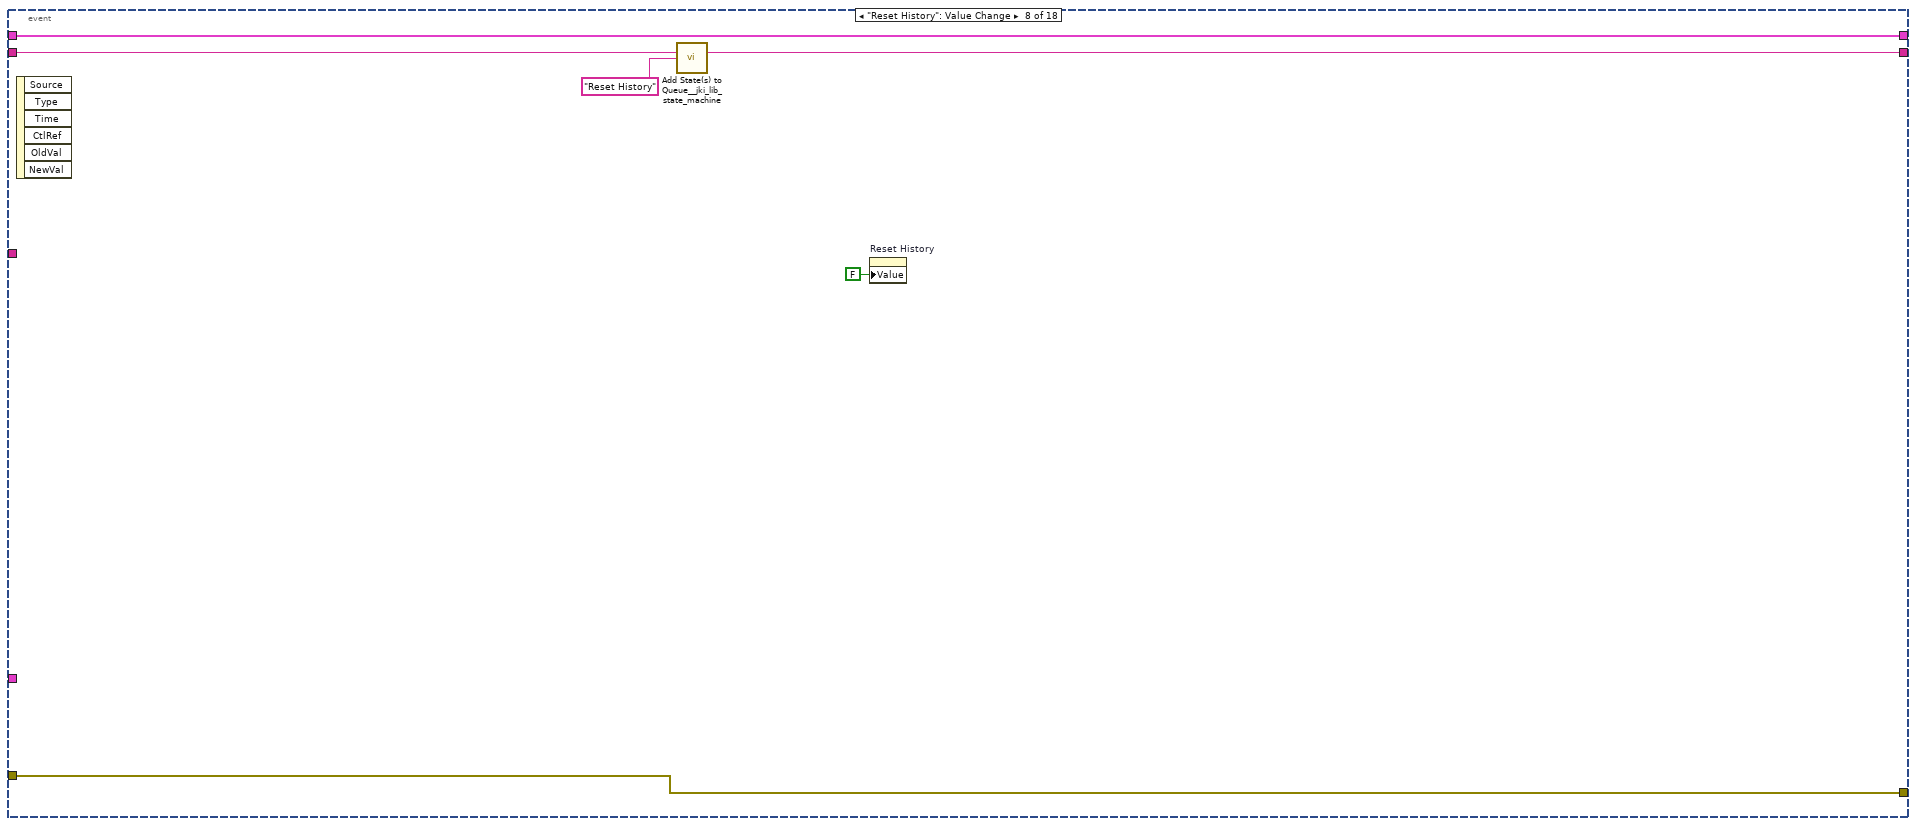
[diagram p15: hidden frame]
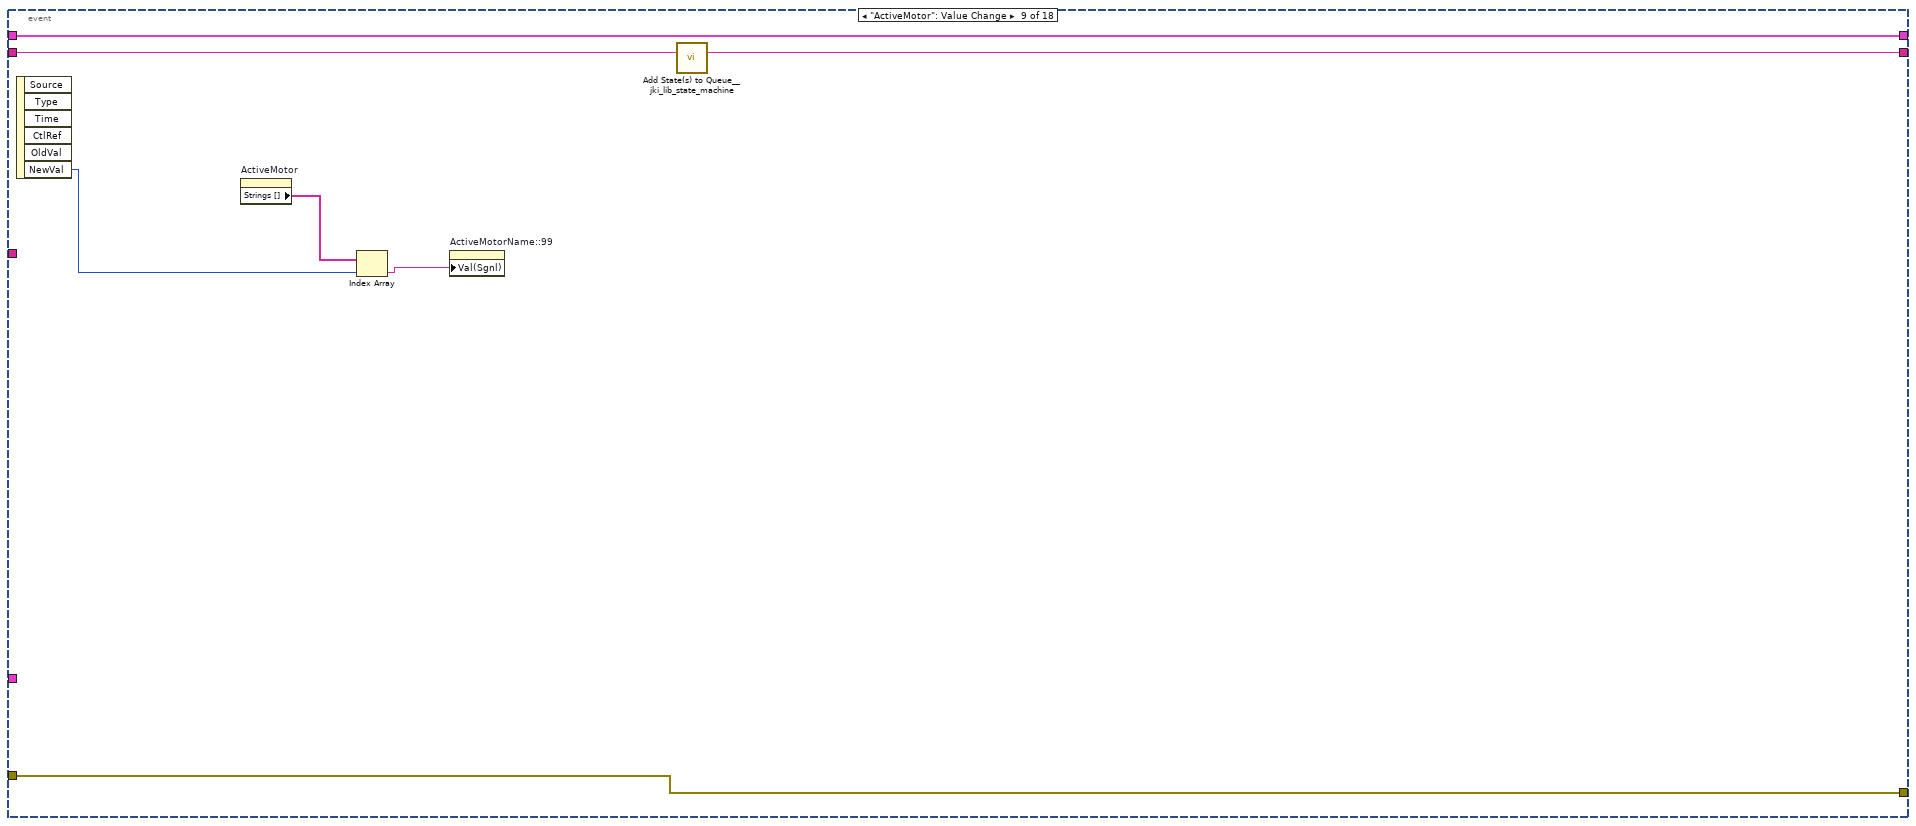
[diagram p16: hidden frame]
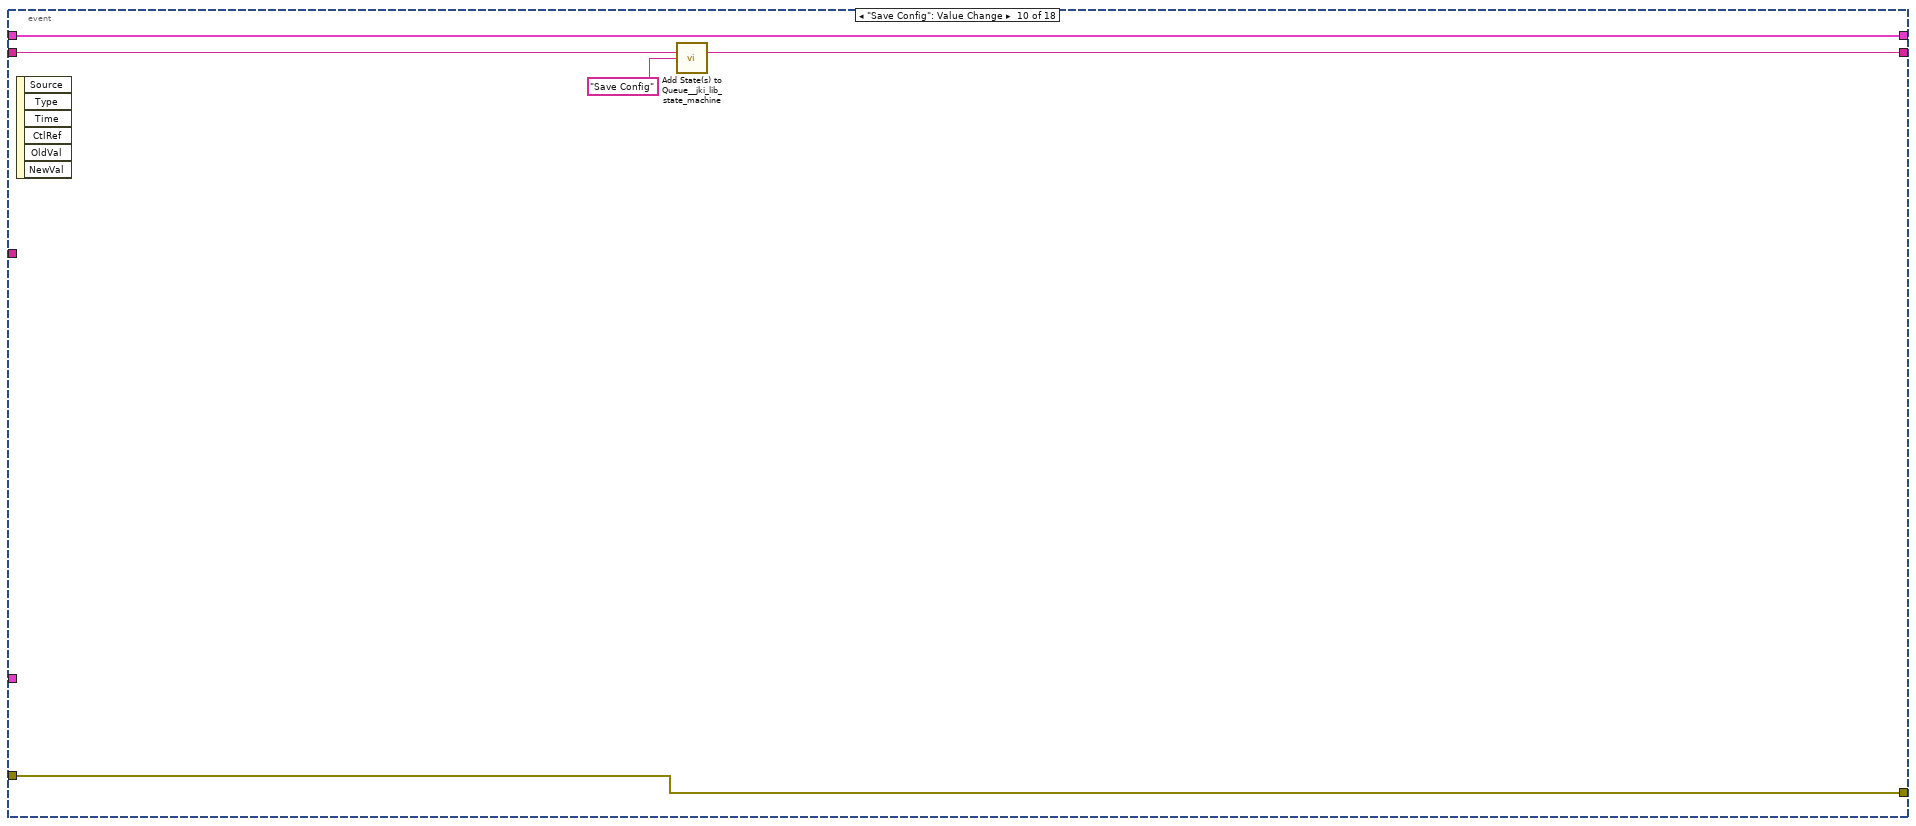
[diagram p17: hidden frame]
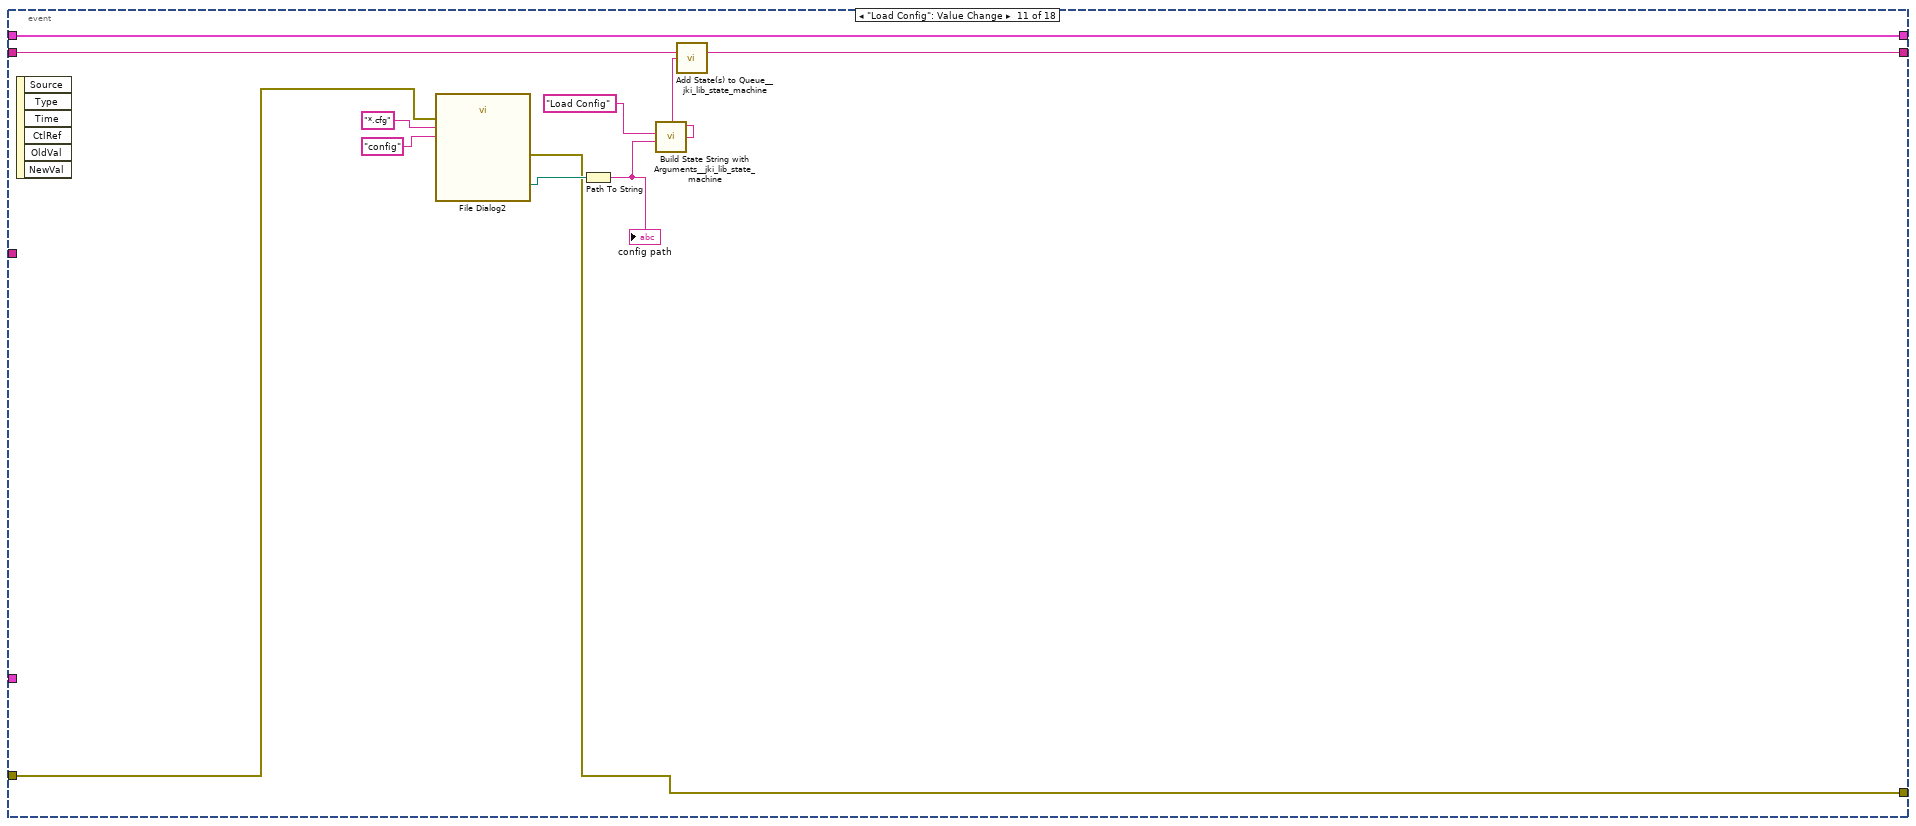
[diagram p18: hidden frame]
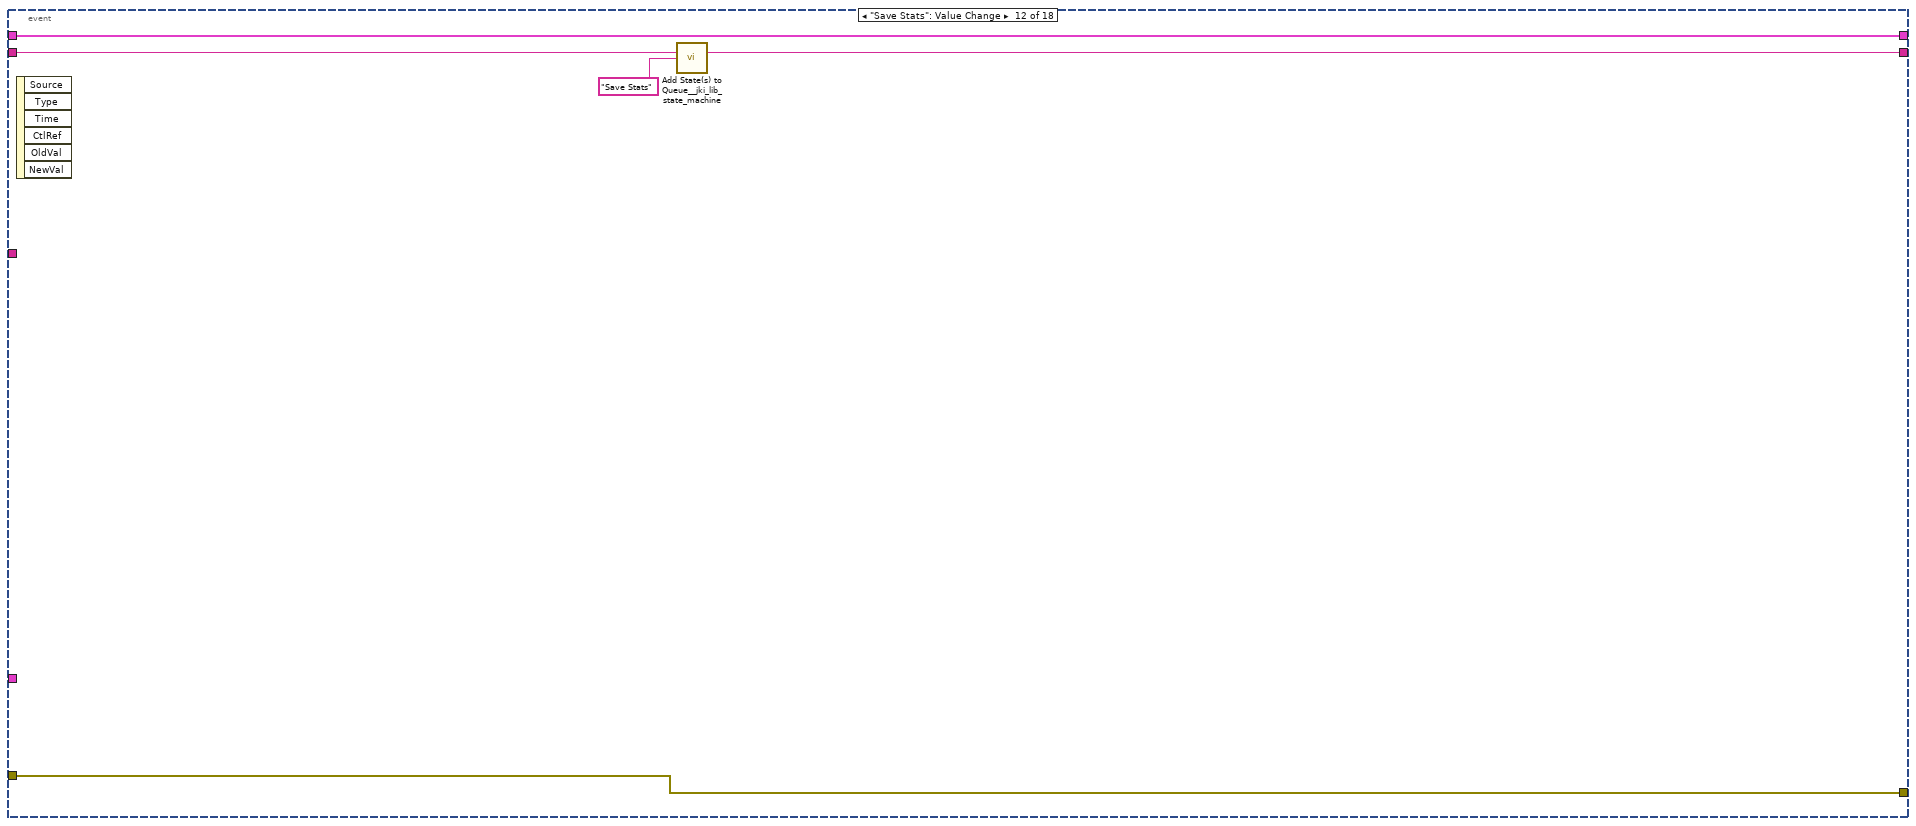
[diagram p19: hidden frame]
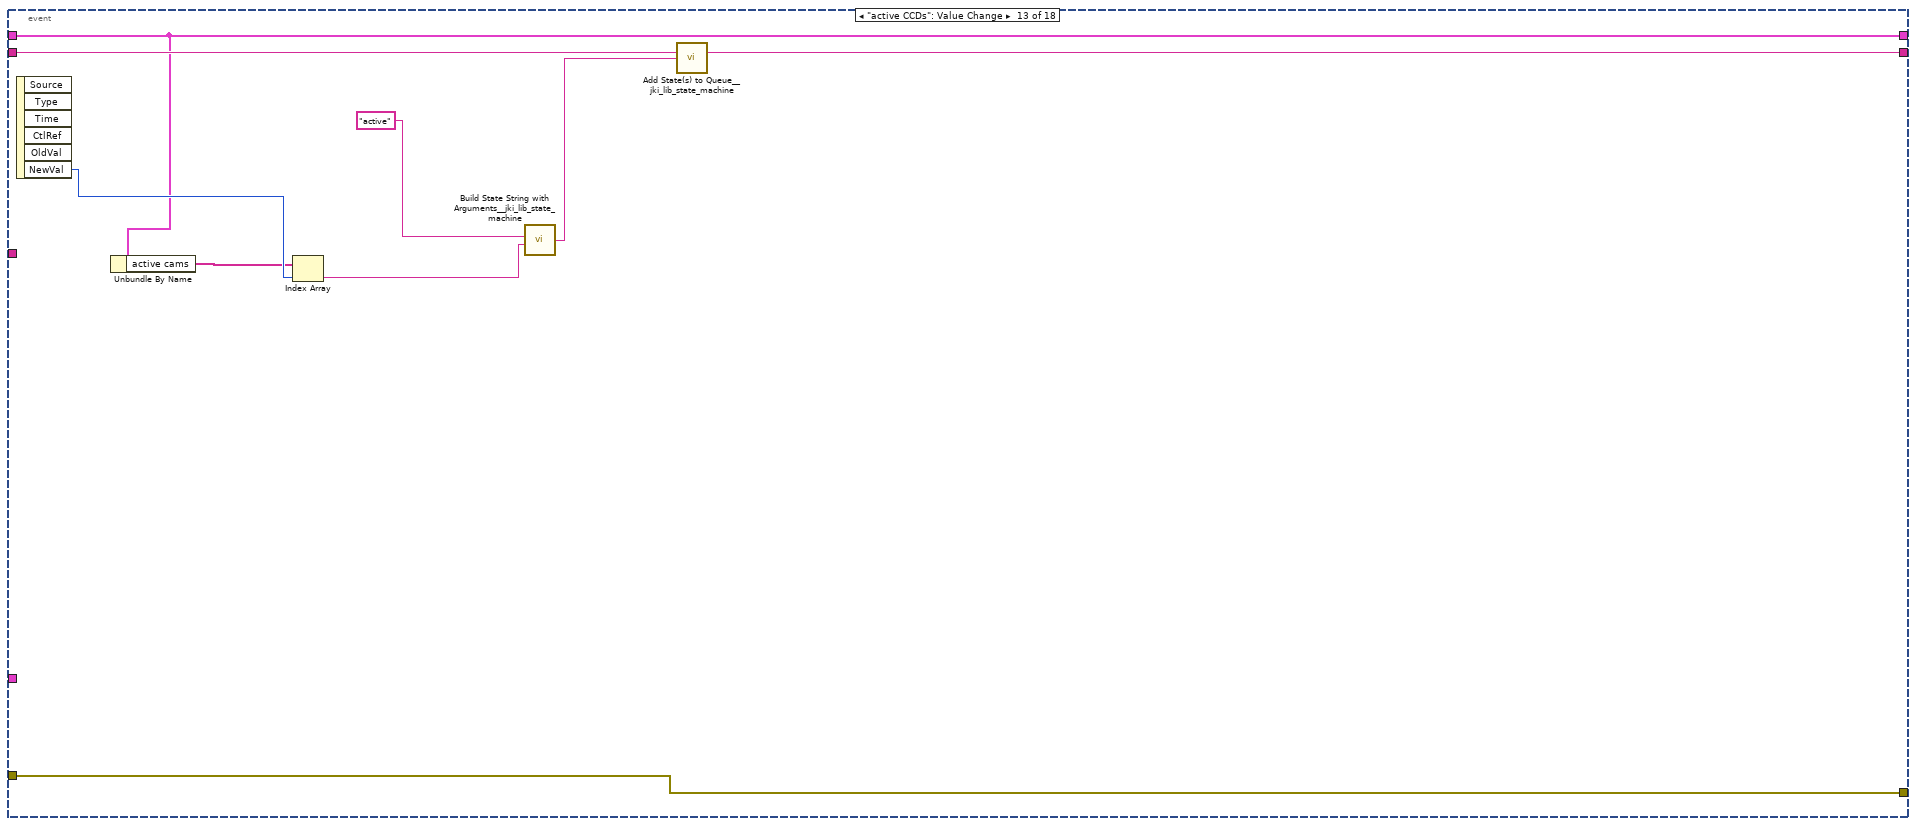
[diagram p20: hidden frame]
diagram:
  n1 = stacked-sequence {
    frame #0 {
      n2 = call <vilib>:"Application Directory.vi"() -> ("Application Directory"=w13:path)
      n3 = Build Path(base path=w13, name or relative path="defaultDevices_UPSTAIRS.txt") -> (appended path=w15:path)
      "appended path" <- w15
      n4 = call-poly <vilib>:"Read From Spreadsheet File.vi"("file path (dialog if empty)"=w15) -> ("all rows"=w16:string[][])  [unwired: 6 in, 4 out]
      n5 = Index Array(array=w16, index (col) #1=0 ("disabled index (col)"), index (col) #2=1 ("index (col)")) -> (element #1=w19:string[])  [unwired: 2 in, 1 out]
      n6 = Index Array(array=w19, index #1=0 ("index"), index #2=1 ("index"), index #3=2 ("index"), index #4=3 ("index"), index #5=4 ("index"), index #6=5 ("index"), index #7=6 ("index"), index #8=7 ("index"), index #9=8 ("index"), index #10=9 ("index"), index #11=10 ("index"), index #12=11 ("index")) -> (element #1=w12:string, element #2=w11:string, element #3=w10:string, element #4=w9:string, element #5=w8:string, element #6=w7:string, element #7=w6:string, element #8=w5:string, element #9=w4:string, element #10=w3:string, element #11=w2:string, element #12=w1:string)
      n7 = property on="GUIdevice 1" class="Str"("Val(Sgnl)"=w12) -> ()  [unwired: 2 in, 2 out]
      n8 = property on="GUIdevice 2" class="Str"("Val(Sgnl)"=w11) -> ()  [unwired: 2 in, 2 out]
      n9 = property on="GUIdevice 3" class="Str"("Val(Sgnl)"=w10) -> ()  [unwired: 2 in, 2 out]
      n10 = property on="GUIdevice 4" class="Str"("Val(Sgnl)"=w9) -> ()  [unwired: 2 in, 2 out]
      n11 = property on="GUIdevice 5" class="Str"("Val(Sgnl)"=w8) -> ()  [unwired: 2 in, 2 out]
      n12 = property on="GUIdevice 6" class="Str"("Val(Sgnl)"=w7) -> ()  [unwired: 2 in, 2 out]
      n13 = property on="GUIdevice 7" class="Str"("Val(Sgnl)"=w6) -> ()  [unwired: 2 in, 2 out]
      n14 = property on="GUIdevice 8" class="Str"("Val(Sgnl)"=w5) -> ()  [unwired: 2 in, 2 out]
      n15 = property on="GUIdevice 9" class="Str"("Val(Sgnl)"=w4) -> ()  [unwired: 2 in, 2 out]
      n16 = property on="GUIdevice 10" class="Str"("Val(Sgnl)"=w3) -> ()  [unwired: 2 in, 2 out]
      n17 = property on="GUIdevice 11" class="Str"("Val(Sgnl)"=w2) -> ()  [unwired: 2 in, 2 out]
      n18 = property on="GUIdevice 12" class="Str"("Val(Sgnl)"=w1) -> ()  [unwired: 2 in, 2 out]
    }
    frame #1 {
      w34 = path "w:/BP_upstairs" ("base path")
      w106 = T21 1 items=["Grayscale (U8)", "Grayscale (I16)", "Grayscale (SGL)", "Complex (CSG)", "RGB (U32)", "HSL (U32)", "RGB (U64)", "Grayscale (U16)"] ("Image Type")
      # "NOT FOR YOU MOFO"
      n19 = control-ref of="Position.Axis 111::98"() -> (w43:refnum<vi>)
      n20 = control-ref of="Position.Axis 112::98"() -> (w44:refnum<vi>)
      n21 = control-ref of="Position.Axis 113::98"() -> (w45:refnum<vi>)
      n22 = control-ref of="Position.Axis 121::98"() -> (w46:refnum<vi>)
      n23 = control-ref of="Position.Axis 122::98"() -> (w47:refnum<vi>)
      n24 = control-ref of="Position.Axis 123::98"() -> (w48:refnum<vi>)
      n25 = control-ref of="Position.Axis 131::98"() -> (w49:refnum<vi>)
      n26 = control-ref of="Position.Axis 132::98"() -> (w50:refnum<vi>)
      n27 = control-ref of="Position.Axis 133::98"() -> (w51:refnum<vi>)
      n28 = control-ref of="Position.Axis 141::98"() -> (w52:refnum<vi>)
      n29 = control-ref of="Position.Axis 142::98"() -> (w53:refnum<vi>)
      n30 = control-ref of="Position.Axis 143::98"() -> (w54:refnum<vi>)
      n31 = control-ref of="Position.Axis 211::98"() -> (w55:refnum<vi>)
      n32 = control-ref of="Position.Axis 212::98"() -> (w56:refnum<vi>)
      n33 = control-ref of="Position.Axis 213::98"() -> (w57:refnum<vi>)
      n34 = control-ref of="Position.Axis 221::98"() -> (w58:refnum<vi>)
      n35 = control-ref of="Position.Axis 222::98"() -> (w59:refnum<vi>)
      n36 = control-ref of="Position.Axis 223::98"() -> (w60:refnum<vi>)
      n37 = control-ref of="Position.Axis 231::98"() -> (w61:refnum<vi>)
      n38 = control-ref of="Position.Axis 232::98"() -> (w62:refnum<vi>)
      n39 = control-ref of="Position.Axis 233::98"() -> (w63:refnum<vi>)
      n40 = control-ref of="Position.Axis 241::98"() -> (w64:refnum<vi>)
      n41 = control-ref of="Position.Axis 242::98"() -> (w65:refnum<vi>)
      n42 = control-ref of="Position.Axis 243::98"() -> (w66:refnum<vi>)
      n43 = control-ref of="Position.Axis 311::98"() -> (w67:refnum<vi>)
      n44 = control-ref of="Position.Axis 312::98"() -> (w68:refnum<vi>)
      n45 = control-ref of="Position.Axis 313::98"() -> (w69:refnum<vi>)
      n46 = control-ref of="Position.Axis 321::98"() -> (w70:refnum<vi>)
      n47 = control-ref of="Position.Axis 322::98"() -> (w71:refnum<vi>)
      n48 = control-ref of="Position.Axis 323::98"() -> (w72:refnum<vi>)
      n49 = control-ref of="Position.Axis 331::98"() -> (w73:refnum<vi>)
      n50 = control-ref of="Position.Axis 332::98"() -> (w74:refnum<vi>)
      n51 = control-ref of="Position.Axis 333::98"() -> (w75:refnum<vi>)
      n52 = control-ref of="Position.Axis 341::98"() -> (w76:refnum<vi>)
      n53 = control-ref of="Position.Axis 342::98"() -> (w77:refnum<vi>)
      n54 = control-ref of="Position.Axis 343::98"() -> (w78:refnum<vi>)
      n55 = control-ref of="Position.Axis 411::98"() -> (w79:refnum<vi>)
      n56 = control-ref of="Position.Axis 412::98"() -> (w80:refnum<vi>)
      n57 = control-ref of="Position.Axis 413::98"() -> (w81:refnum<vi>)
      n58 = control-ref of="Position.Axis 421::98"() -> (w82:refnum<vi>)
      n59 = control-ref of="Position.Axis 422::98"() -> (w83:refnum<vi>)
      n60 = control-ref of="Position.Axis 423::98"() -> (w84:refnum<vi>)
      n61 = control-ref of="Position.Axis 431::98"() -> (w85:refnum<vi>)
      n62 = control-ref of="Position.Axis 432::98"() -> (w86:refnum<vi>)
      n63 = control-ref of="Position.Axis 433::98"() -> (w87:refnum<vi>)
      n64 = control-ref of="Position.Axis 441::98"() -> (w88:refnum<vi>)
      n65 = control-ref of="Position.Axis 442::98"() -> (w89:refnum<vi>)
      n66 = control-ref of="Position.Axis 443::98"() -> (w90:refnum<vi>)
      n67 = control-ref of="Position.Axis 511::98"() -> (w91:refnum<vi>)
      n68 = control-ref of="Position.Axis 512::98"() -> (w92:refnum<vi>)
      n69 = control-ref of="Position.Axis 513::98"() -> (w93:refnum<vi>)
      n70 = control-ref of="Position.Axis 521::98"() -> (w94:refnum<vi>)
      n71 = control-ref of="Position.Axis 522::98"() -> (w95:refnum<vi>)
      n72 = control-ref of="Position.Axis 523::98"() -> (w96:refnum<vi>)
      n73 = control-ref of="Position.Axis 531::98"() -> (w97:refnum<vi>)
      n74 = control-ref of="Position.Axis 532::98"() -> (w98:refnum<vi>)
      n75 = control-ref of="Position.Axis 533::98"() -> (w99:refnum<vi>)
      n76 = control-ref of="Position.Axis 541::98"() -> (w100:refnum<vi>)
      n77 = control-ref of="Position.Axis 542::98"() -> (w101:refnum<vi>)
      n78 = control-ref of="Position.Axis 543::98"() -> (w102:refnum<vi>)
      n79 = control-ref of="Position.Axis 111::99"() -> (w234:refnum<vi>)
      n80 = control-ref of="Position.Axis 112::99"() -> (w233:refnum<vi>)
      n81 = control-ref of="Position.Axis 113::99"() -> (w232:refnum<vi>)
      n82 = control-ref of="Position.Axis 121::99"() -> (w231:refnum<vi>)
      n83 = control-ref of="Position.Axis 122::99"() -> (w230:refnum<vi>)
      n84 = control-ref of="Position.Axis 123::99"() -> (w229:refnum<vi>)
      n85 = control-ref of="Position.Axis 131::99"() -> (w228:refnum<vi>)
      n86 = control-ref of="Position.Axis 132::99"() -> (w227:refnum<vi>)
      n87 = control-ref of="Position.Axis 133::99"() -> (w226:refnum<vi>)
      n88 = control-ref of="Position.Axis 141::99"() -> (w225:refnum<vi>)
      n89 = control-ref of="Position.Axis 142::99"() -> (w224:refnum<vi>)
      n90 = control-ref of="Position.Axis 143::99"() -> (w223:refnum<vi>)
      n91 = control-ref of="Position.Axis 211::99"() -> (w222:refnum<vi>)
      n92 = control-ref of="Position.Axis 212::99"() -> (w221:refnum<vi>)
      n93 = control-ref of="Position.Axis 213::99"() -> (w220:refnum<vi>)
      n94 = control-ref of="Position.Axis 221::99"() -> (w219:refnum<vi>)
      n95 = control-ref of="Position.Axis 222::99"() -> (w218:refnum<vi>)
      n96 = control-ref of="Position.Axis 223::99"() -> (w217:refnum<vi>)
      n97 = control-ref of="Position.Axis 231::99"() -> (w216:refnum<vi>)
      n98 = control-ref of="Position.Axis 232::99"() -> (w215:refnum<vi>)
      n99 = control-ref of="Position.Axis 233::99"() -> (w214:refnum<vi>)
      n100 = control-ref of="Position.Axis 241::99"() -> (w213:refnum<vi>)
      n101 = control-ref of="Position.Axis 242::99"() -> (w212:refnum<vi>)
      n102 = control-ref of="Position.Axis 243::99"() -> (w211:refnum<vi>)
      n103 = control-ref of="Position.Axis 311::99"() -> (w210:refnum<vi>)
      n104 = control-ref of="Position.Axis 312::99"() -> (w209:refnum<vi>)
      n105 = control-ref of="Position.Axis 313::99"() -> (w208:refnum<vi>)
      n106 = control-ref of="Position.Axis 321::99"() -> (w207:refnum<vi>)
      n107 = control-ref of="Position.Axis 322::99"() -> (w206:refnum<vi>)
      n108 = control-ref of="Position.Axis 323::99"() -> (w205:refnum<vi>)
      n109 = control-ref of="Position.Axis 331::99"() -> (w204:refnum<vi>)
      n110 = control-ref of="Position.Axis 332::99"() -> (w203:refnum<vi>)
      n111 = control-ref of="Position.Axis 333::99"() -> (w202:refnum<vi>)
      n112 = control-ref of="Position.Axis 341::99"() -> (w201:refnum<vi>)
      n113 = control-ref of="Position.Axis 342::99"() -> (w200:refnum<vi>)
      n114 = control-ref of="Position.Axis 343::99"() -> (w199:refnum<vi>)
      n115 = control-ref of="Position.Axis 411::99"() -> (w198:refnum<vi>)
      n116 = control-ref of="Position.Axis 412::99"() -> (w197:refnum<vi>)
      n117 = control-ref of="Position.Axis 413::99"() -> (w196:refnum<vi>)
      n118 = control-ref of="Position.Axis 421::99"() -> (w195:refnum<vi>)
      n119 = control-ref of="Position.Axis 422::99"() -> (w194:refnum<vi>)
      n120 = control-ref of="Position.Axis 423::99"() -> (w193:refnum<vi>)
      n121 = control-ref of="Position.Axis 431::99"() -> (w192:refnum<vi>)
      n122 = control-ref of="Position.Axis 432::99"() -> (w191:refnum<vi>)
      n123 = control-ref of="Position.Axis 433::99"() -> (w190:refnum<vi>)
      n124 = control-ref of="Position.Axis 441::99"() -> (w189:refnum<vi>)
      n125 = control-ref of="Position.Axis 442::99"() -> (w188:refnum<vi>)
      n126 = control-ref of="Position.Axis 443::99"() -> (w187:refnum<vi>)
      n127 = control-ref of="Position.Axis 511::99"() -> (w186:refnum<vi>)
      n128 = control-ref of="Position.Axis 512::99"() -> (w185:refnum<vi>)
      n129 = control-ref of="Position.Axis 513::99"() -> (w184:refnum<vi>)
      n130 = control-ref of="Position.Axis 521::99"() -> (w183:refnum<vi>)
      n131 = control-ref of="Position.Axis 522::99"() -> (w182:refnum<vi>)
      n132 = control-ref of="Position.Axis 523::99"() -> (w181:refnum<vi>)
      n133 = control-ref of="Position.Axis 531::99"() -> (w180:refnum<vi>)
      n134 = control-ref of="Position.Axis 532::99"() -> (w179:refnum<vi>)
      n135 = control-ref of="Position.Axis 533::99"() -> (w178:refnum<vi>)
      n136 = control-ref of="Position.Axis 541::99"() -> (w177:refnum<vi>)
      n137 = control-ref of="Position.Axis 542::99"() -> (w176:refnum<vi>)
      n138 = control-ref of="Position.Axis 543::99"() -> (w175:refnum<vi>)
      n139 = Build Array(w43, w44, w45, w46, w47, w48, w49, w50, w51, w52, w53, w54, w55, w56, w57, w58, w59, w60, w61, w62, w63, w64, w65, w66, w67, w68, w69, w70, w71, w72, w73, w74, w75, w76, w77, w78, w79, w80, w81, w82, w83, w84, w85, w86, w87, w88, w89, w90, w91, w92, w93, w94, w95, w96, w97, w98, w99, w100, w101, w102) -> (w40:refnum<vi>[])
      n140 = Build Array(w234, w233, w232, w231, w230, w229, w228, w227, w226, w225, w224, w223, w222, w221, w220, w219, w218, w217, w216, w215, w214, w213, w212, w211, w210, w209, w208, w207, w206, w205, w204, w203, w202, w201, w200, w199, w198, w197, w196, w195, w194, w193, w192, w191, w190, w189, w188, w187, w186, w185, w184, w183, w182, w181, w180, w179, w178, w177, w176, w175) -> (w39:refnum<vi>[])
      n141 = Build Array (concatenate)(w39, w40) -> (→"motor refs":refnum<vi>[])
      n142 = call "getMotorNames.vi"("DeviceName"="GUIdevice 99") -> ("elements"=w37:string[])  [unwired: 10 in]
      n143 = call "getMotorNames.vi"("DeviceName"="GUIdevice 98") -> ("elements"=w36:string[])  [unwired: 10 in]
      n144 = Build Array (concatenate)(w37, w36) -> (w41:string[])
      "Names" <- w41
      n145 = property on="Motor CCD 1" class="Ring (strict)"("Strings []"=w41) -> ()  [unwired: 2 in, 2 out]
      n146 = property on="Motor CCD 2" class="Ring (strict)"("Strings []"=w41) -> ()  [unwired: 2 in, 2 out]
      n147 = property on="Motor CCD 3" class="Ring (strict)"("Strings []"=w41) -> ()  [unwired: 2 in, 2 out]
      n148 = property on="Motor CCD 4" class="Ring (strict)"("Strings []"=w41) -> ()  [unwired: 2 in, 2 out]
      n149 = property on="Motor CCD 5" class="Ring (strict)"("Strings []"=w41) -> ()  [unwired: 2 in, 2 out]
      n150 = property on="Motor CCD 6" class="Ring (strict)"("Strings []"=w41) -> ()  [unwired: 2 in, 2 out]
      n151 = property on="Motor CCD 7" class="Ring (strict)"("Strings []"=w41) -> ()  [unwired: 2 in, 2 out]
      n152 = property on="Motor CCD 8" class="Ring (strict)"("Strings []"=w41) -> ()  [unwired: 2 in, 2 out]
      n153 = property on="Motor CCD 9" class="Ring (strict)"("Strings []"=w41) -> ()  [unwired: 2 in, 2 out]
      n154 = property on="Motor CCD 10" class="Ring (strict)"("Strings []"=w41) -> ()  [unwired: 2 in, 2 out]
      n155 = property on="Motor CCD 11" class="Ring (strict)"("Strings []"=w41) -> ()  [unwired: 2 in, 2 out]
      n156 = property on="Motor CCD 12" class="Ring (strict)"("Strings []"=w41) -> ()  [unwired: 2 in, 2 out]
      n157 = property on="ActiveMotor" class="Ring (strict)"("Strings []"=w37) -> ()  [unwired: 2 in, 2 out]
      n158 = control-ref of="Target.X::1"() -> (w161:refnum<vi>)
      n159 = control-ref of="Target.Y::1"() -> (w160:refnum<vi>)
      n160 = control-ref of="Target.X::2"() -> (w159:refnum<vi>)
      n161 = control-ref of="Target.Y::2"() -> (w158:refnum<vi>)
      n162 = control-ref of="Target.X::3"() -> (w157:refnum<vi>)
      n163 = control-ref of="Target.Y::3"() -> (w156:refnum<vi>)
      n164 = control-ref of="Target.X::4"() -> (w155:refnum<vi>)
      n165 = control-ref of="Target.Y::4"() -> (w154:refnum<vi>)
      n166 = control-ref of="Target.X::5"() -> (w153:refnum<vi>)
      n167 = control-ref of="Target.Y::5"() -> (w152:refnum<vi>)
      n168 = control-ref of="Target.X::6"() -> (w151:refnum<vi>)
      n169 = control-ref of="Target.Y::6"() -> (w150:refnum<vi>)
      n170 = control-ref of="Target.X::7"() -> (w149:refnum<vi>)
      n171 = control-ref of="Target.Y::7"() -> (w148:refnum<vi>)
      n172 = control-ref of="Target.X::8"() -> (w147:refnum<vi>)
      n173 = control-ref of="Target.Y::8"() -> (w146:refnum<vi>)
      n174 = control-ref of="Target.X::9"() -> (w123:refnum<vi>)
      n175 = control-ref of="Target.Y::9"() -> (w122:refnum<vi>)
      n176 = control-ref of="Target.X::10"() -> (w121:refnum<vi>)
      n177 = control-ref of="Target.Y::10"() -> (w120:refnum<vi>)
      n178 = control-ref of="Target.X::11"() -> (w119:refnum<vi>)
      n179 = control-ref of="Target.Y::11"() -> (w118:refnum<vi>)
      n180 = control-ref of="Target.X::12"() -> (w117:refnum<vi>)
      n181 = control-ref of="Target.Y::12"() -> (w116:refnum<vi>)
      n182 = call "IMAQ Create"("Image Name"="GUIdevice 8", "Image Type"=w106) -> ("New Image"=→"image::8":T9)  [unwired: 3 in, 1 out]
      n183 = call "IMAQ Create"("Image Name"="GUIdevice 9", "Image Type"=w106) -> ("New Image"=→"image::9":T9)  [unwired: 3 in, 1 out]
      n184 = call "IMAQ Create"("Image Name"="GUIdevice 10", "Image Type"=w106) -> ("New Image"=→"image::10":T9)  [unwired: 3 in, 1 out]
      n185 = call "IMAQ Create"("Image Name"="GUIdevice 6", "Image Type"=w106) -> ("New Image"=→"image::6":T9)  [unwired: 3 in, 1 out]
      n186 = call "IMAQ Create"("Image Name"="GUIdevice 7", "Image Type"=w106) -> ("New Image"=→"image::7":T9)  [unwired: 3 in, 1 out]
      n187 = call "IMAQ Create"("Image Name"="GUIdevice 11", "Image Type"=w106) -> ("New Image"=→"image::11":T9)  [unwired: 3 in, 1 out]
      n188 = call "IMAQ Create"("Image Name"="GUIdevice 12", "Image Type"=w106) -> ("New Image"=→"image::12":T9)  [unwired: 3 in, 1 out]
      n189 = call "IMAQ Create"("Image Name"="GUIdevice 2") -> ("New Image"=→"image::2":T9)  [unwired: 4 in, 1 out]
      n190 = call "IMAQ Create"("Image Name"="GUIdevice 4", "Image Type"=w106) -> ("New Image"=→"image::4":T9)  [unwired: 3 in, 1 out]
      n191 = call "IMAQ Create"("Image Name"="GUIdevice 1", "Image Type"=w106) -> ("New Image"=→"image::1":T9)  [unwired: 3 in, 1 out]
      n192 = call "IMAQ Create"("Image Name"="GUIdevice 3", "Image Type"=w106) -> ("New Image"=→"image::3":T9)  [unwired: 3 in, 1 out]
      n193 = call "IMAQ Create"("Image Name"="GUIdevice 5", "Image Type"=w106) -> ("New Image"=→"image::5":T9)  [unwired: 3 in, 1 out]
      n194 = Build Array("GUIdevice 1", "GUIdevice 2", "GUIdevice 3", "GUIdevice 4", "GUIdevice 5", "GUIdevice 6", "GUIdevice 7", "GUIdevice 8", "GUIdevice 9", "GUIdevice 10", "GUIdevice 11", "GUIdevice 12") -> (w135:string[])
      "CCDs" <- w135
      n195 = property on="image::8" class="ImageControl"("Caption.Text"="GUIdevice 8") -> ()  [unwired: 2 in, 2 out]
      n196 = property on="image::10" class="ImageControl"("Caption.Text"="GUIdevice 10") -> ()  [unwired: 2 in, 2 out]
      n197 = property on="image::9" class="ImageControl"("Caption.Text"="GUIdevice 9") -> ()  [unwired: 2 in, 2 out]
      n198 = property on="image::1" class="ImageControl"("Caption.Text"="GUIdevice 1") -> ()  [unwired: 2 in, 2 out]
      n199 = property on="image::2" class="ImageControl"("Caption.Text"="GUIdevice 2") -> ()  [unwired: 2 in, 2 out]
      n200 = property on="image::3" class="ImageControl"("Caption.Text"="GUIdevice 3") -> ()  [unwired: 2 in, 2 out]
      n201 = property on="image::4" class="ImageControl"("Caption.Text"="GUIdevice 4") -> ()  [unwired: 2 in, 2 out]
      n202 = property on="image::5" class="ImageControl"("Caption.Text"="GUIdevice 5") -> ()  [unwired: 2 in, 2 out]
      n203 = property on="image::6" class="ImageControl"("Caption.Text"="GUIdevice 6") -> ()  [unwired: 2 in, 2 out]
      n204 = property on="image::7" class="ImageControl"("Caption.Text"="GUIdevice 7") -> ()  [unwired: 2 in, 2 out]
      n205 = property on="image::11" class="ImageControl"("Caption.Text"="GUIdevice 11") -> ()  [unwired: 2 in, 2 out]
      n206 = property on="image::12" class="ImageControl"("Caption.Text"="GUIdevice 12") -> ()  [unwired: 2 in, 2 out]
      n207 = Array To Cluster(array=w135) -> (cluster=→"Cameras":T22)
      n208 = Bundle("Target.X::1"=w161, "Target.Y::1"=w160) -> (w145:T23)  [unwired: 1 in]
      n209 = Bundle("Target.X::2"=w159, "Target.Y::2"=w158) -> (w144:T24)  [unwired: 1 in]
      n210 = Bundle("Target.X::3"=w157, "Target.Y::3"=w156) -> (w143:T25)  [unwired: 1 in]
      n211 = Bundle("Target.X::4"=w155, "Target.Y::4"=w154) -> (w136:T26)  [unwired: 1 in]
      n212 = Bundle("Target.X::5"=w153, "Target.Y::5"=w152) -> (w142:T27)  [unwired: 1 in]
      n213 = Bundle("Target.X::6"=w151, "Target.Y::6"=w150) -> (w141:T28)  [unwired: 1 in]
      n214 = Bundle("Target.X::7"=w149, "Target.Y::7"=w148) -> (w140:T29)  [unwired: 1 in]
      n215 = Bundle("Target.X::8"=w147, "Target.Y::8"=w146) -> (w139:T30)  [unwired: 1 in]
      n216 = Bundle("Target.X::12"=w117, "Target.Y::12"=w116) -> (w112:T31)  [unwired: 1 in]
      n217 = Bundle("Target.X::9"=w123, "Target.Y::9"=w122) -> (w115:T32)  [unwired: 1 in]
      n218 = Bundle("Target.X::10"=w121, "Target.Y::10"=w120) -> (w114:T33)  [unwired: 1 in]
      n219 = Bundle("Target.X::11"=w119, "Target.Y::11"=w118) -> (w113:T34)  [unwired: 1 in]
      n220 = property on="CCDs" class="Ring (strict)"("Strings []"=w135) -> ()  [unwired: 2 in, 2 out]
      n221 = Build Array(w145, w144, w143, w136, w142, w141, w140, w139, w115, w114, w113, w112) -> (w138:T35)
      n222 = Tick Count (ms)() -> (millisecond timer value=→"millisecond timer value":u32)
      n223 = property on="Feedback Global" class="Bool (strict)"("Value"=FALSE ("Feedback Global")) -> ()  [unwired: 2 in, 2 out]
      n224 = Get Date/Time In Seconds() -> (seconds since 1Jan1904=w125:timestamp)
      n225 = Format Date/Time String(time format string (%c)="%Y%m%d%H%M", seconds (now)=w125) -> (date/time string=w124:string)  [unwired: 1 in]
      n226 = Concatenate Strings(w124, "Beampointing_Pico.tdms" ("string")) -> (w128:string)
      n227 = String To Path(string=w128) -> (path=w127:path)
      n228 = Build Path(base path=w34, name or relative path=w127) -> (appended path=w130:path)
      n229 = call <vilib>:"Add State(s) to Queue__jki_lib_state_machine.vi"("State(s) in (\"\")"="Macro: Initialize") -> ("States Out"=w236:string)  [unwired: 14 in]
      n230 = call "supergui create stop queue.vi"() -> ("STOP Queue out"=w32:refnum<queue>)  [unwired: 11 in]
      n231 = Create User Event(user event datatype=T15 {"EventEnum"=enum."new data", "Device name"="Device name"} ("New Event")) -> (user event=w244:refnum<user-event>, error out=w246:errorcluster)  [unwired: 1 in]
      "tcp data event" <- w244
      n232 = while "JKI - String-Based Queued State Machine (Basic) v1.0" {
        shift-right: [w270] -> w134
        shift-left: _ -> [w258]
        shift-right: [w273] -> w162
        shift-left: _ -> [w269]
        shift-right: [w272] -> _
        shift-left: w236 -> [w274]
        tunnel: w138 -> [w267]
        tunnel: w135 -> [w265]
        tunnel: [w265] -> w163
        tunnel: w138 -> [w266]
        tunnel: w130 -> [w256]
        tunnel: w34 -> [w255]
        tunnel: T14 {"Draw"=TRUE, "Target"={"x"=25.0, "y"=25.0}, "Size"={"x"=25.0, "y"=25.0}, "Angle"=0.0, "Color"=8322834, "Thickness"=1, "CrosshairLabel"="xhair"} ("Crosshair") -> [w254]
        stop <- w271 stop-if-true
        n233 = Unbundle By Name(w258) -> ("active cams"=w257:string[])
        n234 = call <vilib>:"Parse State Queue__jki_lib_state_machine.vi"("State Queue"=w274, "Error In (no error)"=w269) -> ("Remaining States"=w276:string, "Current State"=w277:string, "Arguments"=w275:string)  [unwired: 11 in]
        "Current State" <- w277
        n235 = case shown="\"Center\"" w277 {
          selector: w277 -> [_ _ w564 _ _ _ _ _ _ _ _ _ _ _ _ _ _ _ _ _ _ _ _ _ _ _ _ _ _ _ _ _ _ _ _ _ _ _ _ _]
          tunnel: w276 -> [w306 w563 w568 w586 w593 w598 w602 w639 w657 w661 w665 w671 w682 w706 w716 w726 w730 w752 w854 w907 w920 w929 w956 w977 w981 w1000 w1139 w1293 w1384 w1450 w1488 w1508 w1523 w1612 w1664 w1674 w1681 w1714 w1740 w1767]
          tunnel: w275 -> [_ _ _ _ _ _ _ _ _ _ _ w666 w677 _ _ _ _ w747 w805 _ w917 _ _ _ _ w1002 _ w1271 w1361 _ _ _ _ _ _ _ w1678 _ _ _]
          tunnel: w258 -> [w304 w560 w566 w576 w590 w596 w599 _ w653 w658 w663 w669 w676 w703 w714 w718 w727 w744 w806 w905 w912 w925 w948 w970 w978 w984 w1133 w1286 w1377 w1447 w1459 w1505 w1520 w1586 w1661 w1671 w1677 w1702 w1737 w1758]
          tunnel: [w303 w561 w570 w584 errorcluster {"status"=FALSE, "code"=0, "source"=""} ("error out") w595 w600 w611 w650 w659 w662 w667 w679 w704 w715 w724 w728 w748 w810 w897 w918 w927 w954 w975 w979 w1004 w1163 w1291 w1382 w1448 w1486 w1506 w1521 w1571 w1662 w1672 w1679 w1684 w1738 w1765] -> w273
          tunnel: w269 -> [w302 w561 w569 w584 w589 w595 w600 w617 w655 w659 w662 w668 w680 w704 w715 w724 w728 w748 w808 w888 w918 w927 w954 w975 w979 w1004 w1163 w1291 w1382 w1448 w1486 w1506 w1521 w1607 w1662 w1672 w1679 w1700 w1738 w1765]
          tunnel: [w305 w562 w567 w585 w592 w597 w601 w638 w656 w660 w664 w670 w681 w705 w707 w725 w729 w738 w853 w906 w919 w928 w955 w976 w980 w1007 w1164 w1292 w1383 w1449 w1487 w1507 w1522 w1574 w1663 w1673 w1680 w1713 w1739 w1766] -> w272
          tunnel: [_ _ _ _ _ TRUE _ _ _ _ _ _ _ _ _ _ _ _ _ _ _ _ _ _ _ _ _ _ _ _ _ _ _ _ _ _ _ _ _ _] -> w271
          tunnel: [w299 w560 w566 w575 w590 w596 w599 w605 w653 w658 w663 w669 w676 w703 w714 w718 w727 w749 w843 w905 w911 w924 w947 w969 w978 w1029 w1132 w1286 w1377 w1446 w1459 w1505 w1520 w1586 w1660 w1671 w1676 w1703 w1737 w1757] -> w270
          tunnel: "update speed [ms]" -> [w301 _ _ _ _ _ _ _ _ _ _ _ _ _ _ _ _ _ _ _ _ _ _ _ _ _ _ _ _ _ _ _ _ _ _ _ _ _ _ _]
          tunnel: w267 -> [w298 _ _ _ _ _ _ _ _ _ _ _ _ _ _ _ _ _ _ _ _ _ _ _ _ w1027 _ _ _ _ _ _ _ _ _ _ _ _ w1721 _]
          tunnel: w265 -> [w300 _ _ _ _ _ _ w610 _ _ _ _ _ _ _ _ _ w751 w807 _ w913 _ _ _ _ w992 w1129 w1290 w1381 _ w1460 _ w1509 w1610 _ _ _ _ _ _]
          tunnel: w256 -> [_ _ _ _ _ _ _ w615 _ _ _ _ _ _ _ _ _ _ _ _ _ _ _ _ _ _ _ _ _ _ _ _ _ _ _ _ _ _ _ _]
          tunnel: w255 -> [_ _ _ _ _ _ _ _ _ _ _ _ _ _ _ _ _ _ _ _ _ _ _ _ _ _ _ _ _ _ _ _ _ _ _ _ _ w1693 _ _]
          frame "", "Idle" {
            # "executes when the state queue is empty"
            n236 = event shown="[0] Timeout" {
              selector: _ -> [_ _ _ _ _ _ _ _ _ _ _ _ _ _ _ _ _ _]
              dyn-events: _ -> [_ _ _ _ _ _ _ _ _ _ _ _ _ _ _ _ _ _]
              timeout: w301 -> [_ _ _ _ _ _ _ _ _ _ _ _ _ _ _ _ _ _]
              tunnel: w306 -> [w309 w436 w451 w470 w475 w480 w485 w491 w498 w503 w514 w519 w528 w533 w539 w545 w553 w559]
              tunnel: [w324 w435 w450 w469 w474 w479 w484 w490 w497 w502 w513 w518 w527 w532 w538 w544 w552 w558] -> w305
              tunnel: w304 -> [w314 w433 w447 w466 w472 w477 w482 w488 w495 w500 w512 w516 w521 w530 w536 w542 w550 w556]
              tunnel: [w318 w434 w449 w468 w473 w478 w483 w489 w496 w501 w504 w517 w526 w531 w537 w543 w551 w557] -> w303
              tunnel: w302 -> [w321 w434 w449 w468 w473 w478 w483 w489 w496 w501 w505 w517 w526 w531 w537 w543 w551 w557]
              tunnel: [w323 w433 w447 w465 w472 w477 w482 w488 w495 w500 w512 w516 w521 w530 w536 w542 w550 w556] -> w299
              tunnel: w300 -> [w341 _ w443 _ _ _ _ _ _ _ _ _ _ _ _ _ _ _]
              tunnel: w298 -> [_ _ w445 _ _ _ _ _ _ _ _ _ _ _ _ _ _ _]
              event Timeout {
                n237 = event-data() -> ()  [unwired: 1 in, 1 out]
                n238 = Unbundle By Name(w314) -> ("Centroid X"=w311:dbl[][], "Centroid Y"=w351:dbl[][], "Size"=w344:dbl[][], "detection para"=w340:T3[], "active cams"=w335:string[], "thresholds"=w332:cluster{"Lower value":sgl, "Upper value":sgl}[])
                n239 = Unbundle By Name(w314) -> ("active ccd"=w313:i32)
                n240 = call <userlib>:"Tick Count (ms)__ogtk.vi"("error in (no error)"=w321) -> ("error out"=w320:errorcluster, "millisecond timer value"=→"millisecond timer 2":u32)  [unwired: 9 in]
                n241 = for {
                  N: 12 ("Numeric 2") -> [_]
                  tunnel: w335 -> [w396] mode=indexing
                  tunnel: [w397] -> w349 mode=indexing
                  tunnel: w341 -> [w420]
                  tunnel: w340 -> [w418]
                  tunnel: [w416] -> w317 mode=indexing
                  tunnel: [w415] -> w315 mode=indexing
                  tunnel: [w413] -> w336 mode=indexing
                  tunnel: "autodetect" -> [w407]
                  tunnel: w320 -> [w421]
                  tunnel: [w422] -> w342
                  shift-right: [w404] -> w312
                  shift-left: w332 -> [w406]
                  shift-right: [w391] -> w350
                  shift-left: w311 -> [w393]
                  shift-right: [w387] -> w352
                  shift-left: w351 -> [w389]
                  shift-right: [w381] -> w343
                  shift-left: w344 -> [w383]
                  w385 = 0 ("index")
                  n242 = call-poly <userlib>:"Filter 1D Array__ogtk.vi"("items to filter"=w396, "array"=w420) -> ("filtered item indices"=w419:i32[])  [unwired: 4 in, 1 out]
                  n243 = Index Array(array=w419) -> (element=w382:i32)  [unwired: 1 in]
                  n244 = Index Array(array=w383, index (row)=w382) -> (element=w411:dbl[])  [unwired: 1 in]
                  n245 = Index Array(array=w389, index (row)=w382) -> (element=w412:dbl[])  [unwired: 1 in]
                  n246 = Index Array(array=w406, index=w382) -> (element=w410:cluster{"Lower value":sgl, "Upper value":sgl})
                  n247 = Index Array(array=w393, index (row)=w382) -> (element=w395:dbl[])  [unwired: 1 in]
                  n248 = Index Array(array=w418, index=w382) -> (element=w414:T3)
                  n249 = call "CENTRIOD DETECTION.vi"("Refnum in"=w396, "auto threshold"=w407, "Threshold Range In"=w410, "beam detection para"=w414, "error in (no error)"=w421) -> ("Bounding Rect"=w413:T36, "Particle Reports (Pixels)"=w415:T1, "Threshold Range Out"=w405:cluster{"Lower value":sgl, "Upper value":sgl}, "Centriod"=w423:cluster{"X":dbl, "Y":dbl}, "error out"=w422:errorcluster)  [unwired: 7 in, 3 out]
                  n250 = Unbundle By Name(w423) -> ("X"=w394:dbl, "Y"=w390:dbl)
                  n251 = Empty Array?(array=w415) -> (empty?=w417:bool)
                  n252 = Not(x=w417) -> (.not. x?=w416:bool)
                  n253 = Replace Array Subset(array=w406, new element=w405, index=w382) -> (w404:cluster{"Lower value":sgl, "Upper value":sgl}[])
                  n254 = Unbundle By Name(w413) -> ("Right"=w403:dbl, "Left"=w402:dbl, "Bottom"=w401:dbl, "Top"=w400:dbl)
                  n255 = Subtract(x=w403, y=w402) -> (x-y=w398:dbl)
                  n256 = Subtract(x=w401, y=w400) -> (x-y=w399:dbl)
                  n257 = Multiply(x=w398, y=w399) -> (x*y=w386:dbl)
                  n258 = Insert Into Array(array=w412, index=w385, new element=w390) -> (w388:dbl[])
                  n259 = Insert Into Array(array=w411, index=w385, new element=w386) -> (w384:dbl[])
                  n260 = Insert Into Array(array=w395, index=w385, new element=w394) -> (w392:dbl[])
                  n261 = for {
                    shift-right: [w424] -> w408
                    shift-left: dbl[] [] ("Array 4") -> [w427]
                    tunnel: w388 -> [w425] mode=indexing
                    n262 = Equal To 0?(x=w425) -> (x = 0?=w426:bool)
                    n263 = case shown="False" w426 {
                      tunnel: w427 -> [w430 w431]
                      tunnel: w425 -> [w429 _]
                      tunnel: [w428 w431] -> w424
                      frame False {
                        n264 = Build Array (concatenate)(w430, w429) -> (w428:dbl[])
                      }
                      frame True {
                      }
                    }
                  }
                  n265 = Replace Array Subset(array=w393, new element=w392, index (row)=w382) -> (w391:dbl[][])  [unwired: 1 in]
                  n266 = Replace Array Subset(array=w389, new element=w388, index (row)=w382) -> (w387:dbl[][])  [unwired: 1 in]
                  n267 = Replace Array Subset(array=w383, new element=w384, index (row)=w382) -> (w381:dbl[][])  [unwired: 1 in]
                  n268 = Array Size(array=w408) -> (size(s)=w397:i32)
                }
                "detected" <- w317
                "Particle Reports (Pixels)" <- w315
                "Box" <- w336
                n269 = Bundle(0, 1, "Centroid X"=w311) -> (→"Status":cluster{i32, i32, "Centroid X":dbl[][]})  [unwired: 1 in]
                n270 = Index Array(array=w315, index (row)=w313) -> (element=→"particles":T1)  [unwired: 1 in]
                n271 = call <vilib>:"Clear Errors.vi"("error in (no error)"=w342) -> ("error out"=w318:errorcluster)  [unwired: 5 in, 1 out]
                n272 = local read "Img to avg"() -> (w326:i32)
                n273 = local read "Numeric"() -> (w329:dbl)
                n274 = Increment(x=w326) -> (x+1=w325:i32)
                n275 = Greater Or Equal?(x=w329, y=w325) -> (x >= y?=w322:bool)
                n276 = Increment(x=w329) -> (x+1=w328:dbl)
                n277 = Select(t=0.0, s=w322, f=w328) -> (s? t:f=w327:dbl)
                n278 = local write "Numeric"(w327) -> ()
                n279 = for {
                  tunnel: w349 -> [w373] mode=indexing
                  tunnel: w335 -> [w380] mode=indexing
                  shift-right: [w375] -> w345
                  shift-left: "" ("GUIdevice 7") -> [w378]
                  tunnel: [w368] -> w347 mode=indexing
                  tunnel: "Detection Rate" -> [w372]
                  tunnel: w327 -> [w370]
                  n280 = local read "Img to avg"() -> (w374:i32)
                  n281 = Greater Or Equal?(x=w373, y=w374) -> (x >= y?=w369:bool)
                  n282 = Multiply(x=w372, y=w370) -> (x*y=w371:dbl)
                  n283 = Greater Or Equal?(x=w373, y=w371) -> (x >= y?=w367:bool)
                  n284 = And(x=w369, y=w367) -> (x .and. y?=w368:bool)
                  n285 = Select(t=w380, s=w368, f="") -> (s? t:f=w376:string)
                  n286 = Concatenate Strings(w378, "\t", w376) -> (w375:string)
                }
                n287 = Bundle By Name(cluster=w314, "thresholds"=w312, "detected"=w317) -> (w333:T37)
                n288 = Bundle By Name(cluster=w333, "Centroid X"=w350, "Centroid Y"=w352, "Size"=w343) -> (w308:T37)
                n289 = Unbundle By Name(w308) -> ("img to avg"=w307:i32)
                n290 = Or Array Elements(Boolean array=w347) -> (logical OR=w346:bool)
                n291 = case shown="True" w322 {
                  tunnel: w308 -> [w353 w360]
                  tunnel: [w353 w359] -> w323
                  tunnel: w307 -> [_ w355]
                  frame False {
                  }
                  frame True {
                    n292 = Decrement(x=w355) -> (x-1=w354:i32)
                    n293 = Initialize Array(0.0 ("element"), 12 ("dimension size"), w354) -> (w356:dbl[][])
                    n294 = Bundle By Name(cluster=w360, "Centroid X"=w356, "Centroid Y"=w356, "Size"=w356) -> (w359:T37)
                  }
                }
                n295 = case shown="True" w346 {
                  tunnel: w345 -> [_ w365]
                  tunnel: w309 -> [w361 w363]
                  tunnel: [w361 w362] -> w324
                  frame False {
                  }
                  frame True {
                    n296 = call <vilib>:"Build State String with Arguments__jki_lib_state_machine.vi"("Arguments (\"\")"=w365, "State"="detected") -> ("State with Arguments"=w364:string)  [unwired: 4 in]
                    n297 = call <vilib>:"Add State(s) to Queue__jki_lib_state_machine.vi"("State(s) in (\"\")"=w363, "State(s) at Back (\"\")"=w364) -> ("States Out"=w362:string)  [unwired: 13 in]
                  }
                }
              }
              event "stop": Value Change {
                # "Exit Button Value Change (pressed) Event\n(this executes Macro: Exit to terminate the VI)"
                n298 = event-data() -> ()  [unwired: 1 in, 6 out]
                n299 = call <vilib>:"Add State(s) to Queue__jki_lib_state_machine.vi"("State(s) in Front (\"\")"="Macro: Exit", "State(s) in (\"\")"=w436) -> ("States Out"=w435:string)  [unwired: 13 in]
              }
              event Value Change {
                n300 = event-data() -> ()  [unwired: 1 in, 6 out]
                n301 = property on="Set Centriod Target" class="Bool (strict)"("Value"=FALSE) -> ()  [unwired: 2 in, 2 out]
                n302 = Unbundle By Name(w447) -> ("active ccd"=w439:i32, "Centroid X"=w438:dbl[][], "Centroid Y"=w437:dbl[][])
                n303 = Index Array(array=w443, index=w439) -> (element=w442:string)
                n304 = Concatenate Strings("Do want to update the target of " ("message"), w442, "?" ("string")) -> (w440:string)
                n305 = Two Button Dialog(message=w440) -> (T button?=w446:bool)  [unwired: 2 in]
                n306 = case shown="True" w446 {
                  tunnel: w445 -> [_ w458]
                  tunnel: w439 -> [_ w457]
                  tunnel: w438 -> [_ w464]
                  tunnel: w437 -> [_ w459]
                  frame False {
                  }
                  frame True {
                    n307 = Index Array(array=w464, index (row)=w457) -> (element=w463:dbl[])  [unwired: 1 in]
                    n308 = Index Array(array=w459, index (row)=w457) -> (element=w460:dbl[])  [unwired: 1 in]
                    n309 = Index Array(array=w458, index=w457) -> (element=w456:T31)
                    n310 = Unbundle By Name(w456) -> ("Target.X::12"=w455:refnum<vi>, "Target.Y::12"=w453:refnum<vi>)
                    n311 = Reverse 1D Array(array=w463) -> (reversed array=w462:dbl[])
                    n312 = Reverse 1D Array(array=w460) -> (reversed array=w461:dbl[])
                    n313 = Index Array(array=w462) -> (element=w454:dbl)  [unwired: 1 in]
                    n314 = Index Array(array=w461) -> (element=w452:dbl)  [unwired: 1 in]
                    n315 = property class="DigNum (strict)"(reference=w455, "Val(Sgnl)"=w454) -> ()  [unwired: 1 in, 2 out]
                    n316 = property class="DigNum (strict)"(reference=w453, "Val(Sgnl)"=w452) -> ()  [unwired: 1 in, 2 out]
                  }
                }
                n317 = call <vilib>:"Add State(s) to Queue__jki_lib_state_machine.vi"("State(s) in (\"\")"=w451) -> ("States Out"=w450:string)  [unwired: 14 in]
              }
              event "Feedback Global": Value Change {
                # "Exit Button Value Change (pressed) Event\n(this executes Macro: Exit to terminate the VI)"
                n318 = event-data() -> ("NewVal"=w467:bool)  [unwired: 1 in, 5 out]
                n319 = call <vilib>:"Add State(s) to Queue__jki_lib_state_machine.vi"("State(s) in (\"\")"=w470) -> ("States Out"=w469:string)  [unwired: 14 in]
                n320 = Bundle By Name(cluster=w466, "Feedback global"=w467) -> (w465:T37)
              }
              event Value Change {
                n321 = event-data() -> ()  [unwired: 1 in, 6 out]
                n322 = call <vilib>:"Add State(s) to Queue__jki_lib_state_machine.vi"("State(s) in Front (\"\")"="Move Config", "State(s) in (\"\")"=w475) -> ("States Out"=w474:string)  [unwired: 13 in]
              }
              event Value Change {
                n323 = event-data() -> ()  [unwired: 1 in, 6 out]
                n324 = call <vilib>:"Add State(s) to Queue__jki_lib_state_machine.vi"("State(s) in Front (\"\")"="Detection Config", "State(s) in (\"\")"=w480) -> ("States Out"=w479:string)  [unwired: 13 in]
              }
              event "associated motors": Value Change {
                n325 = event-data() -> ()  [unwired: 1 in, 6 out]
                n326 = call <vilib>:"Add State(s) to Queue__jki_lib_state_machine.vi"("State(s) in (\"\")"=w485, "State(s) at Back (\"\")"="Motor Config" ("State(s) at Back (\"\")")) -> ("States Out"=w484:string)  [unwired: 13 in]
              }
              event "Reset History": Value Change {
                n327 = event-data() -> ()  [unwired: 1 in, 6 out]
                n328 = call <vilib>:"Add State(s) to Queue__jki_lib_state_machine.vi"("State(s) in (\"\")"=w491, "State(s) at Back (\"\")"="Reset History" ("State(s) at Back (\"\")")) -> ("States Out"=w490:string)  [unwired: 13 in]
                n329 = property on="Reset History" class="Bool (strict)"("Value"=FALSE ("Reset History")) -> ()  [unwired: 2 in, 2 out]
              }
              event "ActiveMotor": Value Change {
                n330 = event-data() -> ("NewVal"=w493:u16)  [unwired: 1 in, 5 out]
                n331 = property on="ActiveMotor" class="Ring (strict)"() -> ("Strings []"=w494:string[])  [unwired: 2 in, 2 out]
                n332 = Index Array(array=w494, index=w493) -> (element=w492:string)
                n333 = property on="ActiveMotorName::99" class="Str"("Val(Sgnl)"=w492) -> ()  [unwired: 2 in, 2 out]
                n334 = call <vilib>:"Add State(s) to Queue__jki_lib_state_machine.vi"("State(s) in (\"\")"=w498) -> ("States Out"=w497:string)  [unwired: 14 in]
              }
              event "Save Config": Value Change {
                n335 = event-data() -> ()  [unwired: 1 in, 6 out]
                n336 = call <vilib>:"Add State(s) to Queue__jki_lib_state_machine.vi"("State(s) in (\"\")"=w503, "State(s) at Back (\"\")"="Save Config" ("State(s) at Back (\"\")")) -> ("States Out"=w502:string)  [unwired: 13 in]
              }
              event "Load Config": Value Change {
                n337 = event-data() -> ()  [unwired: 1 in, 6 out]
                n338 = call "File Dialog2"("error in"=w505, "pattern (all files)"="*.cfg", "pattern label"="config") -> ("selected path"=w509:path, "error out"=w504:errorcluster)  [unwired: 9 in, 2 out]
                n339 = Path To String(path=w509) -> (string=w507:string)
                "config path" <- w507
                n340 = call <vilib>:"Build State String with Arguments__jki_lib_state_machine.vi"("Arguments (\"\")"=w507, "State"="Load Config" ("State(s) at Back (\"\")")) -> ("State with Arguments"=w506:string)  [unwired: 4 in]
                n341 = call <vilib>:"Add State(s) to Queue__jki_lib_state_machine.vi"("State(s) in (\"\")"=w514, "State(s) at Back (\"\")"=w506) -> ("States Out"=w513:string)  [unwired: 13 in]
              }
              event "Save Stats": Value Change {
                n342 = event-data() -> ()  [unwired: 1 in, 6 out]
                n343 = call <vilib>:"Add State(s) to Queue__jki_lib_state_machine.vi"("State(s) in (\"\")"=w519, "State(s) at Back (\"\")"="Save Stats" ("State(s) at Back (\"\")")) -> ("States Out"=w518:string)  [unwired: 13 in]
              }
              event "active CCDs": Value Change {
                n344 = event-data() -> ("NewVal"=w525:i32)  [unwired: 1 in, 5 out]
                n345 = Unbundle By Name(w521) -> ("active cams"=w520:string[])
                n346 = Index Array(array=w520, index=w525) -> (element=w523:string)
                n347 = call <vilib>:"Build State String with Arguments__jki_lib_state_machine.vi"("Arguments (\"\")"=w523, "State"="active" ("State(s) at Back (\"\")")) -> ("State with Arguments"=w522:string)  [unwired: 4 in]
                n348 = call <vilib>:"Add State(s) to Queue__jki_lib_state_machine.vi"("State(s) in (\"\")"=w528, "State(s) at Back (\"\")"=w522) -> ("States Out"=w527:string)  [unwired: 13 in]
              }
              event "Center": Value Change {
                n349 = event-data() -> ()  [unwired: 1 in, 6 out]
                n350 = call <vilib>:"Add State(s) to Queue__jki_lib_state_machine.vi"("State(s) in (\"\")"=w533, "State(s) at Back (\"\")"="Center" ("State(s) at Back (\"\")")) -> ("States Out"=w532:string)  [unwired: 13 in]
              }
              event "new tdms": Value Change {
                n351 = event-data() -> ()  [unwired: 1 in, 6 out]
                n352 = property on="new tdms" class="Bool (strict)"("Value"=FALSE ("new tdms")) -> ()  [unwired: 2 in, 2 out]
                n353 = call <vilib>:"Add State(s) to Queue__jki_lib_state_machine.vi"("State(s) in (\"\")"=w539, "State(s) at Back (\"\")"="newtdms" ("State(s) at Back (\"\")")) -> ("States Out"=w538:string)  [unwired: 13 in]
              }
              event "deivice ini": Value Change {
                n354 = event-data() -> ()  [unwired: 1 in, 6 out]
                n355 = property on="deivice ini" class="Bool (strict)"("Value"=FALSE ("new tdms")) -> ()  [unwired: 2 in, 2 out]
                n356 = call <vilib>:"Add State(s) to Queue__jki_lib_state_machine.vi"("State(s) in (\"\")"=w545, "State(s) at Back (\"\")"="Device Ini" ("State(s) at Back (\"\")")) -> ("States Out"=w544:string)  [unwired: 13 in]
              }
              event "Img to avg": Value Change {
                n357 = event-data() -> ()  [unwired: 1 in, 6 out]
                n358 = property on="Img to avg" class="DigNum (strict)"() -> ("Value"=w548:i32)  [unwired: 2 in, 2 out]
                n359 = Number To Decimal String(number=w548) -> (decimal integer string=w547:string)  [unwired: 1 in]
                n360 = call <vilib>:"Build State String with Arguments__jki_lib_state_machine.vi"("Arguments (\"\")"=w547, "State"="ImgToAvg" ("State(s) at Back (\"\")")) -> ("State with Arguments"=w546:string)  [unwired: 4 in]
                n361 = call <vilib>:"Add State(s) to Queue__jki_lib_state_machine.vi"("State(s) in (\"\")"=w553, "State(s) at Back (\"\")"=w546) -> ("States Out"=w552:string)  [unwired: 13 in]
              }
              event Panel Close? {
                # "Discard the event because we'll close the front panel ourselves in Macro: Exit"
                # "Close Panel button (pressed) Event\n(this executes Macro: Exit to terminate the VI)"
                n362 = event-data() -> ()  [unwired: 1 in, 1 out]
                n363 = call <vilib>:"Add State(s) to Queue__jki_lib_state_machine.vi"("State(s) in Front (\"\")"="Macro: Exit", "State(s) in (\"\")"=w559) -> ("States Out"=w558:string)  [unwired: 13 in]
                n364 = event-data("Discard?"=TRUE) -> ()  [unwired: 1 in, 1 out]
              }
            }
          }
          frame "---------- Core ----------" {
            # "Do not put any code in this frame.\n(it is a separator no-op)"
            n365 = call <vilib>:"Add State(s) to Queue__jki_lib_state_machine.vi"("State(s) in (\"\")"=w563) -> ("States Out"=w562:string)  [unwired: 14 in]
          }
          frame Default {
            w573 = 42 items=["No error", "Argument error", "Memory is full", "Out of zone", "End of file", "File already open", "Generic file I/O error", "File not found", "File permission error", "Disk is full", "Duplicate path", "Too many files open", "System feature not enabled", "Resource file not found", "Cannot add resource", "Resource not found", "Image not found", "Image memory error", "Pen does not exist", "Config type invalid", "Config token not found", "Config parse error", "Config memory error", "Bad external code format", "Bad external code offset", "External code not present", "Null window", "Destroy window error", "Null menu", "Print aborted", "Bad print record", "Print driver error", "Windows error during printing", "Memory error during printing", "Print dialog error", "Generic print error", "Invalid device refnum", "Device not found", "Device parameter error", "Device unit error", "Cannot open device", "Device call aborted", "Generic error", "Cancelled by user", "Object ID too low", "Object ID too high", "Object not in heap", "Unknown heap", "Unknown object (invalid DefProc)", "Unknown object (DefProc not in table)", "Message out of range", "Invalid (null) method", "Unknown message", "Manager call not supported", "Bad address", "Network operation in progress", "Network operation timed out", "Connection is busy", "Network attribute not supported", "Network error", "Address in use", "System out of memory", "Connection aborted", "Connection refused", "Not connected", "Already connected", "Connection closed", "Initialization error (interapplication manager)", "Bad occurrence", "Wait on unbound occurrence handler", "Occurrence queue overflow", "Datalog type conflict", "Unused", "Unrecognized type (interapplication manager)", "Memory corrupt", "Failed to make temporary DLL", "Old CIN version", "Drag socket not found", "Failed to load drop-object", "Failed to register OLE object", "Failed to release OLE object", "Format specifier type mismatch", "Unknown format specifier", "Too few format specifiers", "Too many format specifiers", "Scan failed", "Newer CIN version", "Error converting to variant", "Runtime menu error", "Password tampered", "Variant attribute not found", "Incompatible variant data type", "Event data is not available", "Event Store is not present", "Occurrence is not found", "Event Queue is not created", "Event info is not available", "Refnum passed is NULL", "Error retrieving Class GUID", "Error retrieving CoClass GUID", "Error retrieving TypeLib GUID.", "Bad built application magic bytes.", "Specific driver is different from the specific driver associated with the Logical Name.", "There is no session opened to the class driver.", "Max Error", "MAX - Error with config objects", "MAX - Error loading configuration", "MAX - Group not supported"]
            # "Current State"
            # "Do not delete, rename, or modify this frame.\n(this is used to capture unhandled states and typos)"
            # "Handle mistyped state name (developer tool)"
            n366 = Format Into String(format string="Software Exception: Unhandled State \"%s\"." ("message"), error in=w569, w564) -> (resulting string=w572:string, error out=w571:errorcluster)  [unwired: 1 in]
            n367 = call <vilib>:"Error Cluster From Error Code.vi"("show call chain? (False)"=TRUE, "error in (no error)"=w571, "error message (\"\")"=w572, "error code (0)"=w573) -> ("error out"=w570:errorcluster)  [unwired: 5 in]
            n368 = call <vilib>:"Add State(s) to Queue__jki_lib_state_machine.vi"("State(s) in (\"\")"=w568) -> ("States Out"=w567:string)  [unwired: 14 in]
          }
          frame "Initialize Core Data" {
            # "Do not delete, rename, or modify this frame.\n(this is used to determine panel behavior on exit)"
            # "originally closed?"
            # "exe?"
            # "If panel starts closed or is an EXE, then close it when we exit"
            n369 = property class="VI"() -> ("Front Panel.Open"=w583:bool)  [unwired: 2 in, 2 out]
            n370 = property class="App"() -> ("App.Kind"=w582:T17)  [unwired: 2 in, 2 out]
            n371 = control-ref of="Current VI Reference"() -> (w577:refnum<vi>)
            n372 = Not(x=w583) -> (.not. x?=w580:bool)
            n373 = Equal?(x=w582, y=T17."Run Time System" ("Application:Kind")) -> (x = y?=w579:bool)
            n374 = Or(x=w580, y=w579) -> (x .or. y?=w578:bool)
            n375 = Bundle By Name(cluster=w576, "Core.Current VI Reference"=w577, "Core.Close Panel on Exit?"=w578) -> (w575:T37)
            n376 = call <vilib>:"Add State(s) to Queue__jki_lib_state_machine.vi"("State(s) in (\"\")"=w586) -> ("States Out"=w585:string)  [unwired: 14 in]
          }
          frame "Error Handler" {
            w587 = T38 0 items=["no dialog", "OK message", "continue or stop message", "OK message + warnings", "continue/stop + warnings"] ("type of dialog (OK msg:1)")
            # "Unhandled Error -- Display it"
            # "Handle any errors here.\nYou can also output any states to clean-up after errors occur"
            # "Clear error"
            n377 = call <vilib>:"General Error Handler.vi"("type of dialog (OK msg:1)"=w587, "error in (no error)"=w589) -> ()  [unwired: 9 in, 5 out]
            n378 = call <vilib>:"Add State(s) to Queue__jki_lib_state_machine.vi"("State(s) in Front (\"\")"="/* Post Error States", "State(s) in (\"\")"=w593) -> ("States Out"=w592:string)  [unwired: 13 in]
          }
          frame "Exit" {
            # "Do not put any code in this frame.\n(No errors that occur here will be handled.)"
            n379 = call <vilib>:"Add State(s) to Queue__jki_lib_state_machine.vi"("State(s) in (\"\")"=w598) -> ("States Out"=w597:string)  [unwired: 14 in]
          }
          frame "---------- Data ----------" {
            # "Do not put any code in this frame.\n(It is a separator no-op. You can make a copy of this frame to create a new Data frame)"
            n380 = call <vilib>:"Add State(s) to Queue__jki_lib_state_machine.vi"("State(s) in (\"\")"=w602) -> ("States Out"=w601:string)  [unwired: 14 in]
          }
          frame "Data: Initialize" {
            w612 = bool[] [FALSE, FALSE, FALSE, FALSE, FALSE, FALSE, FALSE, FALSE, FALSE, FALSE, FALSE, TRUE]  # speedmode Y
            w613 = bool[] [FALSE, FALSE, FALSE, FALSE, FALSE, FALSE, FALSE, FALSE, FALSE, FALSE, FALSE, TRUE]  # speedmode X
            w614 = bool[] [FALSE, FALSE, FALSE, FALSE, TRUE, TRUE, TRUE, FALSE, FALSE, FALSE, FALSE, FALSE]  # detected
            w616 = cluster{"Lower value":sgl, "Upper value":sgl}[] [{"Lower value"=93.0, "Upper value"=255.0}, {"Lower value"=105.0, "Upper value"=255.0}, {"Lower value"=0.0, "Upper value"=255.0}, {"Lower value"=127.0, "Upper value"=255.0}, {"Lower value"=0.0, "Upper value"=255.0}, {"Lower value"=0.0, "Upper value"=255.0}, {"Lower value"=0.0, "Upper value"=255.0}, {"Lower value"=0.0, "Upper value"=255.0}, {"Lower value"=0.0, "Upper value"=255.0}, {"Lower value"=0.0, "Upper value"=255.0}, {"Lower value"=0.0, "Upper value"=255.0}, {"Lower value"=0.0, "Upper value"=255.0}]  # thresholds
            w624 = FALSE  # Feedback global
            w626 = 0  # active ccd
            w604 = 2  # img to avg
            w637 = T39 {"Current VI Reference"=refnum, "Close Panel on Exit?"=FALSE}  # Core
            # "Initialize the shift-register data, here.\n(data names are defined by what you wire into the bundle function)"
            n381 = disable-structure shown="Disabled" {
              disable-tunnel: w617 -> [w645 w649]
              disable-tunnel: w615 -> [w644 _]
              disable-tunnel: [w642 w649] -> w611
              disable-tunnel: w610 -> [w640 _]
              frame Disabled {
                n382 = TDMS Open(6:FALSE ("disable buffering (T)"), 7:enum16{"1.0", "2.0"}."2.0" ("file format version (2.0)"), 8:w645, 10:T18."create or replace" ("operation"), 11:w644) -> (0:w643:errorcluster, 3:w641:refnum<k34>)  [unwired: 2 in]
                n383 = call "TDMSbuffersize.vi"("error in (no error)"=w643, "group names"=w640, "Data Value Reference in"=w641) -> ("error out"=w642:errorcluster)  [unwired: 7 in, 1 out]
              }
              frame Enabled {
              }
            }
            n384 = call <vilib>:"Add State(s) to Queue__jki_lib_state_machine.vi"("State(s) in (\"\")"=w639) -> ("States Out"=w638:string)  [unwired: 14 in]
            n385 = Bundle("Core"=w637, "detection para"="detection para", "thresholds"=w616, "Centroid X"="Centroid X", "Centroid Y"="Centroid Y", "img to avg"=w604, "Mean Centroid X"="Mean Centroid X", "Mean Centroid Y"="Mean Centroid Y", "Offset X"="Offset X", "Offset Y"="Offset Y", "Offset X stats"="Offset X stats", "Offset Y stats"="Offset Y stats", "Size"="Size", "Mean Size"="Mean Size", "Time"="Time", "move properties"="move properties", "active axis refs 2"="active axis refs 2", "active ccd"=w626, "Feedback global"=w624, "Motor X"="Motor X", "Motor Y"="Motor Y", "active cams"="active cams", "Data Value Reference out"=refnum<k34> refnum, "detected"=w614, "speedmode X"=w613, "speedmode Y"=w612) -> (w606:T37)  [unwired: 1 in]
            n386 = Initialize Array(0.0 ("element"), 12 ("dimension size"), w604) -> (w607:dbl[][])
            n387 = Bundle By Name(cluster=w606, "Centroid X"=w607, "Centroid Y"=w607, "Size"=w607) -> (w605:T37)
          }
          frame "Data: Cleanup" {
            # "Cleanup any data and references, here.\n(this is called automatically, by the Macro: Exit)"
            n388 = Unbundle By Name(w653) -> ("Core.Current VI Reference"=w654:refnum<vi>)
            n389 = Close Reference(reference=w654, error in (no error)=w655) -> (error out=w651:errorcluster)
            n390 = Unbundle By Name(w653) -> ("Data Value Reference out"=w652:refnum<k34>)
            n391 = TDMS Close(8:w651, 11:w652) -> (0:w650:errorcluster)  [unwired: 1 out]
            n392 = call <vilib>:"Add State(s) to Queue__jki_lib_state_machine.vi"("State(s) in (\"\")"=w657) -> ("States Out"=w656:string)  [unwired: 14 in]
          }
          frame "---------- UI ----------" {
            # "Do not put any code in this frame.\n(It is a separator no-op. You can make a copy of this frame to create a new UI frame)"
            n393 = call <vilib>:"Add State(s) to Queue__jki_lib_state_machine.vi"("State(s) in (\"\")"=w661) -> ("States Out"=w660:string)  [unwired: 14 in]
          }
          frame "UI: Initialize" {
            # "Initialize the User Interface, here.\n(this is called automatically, by the Macro: Init)"
            n394 = call <vilib>:"Add State(s) to Queue__jki_lib_state_machine.vi"("State(s) in (\"\")"=w665) -> ("States Out"=w664:string)  [unwired: 14 in]
          }
          frame "UI: Cursor Set" {
            # "Argument"
            # "Set and Unset Cursor Busy.\n(Usage: \"UI: Cursor Set >> Busy|Idle\")"
            n395 = case shown="\"Idle\", Default" w666 {
              tunnel: w668 -> [w673 w675]
              tunnel: [w672 w674] -> w667
              frame "Idle", Default {
                n396 = call <vilib>:"Unset Busy.vi"("error in (no error)"=w673) -> ("error out"=w672:errorcluster)  [unwired: 10 in]
              }
              frame "Busy" {
                n397 = call <vilib>:"Set Busy.vi"("error in (no error)"=w675) -> ("error out"=w674:errorcluster)  [unwired: 9 in, 1 out]
              }
            }
            n398 = call <vilib>:"Add State(s) to Queue__jki_lib_state_machine.vi"("State(s) in (\"\")"=w671) -> ("States Out"=w670:string)  [unwired: 14 in]
          }
          frame "UI: Front Panel State" {
            # "Argument"
            # "Set Front Panel Open or Closed\n(Usage: \"UI: Front Panel State >> Open|Close\")"
            n399 = Unbundle By Name(w676) -> ("Core.Current VI Reference"=w678:refnum<vi>)
            n400 = case shown="\"Open\", Default" w677 {
              tunnel: w680 -> [w686 w697]
              tunnel: [w687 w698] -> w679
              tunnel: w678 -> [_ _]
              frame "Open", Default {
                n401 = property class="VI"(error in=w686) -> (reference out=w684:refnum<vi>, error out=w685:errorcluster, "Front Panel.Open"=w683:bool)  [unwired: 1 in]
                n402 = case shown="False" w683 {
                  tunnel: [w690 w693] -> w687
                  tunnel: w685 -> [w689 w693]
                  tunnel: w684 -> [w688 _]
                  frame False {
                    n403 = invoke class="VI" method="FP.Open"(reference=w688, error in=w689, "Activate"=TRUE, "State"=T19."Standard") -> (error out=w690:errorcluster)  [unwired: 1 in, 4 out]
                  }
                  frame True {
                  }
                }
              }
              frame "Close" {
                n404 = property class="VI"(error in=w697) -> (reference out=w695:refnum<vi>, error out=w696:errorcluster, "Front Panel.Open"=w694:bool)  [unwired: 1 in]
                n405 = case shown="True" w694 {
                  tunnel: [w699 w702] -> w698
                  tunnel: w696 -> [w699 w701]
                  tunnel: w695 -> [_ w700]
                  frame False {
                  }
                  frame True {
                    n406 = invoke class="VI" method="FP.Close"(reference=w700, error in=w701) -> (error out=w702:errorcluster)  [unwired: 1 in, 2 out]
                  }
                }
              }
            }
            n407 = call <vilib>:"Add State(s) to Queue__jki_lib_state_machine.vi"("State(s) in (\"\")"=w682) -> ("States Out"=w681:string)  [unwired: 14 in]
          }
          frame "---------- Macro ----------" {
            # "Do not put any code in this frame.\n(It is a separator no-op. You can make a copy of this frame to create a new Macro frame)"
            n408 = call <vilib>:"Add State(s) to Queue__jki_lib_state_machine.vi"("State(s) in (\"\")"=w706) -> ("States Out"=w705:string)  [unwired: 14 in]
          }
          frame "Macro: Initialize" {
            w713 = "Data: Initialize\nInitialize Core Data\nUI: Initialize\nUI: Front Panel State >> Open\nDevice Ini >> 3000\nnewtdms"  # Data: Initialize Initialize Core Data UI: Initialize UI: Front Panel State >> Open Device Ini >> 3000 newtdms
            # "Initialization Macro\n(This is called once, when the VI starts)"
            n409 = property on="Img to avg" class="DigNum (strict)"() -> ("Value"=w711:i32)  [unwired: 2 in, 2 out]
            n410 = call <vilib>:"Add State(s) to Queue__jki_lib_state_machine.vi"("State(s) in Front (\"\")"=w713, "State(s) in (\"\")"=w716) -> ("States Out"=w708:string)  [unwired: 13 in]
            n411 = Number To Decimal String(number=w711) -> (decimal integer string=w710:string)  [unwired: 1 in]
            n412 = call <vilib>:"Build State String with Arguments__jki_lib_state_machine.vi"("Arguments (\"\")"=w710, "State"="ImgToAvg") -> ("State with Arguments"=w709:string)  [unwired: 4 in]
            n413 = call <vilib>:"Add State(s) to Queue__jki_lib_state_machine.vi"("State(s) in (\"\")"=w708, "State(s) at Back (\"\")"=w709) -> ("States Out"=w707:string)  [unwired: 13 in]
          }
          frame "Macro: Exit" {
            # "Exit Macro\n(This is called once, when the VI exits)"
            n414 = Unbundle By Name(w718) -> ("Core.Close Panel on Exit?"=w717:bool)
            n415 = Select(t="UI: Front Panel State >> Close", s=w717, f="") -> (s? t:f=w721:string)
            n416 = call <vilib>:"Add State(s) to Queue__jki_lib_state_machine.vi"("State(s) in (\"\")"=w721, "State(s) at Back (\"\")"="Data: Cleanup\nExit") -> ("States Out"=w719:string)  [unwired: 13 in]
            n417 = call <vilib>:"Add State(s) to Queue__jki_lib_state_machine.vi"("State(s) in Front (\"\")"=w719, "State(s) in (\"\")"=w726) -> ("States Out"=w725:string)  [unwired: 13 in]
          }
          frame "---------- Ini and Configure ----------" {
            # "Template Separator\n(You can make a copy of, or modify, this frame)"
            n418 = call <vilib>:"Add State(s) to Queue__jki_lib_state_machine.vi"("State(s) in (\"\")"=w730) -> ("States Out"=w729:string)  [unwired: 14 in]
          }
          frame "Device Ini" {
            # "Your code here.\n(You can make a copy of, or modify, this frame)"
            n419 = Empty String/Path?(string/path=w747) -> (empty?=w745:bool)
            n420 = case shown="False" w745 {
              tunnel: w747 -> [w784 _]
              tunnel: [w783 0] -> w746
              frame False {
                n421 = Decimal String To Number(string=w784) -> (number=w783:i32)  [unwired: 2 in, 1 out]
              }
              frame True {
              }
            }
            n422 = flat-sequence {
              tunnel: w751 -> [w787]
              tunnel: [w787] -> w750
              tunnel: w746 -> [w786]
              tunnel: w750 -> [w790]
              tunnel: [w788] -> w736
              frame #0 {
                n423 = Wait (ms)(milliseconds to wait=w786) -> ()  [unwired: 1 out]
              }
              frame #1 {
                n424 = for {
                  tunnel: w790 -> [w792] mode=indexing
                  shift-right: [w793] -> w788
                  shift-left: string[] [] -> [w794]
                  n425 = Empty String/Path?(string/path=w792) -> (empty?=w791:bool)
                  n426 = case shown="False" w791 {
                    tunnel: w794 -> [w797 w803]
                    tunnel: [w796 w803] -> w793
                    tunnel: w792 -> [w795 _]
                    frame False {
                      n427 = call "send command.vi"("Device Name"=w795) -> ("status"=w798:bool)  [unwired: 4 in]
                      n428 = case shown="True" w798 {
                        tunnel: w797 -> [w799 w802]
                        tunnel: [w799 w801] -> w796
                        tunnel: w795 -> [_ w800]
                        frame False {
                        }
                        frame True {
                          n429 = Build Array (concatenate)(w802, w800) -> (w801:string[])
                        }
                      }
                    }
                    frame True {
                    }
                  }
                }
              }
            }
            n430 = Unbundle By Name(w744) -> ("active cams"=w737:string[])
            n431 = call <vilib>:"Add State(s) to Queue__jki_lib_state_machine.vi"("State(s) in (\"\")"=w752) -> ("States Out"=w739:string)  [unwired: 14 in]
            n432 = Empty Array?(array=w737) -> (empty?=w741:bool)
            n433 = Equal?(x=w737, y=w736) -> (x = y?=w742:bool[])
            n434 = Not(x=w741) -> (.not. x?=w740:bool)
            n435 = Build Array (concatenate)(w742, w740) -> (w743:bool[])
            n436 = Array Size(array=w736) -> (size(s)=w734:i32)
            n437 = Array Size(array=w737) -> (size(s)=w735:i32)
            n438 = Equal?(x=w735, y=w734) -> (x = y?=w733:bool)
            n439 = And Array Elements(Boolean array=w743) -> (logical AND=w732:bool)
            n440 = And(x=w733, y=w732) -> (x .and. y?=w731:bool)
            n441 = case shown="False" w731 {
              tunnel: [w769 w782] -> w749
              tunnel: w744 -> [w754 w782]
              tunnel: w736 -> [w755 _]
              tunnel: w739 -> [w764 w781]
              tunnel: [w762 w781] -> w738
              frame False {
                n442 = Bundle By Name(cluster=w754, "active cams"=w755) -> (w770:T37)
                n443 = property on="active CCDs" class="LstBox (strict)"("Item Names"=w755) -> ()  [unwired: 2 in, 2 out]
                n444 = Array Size(array=w755) -> (size(s)=w773:i32)
                n445 = for {
                  N: 1 -> [_]
                  shift-right: [w775] -> w768
                  shift-left: timestamp[][] [] ("Time") -> [w777]
                  n446 = for {
                    N: 12 -> [_]
                    tunnel: w777 -> [w780] mode=indexing
                    tunnel: [w778] -> w775 mode=indexing
                    n447 = Get Date/Time In Seconds() -> (seconds since 1Jan1904=w779:timestamp)
                    n448 = Build Array (concatenate)(w780, w779) -> (w778:timestamp[])
                  }
                }
                n449 = Unbundle By Name(w754) -> ("img to avg"=w753:i32)
                n450 = Initialize Array(0.0 ("element"), w773, 0 ("dimension size")) -> (w771:dbl[][])
                n451 = Initialize Array(0.0 ("element"), 12 ("dimension size"), w753) -> (w756:dbl[][])
                n452 = Bundle By Name(cluster=w770, "Offset X stats"=w771, "Offset Y stats"=w771, "Centroid X"=w756, "Centroid Y"=w756, "Mean Centroid X"=w771, "Mean Centroid Y"=w771, "Offset X"=w771, "Offset Y"=w771, "Size"=w756, "Mean Size"=w771, "Motor X"=w771, "Motor Y"=w771) -> (w769:T37)
                n453 = property on="Time" class="Arr (strict)"("Value"=w768) -> ()  [unwired: 2 in, 2 out]
                n454 = property on="config path" class="Str"() -> ("Value"=w761:string)  [unwired: 2 in, 2 out]
                n455 = call <vilib>:"Add State(s) to Queue__jki_lib_state_machine.vi"("State(s) in Front (\"\")"="newtdms\nMove Config\nDetection Config\nactive\nCenter" ("State(s) in Front (\"\")"), "State(s) in (\"\")"=w764) -> ("States Out"=w763:string)  [unwired: 13 in]
                n456 = call <vilib>:"Build State String with Arguments__jki_lib_state_machine.vi"("Arguments (\"\")"=w761, "State"="Load Config" ("State(s) in Front (\"\")")) -> ("State with Arguments"=w759:string)  [unwired: 4 in]
                n457 = call <vilib>:"Add State(s) to Queue__jki_lib_state_machine.vi"("State(s) in Front (\"\")"=w759, "State(s) in (\"\")"=w763) -> ("States Out"=w762:string)  [unwired: 13 in]
                "name array" <- w755
              }
              frame True {
              }
            }
          }
          frame "Load Config" {
            # "Your code here.\n(You can make a copy of, or modify, this frame)"
            n458 = Unbundle By Name(w806) -> ("detection para"=w849:T3[], "move properties"=w846:T2[], "thresholds"=w841:cluster{"Lower value":sgl, "Upper value":sgl}[])
            n459 = Empty String/Path?(string/path=w805) -> (empty?=w804:bool)
            n460 = property on="Load Config" class="Bool (strict)"("Value"=FALSE ("Load Config")) -> ()  [unwired: 2 in, 2 out]
            n461 = case shown="False" w804 {
              tunnel: [w860 T5 {"CCDs"=[], "move properties"=[], "detection para"=[], "thresholds"=[], "Value"={"Motor CCD 1"=0, "Motor CCD 2"=0, "Motor CCD 3"=0, "Motor CCD 4"=0, "Motor CCD 5"=0, "Motor CCD 6"=0, "Motor CCD 7"=0, "Motor CCD 8"=0, "Motor CCD 9"=0, "Motor CCD 10"=0, "Motor CCD 11"=0, "Motor CCD 12"=0}} ("output cluster 2")] -> w851
              tunnel: [w858 w867] -> w811
              tunnel: w805 -> [w857 _]
              tunnel: w808 -> [w855 w867]
              tunnel: w806 -> [_ _]
              frame False {
                n462 = String To Path(string=w857) -> (path=w856:path)
                n463 = Open/Create/Replace File(file path (use dialog)=w856, error in=w855, operation (0:open)=T20."open or create") -> (refnum out=w862:refnum<file>, error out=w863:errorcluster)  [unwired: 3 in, 1 out]
                n464 = Read from Binary File(5:"output cluster 2", 8:w863, 11:w862) -> (0:w864:errorcluster, 2:w860:T5, 3:w865:refnum<file>)  [unwired: 3 in, 1 out]
                n465 = Close File(refnum=w865, error in=w864) -> (error out=w858:errorcluster)  [unwired: 1 out]
              }
              frame True {
              }
            }
            n466 = Unbundle By Name(w851) -> ("Value"=w838:T7, "CCDs"=w850:string[], "detection para"=w848:T3[], "move properties"=w847:T2[], "thresholds"=w842:cluster{"Lower value":sgl, "Upper value":sgl}[])
            n467 = Cluster To Array(cluster=w838) -> (array=w839:u16[])
            n468 = call <vilib>:"Add State(s) to Queue__jki_lib_state_machine.vi"("State(s) in (\"\")"=w854, "State(s) at Back (\"\")"="Motor Config" ("State(s) at Back (\"\")")) -> ("States Out"=w853:string)  [unwired: 13 in]
            n469 = for {
              tunnel: w850 -> [w883]
              tunnel: w848 -> [w885]
              tunnel: w847 -> [w884]
              shift-right: [w877] -> w845
              shift-left: w849 -> [w882]
              shift-right: [w875] -> w844
              shift-left: w846 -> [w881]
              tunnel: w807 -> [w880] mode=indexing
              tunnel: w842 -> [w876]
              shift-right: [w872] -> w840
              shift-left: w841 -> [w874]
              tunnel: w839 -> [w871]
              tunnel: [w868] -> w837 mode=indexing
              i -> [w869]
              n470 = call-poly <userlib>:"Filter 1D Array__ogtk.vi"("items to filter"=w880, "array"=w883) -> ("filtered item indices"=w886:i32[])  [unwired: 4 in, 1 out]
              n471 = Index Array(array=w886) -> (element=w870:i32)  [unwired: 1 in]
              n472 = Index Array(array=w871, index=w870) -> (element=w868:u16)
              n473 = Index Array(array=w885, index=w870) -> (element=w879:T3)
              n474 = Index Array(array=w884, index=w870) -> (element=w878:T2)
              n475 = Index Array(array=w876, index=w870) -> (element=w873:cluster{"Lower value":sgl, "Upper value":sgl})
              n476 = Replace Array Subset(array=w882, new element=w879, index=w869) -> (w877:T3[])
              n477 = Replace Array Subset(array=w881, new element=w878, index=w869) -> (w875:T2[])
              n478 = Replace Array Subset(array=w874, new element=w873, index=w869) -> (w872:cluster{"Lower value":sgl, "Upper value":sgl}[])
            }
            n479 = Index Array(array=w837, index #1=0 ("index (row)"), index #2=1 ("index (row)"), index #3=2 ("index (row)"), index #4=3 ("index (row)"), index #5=4 ("index (row)"), index #6=5 ("index (row)"), index #7=6 ("index (row)"), index #8=7 ("index (row)"), index #9=8 ("index (row)"), index #10=9 ("index (row)"), index #11=10 ("index (row)"), index #12=11 ("index (row)")) -> (element #1=w824:u16, element #2=w823:u16, element #3=w822:u16, element #4=w821:u16, element #5=w820:u16, element #6=w819:u16, element #7=w818:u16, element #8=w817:u16, element #9=w816:u16, element #10=w815:u16, element #11=w814:u16, element #12=w813:u16)
            n480 = Bundle By Name(cluster=w838, "Motor CCD 1"=w824, "Motor CCD 2"=w823, "Motor CCD 3"=w822, "Motor CCD 4"=w821, "Motor CCD 5"=w820, "Motor CCD 6"=w819, "Motor CCD 7"=w818, "Motor CCD 8"=w817, "Motor CCD 9"=w816, "Motor CCD 10"=w815, "Motor CCD 11"=w814, "Motor CCD 12"=w813) -> (w812:T7)
            n481 = Bundle By Name(cluster=w806, "detection para"=w845, "move properties"=w844, "thresholds"=w840) -> (w843:T37)
            n482 = property on="associated motors" class="Clust (strict)"(error in=w811, "Val(Sgnl)"=w812) -> (error out=w810:errorcluster)  [unwired: 1 in, 1 out]
          }
          frame "Save Config" {
            # "Your code here.\n(You can make a copy of, or modify, this frame)"
            n483 = Unbundle By Name(w905) -> ("move properties"=w892:T2[], "detection para"=w900:T3[], "thresholds"=w889:cluster{"Lower value":sgl, "Upper value":sgl}[])
            n484 = property on="associated motors" class="Clust (strict)"() -> ("Value"=w899:T7)  [unwired: 2 in, 2 out]
            n485 = property on="Save Config" class="Bool (strict)"("Value"=FALSE ("Save Config")) -> ()  [unwired: 2 in, 2 out]
            n486 = local read "CCDs"() -> (w890:string[])
            n487 = call "File Dialog"("error in"=w888, "pattern (all files)"="*.cfg", "pattern label"="config") -> ("selected path"=w894:path, "error out"=w887:errorcluster)  [unwired: 9 in, 2 out]
            n488 = Bundle("CCDs"=w890, "move properties"=w892, "detection para"=w900, "thresholds"=w889, "Value"=w899) -> (w893:T5)  [unwired: 1 in]
            n489 = Open/Create/Replace File(file path (use dialog)=w894, error in=w887, operation (0:open)=T20."replace or create with confirmation") -> (refnum out=w901:refnum<file>, error out=w902:errorcluster)  [unwired: 3 in, 1 out]
            n490 = Write to Binary File(file (use dialog)=w901, data=w893, error in=w902) -> (refnum out=w904:refnum<file>, error out=w903:errorcluster)  [unwired: 3 in, 1 out]
            n491 = Close File(refnum=w904, error in=w903) -> (error out=w897:errorcluster)  [unwired: 1 out]
            n492 = call <vilib>:"Add State(s) to Queue__jki_lib_state_machine.vi"("State(s) in (\"\")"=w907) -> ("States Out"=w906:string)  [unwired: 14 in]
          }
          frame "active" {
            # "Your code here.\n(You can make a copy of, or modify, this frame)"
            n493 = call-poly <userlib>:"Filter 1D Array__ogtk.vi"("items to filter"=w917, "array"=w913) -> ("filtered item indices"=w916:i32[])  [unwired: 4 in, 1 out]
            n494 = Unbundle By Name(w912) -> ("move properties"=w915:T2[], "detection para"=w910:T3[])  [unwired: 1 out]
            n495 = Index Array(array=w916) -> (element=w908:i32)  [unwired: 1 in]
            n496 = Index Array(array=w915, index=w908) -> (element=w914:T2)
            n497 = Index Array(array=w910, index=w908) -> (element=w909:T3)
            n498 = property on="move config" class="Clust (strict)"("Value"=w914) -> ()  [unwired: 2 in, 2 out]
            n499 = property on="beam detection para" class="Clust (strict)"("Value"=w909) -> ()  [unwired: 2 in, 2 out]
            n500 = Bundle By Name(cluster=w912, "active ccd"=w908) -> (w911:T37)
            n501 = call <vilib>:"Add State(s) to Queue__jki_lib_state_machine.vi"("State(s) in (\"\")"=w920) -> ("States Out"=w919:string)  [unwired: 14 in]
          }
          frame "Detection Config" {
            # "Your code here.\n(You can make a copy of, or modify, this frame)"
            n502 = Unbundle By Name(w925) -> ("detection para"=w921:T3[], "active ccd"=w926:i32)
            n503 = Replace Array Subset(array=w921, new element="beam detection para", index=w926) -> (w922:T3[])
            n504 = Bundle By Name(cluster=w925, "detection para"=w922) -> (w924:T37)
            n505 = call <vilib>:"Add State(s) to Queue__jki_lib_state_machine.vi"("State(s) in (\"\")"=w929) -> ("States Out"=w928:string)  [unwired: 14 in]
          }
          frame "Motor Config" {
            # "Your code here.\n(You can make a copy of, or modify, this frame)"
            n506 = Unbundle By Name("associated motors") -> ("Motor CCD 1"=w951:u16, "Motor CCD 2"=w952:u16, "Motor CCD 3"=w953:u16, "Motor CCD 4"=w946:u16, "Motor CCD 5"=w945:u16, "Motor CCD 6"=w944:u16, "Motor CCD 7"=w943:u16, "Motor CCD 8"=w942:u16, "Motor CCD 9"=w941:u16, "Motor CCD 10"=w940:u16, "Motor CCD 11"=w939:u16, "Motor CCD 12"=w938:u16)
            n507 = local read "motor refs"() -> (w949:refnum<vi>[])
            n508 = property on="ActiveMotor" class="Ring (strict)"() -> ("Value"=w932:u16)  [unwired: 2 in, 2 out]
            n509 = property on="ActiveMotor" class="Ring (strict)"() -> ("Strings []"=w934:string[])  [unwired: 2 in, 2 out]
            n510 = Build Array(w951, w952, w953, w946, w945, w944, w943, w942, w941, w940, w939, w938) -> (w937:u16[])
            n511 = Increment(x=w937) -> (x+1=w936:u16[])
            n512 = Index Array(array=w934, index=w932) -> (element=w933:string)
            n513 = for {
              tunnel: w936 -> [w968] mode=indexing
              tunnel: w949 -> [w963]
              tunnel: [w959] -> w935 mode=indexing
              tunnel: [w958] -> w931 mode=indexing
              tunnel: [w957] -> w930 mode=indexing
              n514 = Multiply(x=w968, y=u16 3) -> (x*y=w964:u16)
              n515 = Subtract(x=w964, y=u16 3) -> (x-y=w958:u16)
              n516 = Subtract(x=w964, y=u16 2) -> (x-y=w957:u16)
              n517 = Index Array(array=w963, index=w958) -> (element=w962:refnum<vi>)
              n518 = Index Array(array=w963, index=w957) -> (element=w961:refnum<vi>)
              n519 = Bundle By Name(cluster="active Axis ref", "Ref X"=w962, "Ref Y"=w961) -> (w959:cluster{"Ref X":refnum<vi>, "Ref Y":refnum<vi>})
            }
            "Array" <- w931
            "Array 2" <- w930
            n520 = property on="ActiveMotorName::99" class="Str"("Val(Sgnl)"=w933) -> ()  [unwired: 2 in, 2 out]
            n521 = call <vilib>:"Add State(s) to Queue__jki_lib_state_machine.vi"("State(s) in (\"\")"=w956) -> ("States Out"=w955:string)  [unwired: 14 in]
            n522 = Bundle By Name(cluster=w948, "active axis refs 2"=w935) -> (w947:T37)
          }
          frame "Move Config" {
            # "Your code here.\n(You can make a copy of, or modify, this frame)"
            n523 = Unbundle By Name(w970) -> ("move properties"=w974:T2[], "active ccd"=w973:i32)
            n524 = Replace Array Subset(array=w974, new element="move config", index=w973) -> (w971:T2[])
            n525 = Bundle By Name(cluster=w970, "move properties"=w971) -> (w969:T37)
            n526 = call <vilib>:"Add State(s) to Queue__jki_lib_state_machine.vi"("State(s) in (\"\")"=w977) -> ("States Out"=w976:string)  [unwired: 14 in]
          }
          frame "----------Centroid & Move----------" {
            # "Template Separator\n(You can make a copy of, or modify, this frame)"
            n527 = call <vilib>:"Add State(s) to Queue__jki_lib_state_machine.vi"("State(s) in (\"\")"=w981) -> ("States Out"=w980:string)  [unwired: 14 in]
          }
          frame "detected" {
            n528 = Unbundle By Name(w984) -> ("Offset X"=w1026:dbl[][], "Offset Y"=w1025:dbl[][], "Size"=w1024:dbl[][], "Mean Size"=w1023:dbl[][], "Time"=w1020:timestamp[][], "Motor X"=w998:dbl[][], "active axis refs 2"=w997:T12, "Motor Y"=w996:dbl[][])
            n529 = Spreadsheet String To Array(format string="%s", spreadsheet string=w1002, array type (2D Dbl)=string[] []) -> (array=w991:string[])  [unwired: 1 in]
            n530 = call-poly <userlib>:"Filter 1D Array__ogtk.vi"("items to filter"=w991, "array"=w992) -> ("filtered item indices"=w989:i32[])  [unwired: 4 in, 1 out]
            n531 = for {
              tunnel: w992 -> [w1043] mode=indexing
              tunnel: w991 -> [w1042]
              tunnel: [w1040] -> w993 mode=indexing
              n532 = for {
                tunnel: w1043 -> [w1046]
                tunnel: [w1045] -> w1041 mode=indexing
                tunnel: w1042 -> [w1044] mode=indexing
                n533 = Equal?(x=w1046, y=w1044) -> (x = y?=w1045:bool)
              }
              n534 = Or Array Elements(Boolean array=w1041) -> (logical OR=w1040:bool)
            }
            n535 = for {
              N: 12 -> [_]
              tunnel: w989 -> [w1039]
              tunnel: [w1036] -> w988 mode=indexing
              i -> [w1038]
              n536 = Equal?(x=w1039, y=w1038) -> (x = y?=w1037:bool[])
              n537 = Or Array Elements(Boolean array=w1037) -> (logical OR=w1036:bool)
            }
            "Array 3" <- w988
            n538 = call <vilib>:"Build State String with Arguments__jki_lib_state_machine.vi"("Arguments (\"\")"=w1002, "State"="stats") -> ("State with Arguments"=w1001:string)  [unwired: 4 in]
            n539 = Unbundle By Name(w984) -> ("Mean Centroid X"=w1031:dbl[][], "Mean Centroid Y"=w1030:dbl[][], "Centroid X"=w1033:dbl[][], "Centroid Y"=w1032:dbl[][])
            n540 = call <vilib>:"Add State(s) to Queue__jki_lib_state_machine.vi"("State(s) in (\"\")"=w1000, "State(s) at Back (\"\")"=w1001) -> ("States Out"=w999:string)  [unwired: 13 in]
            n541 = for {
              tunnel: w1033 -> [w1096]
              tunnel: w1032 -> [w1095]
              tunnel: w1031 -> [w1094]
              tunnel: w1030 -> [w1093]
              tunnel: [w1092] -> w1017 mode=indexing
              tunnel: [w1091] -> w1028 mode=indexing
              tunnel: w1027 -> [w1064] mode=indexing
              tunnel: w1026 -> [w1090]
              tunnel: w1025 -> [w1089]
              tunnel: [w1088] -> w1005 mode=indexing
              tunnel: [w1087] -> w1018 mode=indexing
              tunnel: w1024 -> [w1086]
              tunnel: w1023 -> [w1085]
              tunnel: [w1084] -> w1022 mode=indexing
              tunnel: w1020 -> [w1083]
              tunnel: [w1082] -> w1019 mode=indexing
              tunnel: w998 -> [w1056]
              tunnel: w997 -> [w1055]
              tunnel: w996 -> [w1054]
              tunnel: [w1053] -> w995 mode=indexing
              tunnel: [w1052] -> w994 mode=indexing
              tunnel: w993 -> [w1051]
              i -> [w1050]
              n542 = Unbundle By Name(w1064) -> ("Target.X::12"=w1067:refnum<vi>, "Target.Y::12"=w1066:refnum<vi>)
              n543 = Index Array(array=w1056, index (row)=w1050) -> (element=w1059:dbl[])  [unwired: 1 in]
              n544 = Index Array(array=w1055, index=w1050) -> (element=w1058:cluster{"Ref X":refnum<vi>, "Ref Y":refnum<vi>})
              n545 = Index Array(array=w1054, index (row)=w1050) -> (element=w1063:dbl[])  [unwired: 1 in]
              n546 = Index Array(array=w1094, index (row)=w1050) -> (element=w1078:dbl[])  [unwired: 1 in]
              n547 = Index Array(array=w1093, index (row)=w1050) -> (element=w1079:dbl[])  [unwired: 1 in]
              n548 = Index Array(array=w1096, index (row)=w1050) -> (element=w1081:dbl[])  [unwired: 1 in]
              n549 = Index Array(array=w1095, index (row)=w1050) -> (element=w1080:dbl[])  [unwired: 1 in]
              n550 = Index Array(array=w1090, index (row)=w1050) -> (element=w1075:dbl[])  [unwired: 1 in]
              n551 = Index Array(array=w1089, index (row)=w1050) -> (element=w1074:dbl[])  [unwired: 1 in]
              n552 = Index Array(array=w1086, index (row)=w1050) -> (element=w1072:dbl[])  [unwired: 1 in]
              n553 = Index Array(array=w1085, index (row)=w1050) -> (element=w1071:dbl[])  [unwired: 1 in]
              n554 = Index Array(array=w1083, index (row)=w1050) -> (element=w1068:timestamp[])  [unwired: 1 in]
              n555 = Index Array(array=w1051, index=w1050) -> (element=w1049:bool)
              n556 = Unbundle By Name(w1058) -> ("Ref X"=w1057:refnum<vi>, "Ref Y"=w1061:refnum<vi>)
              n557 = property class="DigNum (strict)"(reference=w1067) -> ("Value"=w1048:dbl)  [unwired: 1 in, 2 out]
              n558 = property class="DigNum (strict)"(reference=w1066) -> ("Value"=w1065:dbl)  [unwired: 1 in, 2 out]
              n559 = call <vilib>:"Std Deviation and Variance.vi"("X"=w1081) -> ("mean"=w1047:dbl)  [unwired: 1 in, 2 out]
              n560 = call <vilib>:"Std Deviation and Variance.vi"("X"=w1080) -> ("mean"=w1077:dbl)  [unwired: 1 in, 2 out]
              n561 = call <vilib>:"Std Deviation and Variance.vi"("X"=w1072) -> ("mean"=w1070:dbl)  [unwired: 1 in, 2 out]
              n562 = Get Date/Time In Seconds() -> (seconds since 1Jan1904=w1069:timestamp)
              n563 = property class="DigNum (strict)"(reference=w1057) -> ("Value"=w1060:dbl)  [unwired: 1 in, 2 out]
              n564 = property class="DigNum (strict)"(reference=w1061) -> ("Value"=w1062:dbl)  [unwired: 1 in, 2 out]
              n565 = Subtract(x=w1048, y=w1047) -> (x-y=w1076:dbl)
              n566 = Subtract(x=w1065, y=w1077) -> (x-y=w1073:dbl)
              n567 = case shown="True" w1049 {
                tunnel: [w1114 w1128] -> w1092
                tunnel: [w1113 w1127] -> w1091
                tunnel: [w1112 w1126] -> w1088
                tunnel: [w1111 w1125] -> w1087
                tunnel: [w1110 w1124] -> w1084
                tunnel: [w1109 w1123] -> w1082
                tunnel: w1079 -> [w1108 w1122]
                tunnel: w1078 -> [w1107 w1121]
                tunnel: w1047 -> [w1106 _]
                tunnel: w1077 -> [w1105 _]
                tunnel: w1076 -> [w1104 _]
                tunnel: w1075 -> [w1103 w1120]
                tunnel: w1074 -> [w1102 w1119]
                tunnel: w1073 -> [w1101 _]
                tunnel: w1071 -> [w1100 w1118]
                tunnel: w1070 -> [w1099 _]
                tunnel: w1069 -> [w1098 w1117]
                tunnel: w1068 -> [w1097 w1116]
                frame True {
                  n568 = Build Array (concatenate)(w1107, w1106) -> (w1114:dbl[])
                  n569 = Build Array (concatenate)(w1108, w1105) -> (w1113:dbl[])
                  n570 = Build Array (concatenate)(w1103, w1104) -> (w1112:dbl[])
                  n571 = Build Array (concatenate)(w1102, w1101) -> (w1111:dbl[])
                  n572 = Build Array (concatenate)(w1100, w1099) -> (w1110:dbl[])
                  n573 = Build Array (concatenate)(w1097, w1098) -> (w1109:timestamp[])
                }
                frame False {
                  w1115 = 0.0
                  n574 = Build Array (concatenate)(w1121, w1115) -> (w1128:dbl[])
                  n575 = Build Array (concatenate)(w1122, w1115) -> (w1127:dbl[])
                  n576 = Build Array (concatenate)(w1120, w1115) -> (w1126:dbl[])
                  n577 = Build Array (concatenate)(w1119, w1115) -> (w1125:dbl[])
                  n578 = Build Array (concatenate)(w1118, w1115) -> (w1124:dbl[])
                  n579 = Build Array (concatenate)(w1116, w1117) -> (w1123:timestamp[])
                }
              }
              n580 = Build Array (concatenate)(w1063, w1062) -> (w1052:dbl[])
              n581 = Build Array (concatenate)(w1059, w1060) -> (w1053:dbl[])
            }
            n582 = local write "Numeric"(0.0 ("Numeric")) -> ()
            n583 = Array Size(array=w1005) -> (size(s)=w1016:i32[])
            n584 = Index Array(array=w1016, index=1) -> (element=w1014:i32)
            "History index" <- w1014
            n585 = call <vilib>:"Add State(s) to Queue__jki_lib_state_machine.vi"("State(s) in (\"\")"=w999, "State(s) at Back (\"\")"="Check Move\ntdms" ("State(s) at Back (\"\")")) -> ("States Out"=w1008:string)  [unwired: 13 in]
            n586 = Unbundle By Name(w984) -> ("img to avg"=w983:i32)
            n587 = Decrement(x=w983) -> (x-1=w982:i32)
            n588 = Initialize Array(0.0 ("element"), 12 ("dimension size"), w982) -> (w985:dbl[][])
            n589 = Greater?(x=w1014, y="History Size") -> (0:w1012:bool)
            n590 = Bundle By Name(cluster=w984, "Centroid X"=w985, "Centroid Y"=w985, "Mean Centroid X"=w1017, "Mean Centroid Y"=w1028, "Offset X"=w1005, "Offset Y"=w1018, "Mean Size"=w1022, "Size"=w985, "Time"=w1019, "Motor X"=w995, "Motor Y"=w994) -> (w1029:T37)
            n591 = Select(t="history" ("State(s) at Back (\"\")"), s=w1012, f="") -> (s? t:f=w1009:string)
            n592 = call <vilib>:"Add State(s) to Queue__jki_lib_state_machine.vi"("State(s) in (\"\")"=w1008, "State(s) at Back (\"\")"=w1009) -> ("States Out"=w1007:string)  [unwired: 13 in]
          }
          frame "Check Move" {
            (unwired) "Device Ini" ("State(s) in Front (\"\")")
            # "Your code here.\n(You can make a copy of, or modify, this frame)"
            n593 = Unbundle By Name(w1133) -> ("move properties"=w1136:T2[], "Mean Size"=w1159:dbl[][], "move properties"=w1162:T2[], "Offset X"=w1161:dbl[][], "Offset Y"=w1160:dbl[][], "active cams"=w1140:string[])
            n594 = for {
              tunnel: w1162 -> [w1227]
              tunnel: w1161 -> [w1226]
              tunnel: w1160 -> [w1225]
              tunnel: w1159 -> [w1228]
              tunnel: [w1244] -> w1158 mode=indexing
              tunnel: [w1240] -> w1157 mode=indexing
              tunnel: w1140 -> [w1230] mode=indexing
              tunnel: [w1262] -> w1156 mode=indexing
              tunnel: [w1261] -> w1155 mode=indexing
              tunnel: w1136 -> [w1220]
              tunnel: [w1238] -> w1134 mode=indexing
              tunnel: [w1233] -> w1130 mode=indexing
              tunnel: "Speedmode @" -> [w1232]
              tunnel: w1129 -> [w1231]
              n595 = call-poly <userlib>:"Filter 1D Array__ogtk.vi"("items to filter"=w1230, "array"=w1231) -> ("filtered item indices"=w1229:i32[])  [unwired: 4 in, 1 out]
              n596 = Index Array(array=w1229) -> (element=w1219:i32)  [unwired: 1 in]
              n597 = Index Array(array=w1228, index (row)=w1219) -> (element=w1224:dbl[])  [unwired: 1 in]
              n598 = Index Array(array=w1227, index=w1219) -> (element=w1223:T2)
              n599 = Index Array(array=w1226, index (row)=w1219) -> (element=w1222:dbl[])  [unwired: 1 in]
              n600 = Index Array(array=w1220, index=w1219) -> (element=w1218:T2)
              n601 = Index Array(array=w1225, index (row)=w1219) -> (element=w1221:dbl[])  [unwired: 1 in]
              n602 = Unbundle By Name(w1223) -> ("Tolerance [%]"=w1255:dbl)
              n603 = Reverse 1D Array(array=w1222) -> (reversed array=w1260:dbl[])
              n604 = Reverse 1D Array(array=w1221) -> (reversed array=w1259:dbl[])
              n605 = Reverse 1D Array(array=w1224) -> (reversed array=w1254:dbl[])
              n606 = Unbundle By Name(w1218) -> ("enable feedback"=w1243:bool)
              n607 = Index Array(array=w1260) -> (element=w1258:dbl)  [unwired: 1 in]
              n608 = Index Array(array=w1259) -> (element=w1257:dbl)  [unwired: 1 in]
              n609 = Index Array(array=w1254) -> (element=w1253:dbl)  [unwired: 1 in]
              n610 = Absolute Value(x=w1258) -> (abs(x)=w1239:dbl)
              n611 = Absolute Value(x=w1257) -> (abs(x)=w1236:dbl)
              n612 = Square Root(x=w1253) -> (sqrt(x)=w1252:dbl)
              n613 = Divide(x=w1255, y=100.0) -> (x/y=w1251:dbl)
              n614 = Multiply(x=w1252, y=w1251) -> (x*y=w1235:dbl)
              n615 = Not Equal To 0?(x=w1236) -> (x != 0?=w1241:bool)
              n616 = Not Equal To 0?(x=w1239) -> (x != 0?=w1246:bool)
              n617 = Greater Or Equal?(x=w1239, y=w1235) -> (x >= y?=w1245:bool)
              n618 = Greater Or Equal?(x=w1236, y=w1235) -> (x >= y?=w1242:bool)
              n619 = Divide(x=w1239, y=w1235) -> (x/y=w1237:dbl)
              n620 = Divide(x=w1236, y=w1235) -> (x/y=w1234:dbl)
              n621 = Compound Arithmetic op=AND(w1243, w1246, w1245) -> (w1244:bool)
              n622 = Compound Arithmetic op=AND(w1243, w1242, w1241) -> (w1240:bool)
              n623 = Boolean To (0,1)(Boolean=w1240) -> (0, 1=w1247:i16)
              n624 = Greater?(x=w1237, y=w1232) -> (0:w1238:bool)
              n625 = Greater?(x=w1234, y=w1232) -> (0:w1233:bool)
              n626 = Multiply(x=w1247, y=w1236) -> (x*y=w1248:dbl)
              n627 = Boolean To (0,1)(Boolean=w1244) -> (0, 1=w1250:i16)
              n628 = Multiply(x=w1250, y=w1239) -> (x*y=w1249:dbl)
              n629 = Bundle(w1248, "GUIdevice 8"=w1230) -> (w1261:cluster{dbl, "GUIdevice 8":string})  [unwired: 1 in]
              n630 = Bundle(w1249, "GUIdevice 8"=w1230) -> (w1262:cluster{dbl, "GUIdevice 8":string})  [unwired: 1 in]
            }
            "required X" <- w1158
            "required Y" <- w1157
            "speedmode X" <- w1134
            "speedmode Y" <- w1130
            n631 = case shown="True" "Align" {
              tunnel: w1156 -> [w1170 w1175]
              tunnel: w1155 -> [w1169 w1172]
              tunnel: [w1168 w1174] -> w1152
              tunnel: [w1167 w1171] -> w1146
              frame False {
                n632 = Sort 1D Array(array=w1169) -> (sorted array=w1166:cluster{dbl, "GUIdevice 8":string}[])
                n633 = Sort 1D Array(array=w1170) -> (sorted array=w1165:cluster{dbl, "GUIdevice 8":string}[])
                n634 = Reverse 1D Array(array=w1166) -> (reversed array=w1167:cluster{dbl, "GUIdevice 8":string}[])
                n635 = Reverse 1D Array(array=w1165) -> (reversed array=w1168:cluster{dbl, "GUIdevice 8":string}[])
              }
              frame True {
                w1173 = cluster{dbl, "GUIdevice 8":string}[] [] ("Array")
                n636 = for {
                  shift-right: [w1185] -> w1174
                  shift-left: w1173 -> [w1187]
                  tunnel: w1175 -> [w1186] mode=indexing
                  n637 = Unbundle(w1186) -> (w1189:dbl)  [unwired: 1 out]
                  n638 = Not Equal To 0?(x=w1189) -> (x != 0?=w1188:bool)
                  n639 = case shown="True" w1188 {
                    tunnel: w1187 -> [w1190 w1193]
                    tunnel: w1186 -> [_ w1192]
                    tunnel: [w1190 w1191] -> w1185
                    frame False {
                    }
                    frame True {
                      n640 = Build Array (concatenate)(w1193, w1192) -> (w1191:cluster{dbl, "GUIdevice 8":string}[])
                    }
                  }
                }
                n641 = for {
                  shift-right: [w1176] -> w1171
                  shift-left: w1173 -> [w1178]
                  tunnel: w1172 -> [w1177] mode=indexing
                  n642 = Unbundle(w1177) -> (w1180:dbl)  [unwired: 1 out]
                  n643 = Not Equal To 0?(x=w1180) -> (x != 0?=w1179:bool)
                  n644 = case shown="True" w1179 {
                    tunnel: w1178 -> [w1181 w1184]
                    tunnel: w1177 -> [_ w1183]
                    tunnel: [w1181 w1182] -> w1176
                    frame False {
                    }
                    frame True {
                      n645 = Build Array (concatenate)(w1184, w1183) -> (w1182:cluster{dbl, "GUIdevice 8":string}[])
                    }
                  }
                }
              }
            }
            n646 = call <vilib>:"Add State(s) to Queue__jki_lib_state_machine.vi"("State(s) in (\"\")"=w1139) -> ("States Out"=w1138:string)  [unwired: 14 in]
            n647 = Bundle By Name(cluster=w1133, "speedmode X"=w1134, "speedmode Y"=w1130) -> (w1132:T37)
            n648 = Empty Array?(array=w1152) -> (empty?=w1149:bool)
            n649 = Empty Array?(array=w1146) -> (empty?=w1144:bool)
            n650 = Index Array(array=w1152) -> (element=w1142:cluster{dbl, "GUIdevice 8":string})  [unwired: 1 in]
            n651 = Index Array(array=w1146) -> (element=w1141:cluster{dbl, "GUIdevice 8":string})  [unwired: 1 in]
            n652 = Unbundle(w1142) -> (w1151:dbl)  [unwired: 1 out]
            n653 = Unbundle(w1141) -> (w1147:dbl)  [unwired: 1 out]
            n654 = Equal To 0?(x=w1151) -> (x = 0?=w1150:bool)
            n655 = Equal To 0?(x=w1147) -> (x = 0?=w1145:bool)
            n656 = property on="autodetect" class="Bool (strict)"("Value"=FALSE ("autodetect")) -> ()  [unwired: 2 in, 2 out]
            n657 = Unbundle By Name(w1132) -> ("Feedback global"=w1153:bool)
            n658 = Or(x=w1150, y=w1149) -> (x .or. y?=w1148:bool)
            n659 = Or(x=w1145, y=w1144) -> (x .or. y?=w1143:bool)
            n660 = case shown="True" w1153 {
              tunnel: w1148 -> [_ w1201]
              tunnel: w1152 -> [_ w1200]
              tunnel: w1143 -> [_ w1198]
              tunnel: w1146 -> [_ w1197]
              tunnel: w1138 -> [w1194 w1196]
              tunnel: [w1194 w1195] -> w1154
              frame False {
              }
              frame True {
                n661 = case shown="False" w1201 {
                  tunnel: w1200 -> [w1216 _]
                  tunnel: w1196 -> [w1212 w1217]
                  tunnel: [w1210 w1217] -> w1199
                  frame False {
                    n662 = Index Array(array=w1216) -> (element=w1215:cluster{dbl, "GUIdevice 8":string})  [unwired: 1 in]
                    n663 = Unbundle By Name(w1215) -> ("GUIdevice 8"=w1214:string)
                    n664 = call <vilib>:"Build State String with Arguments__jki_lib_state_machine.vi"("Arguments (\"\")"=w1214, "State"="Move X") -> ("State with Arguments"=w1211:string)  [unwired: 4 in]
                    n665 = call <vilib>:"Add State(s) to Queue__jki_lib_state_machine.vi"("State(s) in (\"\")"=w1212, "State(s) at Back (\"\")"=w1211) -> ("States Out"=w1210:string)  [unwired: 13 in]
                  }
                  frame True {
                  }
                }
                n666 = case shown="False" w1198 {
                  tunnel: w1197 -> [w1208 _]
                  tunnel: w1199 -> [w1204 w1209]
                  tunnel: [w1202 w1209] -> w1195
                  frame False {
                    n667 = Index Array(array=w1208) -> (element=w1207:cluster{dbl, "GUIdevice 8":string})  [unwired: 1 in]
                    n668 = Unbundle By Name(w1207) -> ("GUIdevice 8"=w1206:string)
                    n669 = call <vilib>:"Build State String with Arguments__jki_lib_state_machine.vi"("Arguments (\"\")"=w1206, "State"="Move Y") -> ("State with Arguments"=w1203:string)  [unwired: 4 in]
                    n670 = call <vilib>:"Add State(s) to Queue__jki_lib_state_machine.vi"("State(s) in (\"\")"=w1204, "State(s) at Back (\"\")"=w1203) -> ("States Out"=w1202:string)  [unwired: 13 in]
                  }
                  frame True {
                  }
                }
              }
            }
            n671 = call <vilib>:"Add State(s) to Queue__jki_lib_state_machine.vi"("State(s) in (\"\")"=w1138, "State(s) at Back (\"\")"=w1154) -> ("States Out"=w1164:string)  [unwired: 13 in]
          }
          frame "Move X" {
            # "Your code here.\n(You can make a copy of, or modify, this frame)"
            n672 = Unbundle By Name(w1286) -> ("Offset X"=w1263:dbl[][])
            n673 = call-poly <userlib>:"Filter 1D Array__ogtk.vi"("items to filter"=w1271, "array"=w1290) -> ("filtered item indices"=w1275:i32[])  [unwired: 4 in, 1 out]
            n674 = Unbundle By Name(w1286) -> ("speedmode X"=w1270:bool[], "active axis refs 2"=w1289:T12, "move properties"=w1274:T2[])
            n675 = for {
              tunnel: w1275 -> [w1295] mode=indexing
              tunnel: w1274 -> [w1299]
              shift-right: [w1294] -> w1272
              shift-left: i32[] [] ("filtered item indices") -> [w1297]
              n676 = Index Array(array=w1299, index=w1295) -> (element=w1298:T2)
              n677 = Unbundle By Name(w1298) -> ("enable feedback"=w1296:bool)
              n678 = case shown="True" w1296 {
                tunnel: w1297 -> [w1300 w1303]
                tunnel: w1295 -> [_ w1302]
                tunnel: [w1300 w1301] -> w1294
                frame False {
                }
                frame True {
                  n679 = Build Array (concatenate)(w1303, w1302) -> (w1301:i32[])
                }
              }
            }
            n680 = Index Array(array=w1272) -> (element=w1269:i32)  [unwired: 1 in]
            n681 = Index Array(array=w1263, index (row)=w1269) -> (element=w1285:dbl[])  [unwired: 1 in]
            n682 = Reverse 1D Array(array=w1285) -> (reversed array=w1284:dbl[])
            n683 = Index Array(array=w1289, index=w1269) -> (element=w1288:cluster{"Ref X":refnum<vi>, "Ref Y":refnum<vi>})
            n684 = Index Array(array=w1284) -> (element=w1282:dbl)  [unwired: 1 in]
            n685 = Index Array(array=w1274, index=w1269) -> (element=w1287:T2)
            n686 = Unbundle By Name(w1288) -> ("Ref X"=w1279:refnum<vi>, "Ref Y"=w1278:refnum<vi>)
            n687 = Index Array(array=w1270, index=w1269) -> (element=w1268:bool)
            n688 = Unbundle By Name(w1287) -> ("Invert Direction X"=w1280:bool, "Invert Axis"=w1283:bool, "Stepsize"=w1266:dbl, "enable feedback"=w1277:bool)
            n689 = Greater Or Equal To 0?(x=w1282) -> (x >= 0?=w1281:bool)
            n690 = call <vilib>:"Add State(s) to Queue__jki_lib_state_machine.vi"("State(s) in Front (\"\")"="Wait" ("State(s) in Front (\"\")"), "State(s) in (\"\")"=w1293) -> ("States Out"=w1292:string)  [unwired: 13 in]
            n691 = property on="Speedmode @" class="DigNum (strict)"() -> ("Value"=w1265:dbl)  [unwired: 2 in, 2 out]
            n692 = Multiply(x=w1265, y=w1266) -> (x*y=w1267:dbl)
            n693 = Select(t=w1267, s=w1268, f=w1266) -> (s? t:f=w1264:dbl)
            n694 = case shown="True" w1277 {
              tunnel: w1283 -> [_ w1309]
              tunnel: w1281 -> [_ w1308]
              tunnel: w1264 -> [_ w1307]
              tunnel: w1280 -> [_ w1306]
              tunnel: w1279 -> [_ w1305]
              tunnel: w1278 -> [_ w1304]
              frame False {
              }
              frame True {
                n695 = case shown="False" w1308 {
                  tunnel: w1306 -> [w1317 w1339]
                  tunnel: w1307 -> [w1315 w1337]
                  tunnel: w1309 -> [w1314 w1336]
                  tunnel: w1309 -> [w1313 w1335]
                  tunnel: w1305 -> [w1311 w1333]
                  tunnel: w1304 -> [w1310 w1332]
                  frame True {
                    n696 = case shown="False" w1314 {
                      tunnel: [w1328 w1330] -> w1316
                      tunnel: w1311 -> [w1329 _]
                      tunnel: w1310 -> [_ w1331]
                      frame False {
                        n697 = property class="DigNum (strict)"(reference=w1329) -> ("Value"=w1328:dbl)  [unwired: 1 in, 2 out]
                      }
                      frame True {
                        n698 = property class="DigNum (strict)"(reference=w1331) -> ("Value"=w1330:dbl)  [unwired: 1 in, 2 out]
                      }
                    }
                    n699 = case shown="False" w1317 {
                      tunnel: w1316 -> [w1324 w1327]
                      tunnel: w1315 -> [w1323 w1326]
                      tunnel: [w1322 w1325] -> w1312
                      frame False {
                        n700 = Add(x=w1324, y=w1323) -> (x+y=w1322:dbl)
                      }
                      frame True {
                        n701 = Subtract(x=w1327, y=w1326) -> (x-y=w1325:dbl)
                      }
                    }
                    n702 = case shown="False" w1313 {
                      tunnel: w1312 -> [w1318 w1320]
                      tunnel: w1311 -> [w1319 _]
                      tunnel: w1310 -> [_ w1321]
                      frame False {
                        n703 = property class="DigNum (strict)"(reference=w1319, "Val(Sgnl)"=w1318) -> ()  [unwired: 1 in, 2 out]
                      }
                      frame True {
                        n704 = property class="DigNum (strict)"(reference=w1321, "Val(Sgnl)"=w1320) -> ()  [unwired: 1 in, 2 out]
                      }
                    }
                  }
                  frame False {
                    n705 = case shown="False" w1336 {
                      tunnel: [w1350 w1352] -> w1338
                      tunnel: w1333 -> [w1351 _]
                      tunnel: w1332 -> [_ w1353]
                      frame False {
                        n706 = property class="DigNum (strict)"(reference=w1351) -> ("Value"=w1350:dbl)  [unwired: 1 in, 2 out]
                      }
                      frame True {
                        n707 = property class="DigNum (strict)"(reference=w1353) -> ("Value"=w1352:dbl)  [unwired: 1 in, 2 out]
                      }
                    }
                    n708 = case shown="False" w1339 {
                      tunnel: w1338 -> [w1346 w1349]
                      tunnel: w1337 -> [w1345 w1348]
                      tunnel: [w1344 w1347] -> w1334
                      frame False {
                        n709 = Subtract(x=w1346, y=w1345) -> (x-y=w1344:dbl)
                      }
                      frame True {
                        n710 = Add(x=w1349, y=w1348) -> (x+y=w1347:dbl)
                      }
                    }
                    n711 = case shown="False" w1335 {
                      tunnel: w1334 -> [w1340 w1342]
                      tunnel: w1333 -> [w1341 _]
                      tunnel: w1332 -> [_ w1343]
                      frame False {
                        n712 = property class="DigNum (strict)"(reference=w1341, "Val(Sgnl)"=w1340) -> ()  [unwired: 1 in, 2 out]
                      }
                      frame True {
                        n713 = property class="DigNum (strict)"(reference=w1343, "Val(Sgnl)"=w1342) -> ()  [unwired: 1 in, 2 out]
                      }
                    }
                  }
                }
              }
            }
            "Arguments X" <- w1271
            "Moving X" <- w1271
          }
          frame "Move Y" {
            # "Your code here.\n(You can make a copy of, or modify, this frame)"
            n714 = Unbundle By Name(w1377) -> ("Offset Y"=w1376:dbl[][])
            n715 = call-poly <userlib>:"Filter 1D Array__ogtk.vi"("items to filter"=w1361, "array"=w1381) -> ("filtered item indices"=w1366:i32[])  [unwired: 4 in, 1 out]
            n716 = Unbundle By Name(w1377) -> ("speedmode Y"=w1360:bool[], "active axis refs 2"=w1380:T12, "move properties"=w1364:T2[])
            n717 = for {
              tunnel: w1366 -> [w1386] mode=indexing
              tunnel: w1364 -> [w1390]
              shift-right: [w1385] -> w1365
              shift-left: i32[] [] ("filtered item indices") -> [w1388]
              n718 = Index Array(array=w1390, index=w1386) -> (element=w1389:T2)
              n719 = Unbundle By Name(w1389) -> ("enable feedback"=w1387:bool)
              n720 = case shown="True" w1387 {
                tunnel: w1388 -> [w1391 w1394]
                tunnel: w1386 -> [_ w1393]
                tunnel: [w1391 w1392] -> w1385
                frame False {
                }
                frame True {
                  n721 = Build Array (concatenate)(w1394, w1393) -> (w1392:i32[])
                }
              }
            }
            n722 = Index Array(array=w1365) -> (element=w1359:i32)  [unwired: 1 in]
            n723 = Index Array(array=w1376, index (row)=w1359) -> (element=w1375:dbl[])  [unwired: 1 in]
            n724 = Reverse 1D Array(array=w1375) -> (reversed array=w1374:dbl[])
            n725 = Index Array(array=w1380, index=w1359) -> (element=w1379:cluster{"Ref X":refnum<vi>, "Ref Y":refnum<vi>})
            n726 = Index Array(array=w1374) -> (element=w1372:dbl)  [unwired: 1 in]
            n727 = Index Array(array=w1364, index=w1359) -> (element=w1378:T2)
            n728 = Index Array(array=w1360, index=w1359) -> (element=w1358:bool)
            n729 = Unbundle By Name(w1379) -> ("Ref Y"=w1369:refnum<vi>, "Ref X"=w1368:refnum<vi>)
            n730 = Unbundle By Name(w1378) -> ("Invert Direction Y"=w1370:bool, "Invert Axis"=w1373:bool, "Stepsize"=w1356:dbl, "enable feedback"=w1367:bool)
            n731 = Greater Or Equal To 0?(x=w1372) -> (x >= 0?=w1371:bool)
            n732 = call <vilib>:"Add State(s) to Queue__jki_lib_state_machine.vi"("State(s) in Front (\"\")"="Wait" ("State(s) in Front (\"\")"), "State(s) in (\"\")"=w1384) -> ("States Out"=w1383:string)  [unwired: 13 in]
            n733 = property on="Speedmode @" class="DigNum (strict)"() -> ("Value"=w1355:dbl)  [unwired: 2 in, 2 out]
            n734 = Multiply(x=w1355, y=w1356) -> (x*y=w1354:dbl)
            n735 = Select(t=w1354, s=w1358, f=w1356) -> (s? t:f=w1357:dbl)
            n736 = case shown="True" w1367 {
              tunnel: w1373 -> [_ w1400]
              tunnel: w1371 -> [_ w1399]
              tunnel: w1357 -> [_ w1398]
              tunnel: w1370 -> [_ w1397]
              tunnel: w1369 -> [_ w1396]
              tunnel: w1368 -> [_ w1395]
              frame False {
              }
              frame True {
                n737 = case shown="True" w1399 {
                  tunnel: w1397 -> [w1408 w1430]
                  tunnel: w1398 -> [w1406 w1428]
                  tunnel: w1400 -> [w1405 w1427]
                  tunnel: w1400 -> [w1404 w1426]
                  tunnel: w1396 -> [w1402 w1424]
                  tunnel: w1395 -> [w1401 w1423]
                  frame True {
                    n738 = case shown="False" w1405 {
                      tunnel: [w1419 w1421] -> w1407
                      tunnel: w1402 -> [w1420 _]
                      tunnel: w1401 -> [_ w1422]
                      frame False {
                        n739 = property class="DigNum (strict)"(reference=w1420) -> ("Value"=w1419:dbl)  [unwired: 1 in, 2 out]
                      }
                      frame True {
                        n740 = property class="DigNum (strict)"(reference=w1422) -> ("Value"=w1421:dbl)  [unwired: 1 in, 2 out]
                      }
                    }
                    n741 = case shown="False" w1408 {
                      tunnel: w1407 -> [w1415 w1418]
                      tunnel: w1406 -> [w1414 w1417]
                      tunnel: [w1413 w1416] -> w1403
                      frame False {
                        n742 = Add(x=w1415, y=w1414) -> (x+y=w1413:dbl)
                      }
                      frame True {
                        n743 = Subtract(x=w1418, y=w1417) -> (x-y=w1416:dbl)
                      }
                    }
                    n744 = case shown="False" w1404 {
                      tunnel: w1403 -> [w1409 w1411]
                      tunnel: w1402 -> [w1410 _]
                      tunnel: w1401 -> [_ w1412]
                      frame False {
                        n745 = property class="DigNum (strict)"(reference=w1410, "Val(Sgnl)"=w1409) -> ()  [unwired: 1 in, 2 out]
                      }
                      frame True {
                        n746 = property class="DigNum (strict)"(reference=w1412, "Val(Sgnl)"=w1411) -> ()  [unwired: 1 in, 2 out]
                      }
                    }
                  }
                  frame False {
                    n747 = case shown="False" w1427 {
                      tunnel: [w1441 w1443] -> w1429
                      tunnel: w1424 -> [w1442 _]
                      tunnel: w1423 -> [_ w1444]
                      frame False {
                        n748 = property class="DigNum (strict)"(reference=w1442) -> ("Value"=w1441:dbl)  [unwired: 1 in, 2 out]
                      }
                      frame True {
                        n749 = property class="DigNum (strict)"(reference=w1444) -> ("Value"=w1443:dbl)  [unwired: 1 in, 2 out]
                      }
                    }
                    n750 = case shown="False" w1430 {
                      tunnel: w1429 -> [w1437 w1440]
                      tunnel: w1428 -> [w1436 w1439]
                      tunnel: [w1435 w1438] -> w1425
                      frame False {
                        n751 = Subtract(x=w1437, y=w1436) -> (x-y=w1435:dbl)
                      }
                      frame True {
                        n752 = Add(x=w1440, y=w1439) -> (x+y=w1438:dbl)
                      }
                    }
                    n753 = case shown="False" w1426 {
                      tunnel: w1425 -> [w1431 w1433]
                      tunnel: w1424 -> [w1432 _]
                      tunnel: w1423 -> [_ w1434]
                      frame False {
                        n754 = property class="DigNum (strict)"(reference=w1432, "Val(Sgnl)"=w1431) -> ()  [unwired: 1 in, 2 out]
                      }
                      frame True {
                        n755 = property class="DigNum (strict)"(reference=w1434, "Val(Sgnl)"=w1433) -> ()  [unwired: 1 in, 2 out]
                      }
                    }
                  }
                }
              }
            }
            "Arguments Y" <- w1361
            "Moving Y" <- w1361
          }
          frame "Wait" {
            # "Your code here.\n(You can make a copy of, or modify, this frame)"
            n756 = flat-sequence {
              frame #0 {
                n757 = Wait (ms)(milliseconds to wait=u32 300) -> ()  [unwired: 1 out]
              }
              frame #1 {
                n758 = property on="Moving Y" class="Str"("Value"="") -> ()  [unwired: 2 in, 2 out]
                n759 = property on="Moving X" class="Str"("Value"="") -> ()  [unwired: 2 in, 2 out]
              }
            }
            n760 = call <vilib>:"Add State(s) to Queue__jki_lib_state_machine.vi"("State(s) in (\"\")"=w1450) -> ("States Out"=w1449:string)  [unwired: 14 in]
            n761 = local read "Mean Centroid X"() -> (w1445:dbl[][])
            n762 = Bundle By Name(cluster=w1447, "Mean Centroid X"=w1445, "Mean Centroid Y"=w1445) -> (w1446:T37)
          }
          frame "stats" {
            # "Your code here.\n(You can make a copy of, or modify, this frame)"
            n763 = Unbundle By Name(w1459) -> ("Offset X"=w1458:dbl[][], "Offset Y"=w1457:dbl[][], "Time"=w1456:timestamp[][], "Motor X"=w1455:dbl[][], "Motor Y"=w1454:dbl[][])
            n764 = for {
              tunnel: w1457 -> [w1497]
              tunnel: w1456 -> [w1498]
              tunnel: w1458 -> [w1499]
              tunnel: [w1502] -> w1485 mode=indexing
              tunnel: w1455 -> [w1496]
              tunnel: w1454 -> [w1495]
              tunnel: w1460 -> [_] mode=indexing
              i -> [w1489]
              n765 = Index Array(array=w1497, index (row)=w1489) -> (element=w1493:dbl[])  [unwired: 1 in]
              n766 = Index Array(array=w1496, index (row)=w1489) -> (element=w1491:dbl[])  [unwired: 1 in]
              n767 = Index Array(array=w1495, index (row)=w1489) -> (element=w1490:dbl[])  [unwired: 1 in]
              n768 = Index Array(array=w1499, index (row)=w1489) -> (element=w1494:dbl[])  [unwired: 1 in]
              n769 = Index Array(array=w1498, index (row)=w1489) -> (element=w1492:timestamp[])  [unwired: 1 in]
              n770 = Bundle("Time"=w1492, "Motor X"=w1491) -> (w1501:cluster{"Time":timestamp[], "Motor X":dbl[]})  [unwired: 1 in]
              n771 = Bundle("Time"=w1492, "Motor Y"=w1490) -> (w1500:cluster{"Time":timestamp[], "Motor Y":dbl[]})  [unwired: 1 in]
              n772 = Bundle("Time"=w1492, "Offset X"=w1494) -> (w1503:cluster{"Time":timestamp[], "Offset X":dbl[]})  [unwired: 1 in]
              n773 = Bundle("Time"=w1492, "Offset Y"=w1493) -> (w1504:cluster{"Time":timestamp[], "Offset Y":dbl[]})  [unwired: 1 in]
              n774 = Build Array(w1504, w1503, w1501, w1500) -> (w1502:cluster{"Time":timestamp[], "Motor Y":dbl[]}[])
            }
            n775 = call <vilib>:"Add State(s) to Queue__jki_lib_state_machine.vi"("State(s) in (\"\")"=w1488) -> ("States Out"=w1487:string)  [unwired: 14 in]
            n776 = Index Array(array=w1485, index (row) #1=0 ("index (row)"), index (row) #2=1 ("index (row)"), index (row) #3=2 ("index (row)"), index (row) #4=3 ("index (row)"), index (row) #5=4 ("index (row)"), index (row) #6=5 ("index (row)"), index (row) #7=6 ("index (row)"), index (row) #8=7 ("index (row)"), index (row) #9=8 ("index (row)"), index (row) #10=9 ("index (row)"), index (row) #11=10 ("index (row)"), index (row) #12=11 ("index (row)")) -> (element #1=→"CCD 1":cluster{"Time":timestamp[], "Motor Y":dbl[]}[], element #2=→"CCD 2":cluster{"Time":timestamp[], "Motor Y":dbl[]}[], element #3=→"CCD 3":cluster{"Time":timestamp[], "Motor Y":dbl[]}[], element #4=→"CCD 4":cluster{"Time":timestamp[], "Motor Y":dbl[]}[], element #5=→"CCD 5":cluster{"Time":timestamp[], "Motor Y":dbl[]}[], element #6=→"CCD 6":cluster{"Time":timestamp[], "Motor Y":dbl[]}[], element #7=→"CCD 7":cluster{"Time":timestamp[], "Motor Y":dbl[]}[], element #8=→"CCD 8":cluster{"Time":timestamp[], "Motor Y":dbl[]}[], element #9=→"CCD 9":cluster{"Time":timestamp[], "Motor Y":dbl[]}[], element #10=→"CCD 10":cluster{"Time":timestamp[], "Motor Y":dbl[]}[], element #11=→"CCD 11":cluster{"Time":timestamp[], "Motor Y":dbl[]}[], element #12=→"CCD 12":cluster{"Time":timestamp[], "Motor Y":dbl[]}[])  [unwired: 12 in]
          }
          frame "---------------Statistics--------------" {
            # "Template Separator\n(You can make a copy of, or modify, this frame)"
            n777 = call <vilib>:"Add State(s) to Queue__jki_lib_state_machine.vi"("State(s) in (\"\")"=w1508) -> ("States Out"=w1507:string)  [unwired: 14 in]
          }
          frame "Save Stats" {
            # "Your code here.\n(You can make a copy of, or modify, this frame)"
            n778 = property on="CCD 1" class="XYGraph (strict)"() -> ("Value"=w1518:cluster{timestamp[], dbl[]}[])  [unwired: 2 in, 2 out]
            n779 = property on="CCD 2" class="XYGraph (strict)"() -> ("Value"=w1517:cluster{timestamp[], dbl[]}[])  [unwired: 2 in, 2 out]
            n780 = property on="CCD 3" class="XYGraph (strict)"() -> ("Value"=w1516:cluster{timestamp[], dbl[]}[])  [unwired: 2 in, 2 out]
            n781 = property on="CCD 4" class="XYGraph (strict)"() -> ("Value"=w1515:cluster{timestamp[], dbl[]}[])  [unwired: 2 in, 2 out]
            n782 = property on="CCD 5" class="XYGraph (strict)"() -> ("Value"=w1514:cluster{timestamp[], dbl[]}[])  [unwired: 2 in, 2 out]
            n783 = property on="CCD 6" class="XYGraph (strict)"() -> ("Value"=w1513:cluster{timestamp[], dbl[]}[])  [unwired: 2 in, 2 out]
            n784 = property on="CCD 7" class="XYGraph (strict)"() -> ("Value"=w1512:cluster{timestamp[], dbl[]}[])  [unwired: 2 in, 2 out]
            n785 = property on="CCD 8" class="XYGraph (strict)"() -> ("Value"=w1511:cluster{timestamp[], dbl[]}[])  [unwired: 2 in, 2 out]
            n786 = Build Array(w1518, w1517, w1516, w1515, w1514, w1513, w1512, w1511) -> (w1510:cluster{timestamp[], dbl[]}[][])
            n787 = for {
              tunnel: w1510 -> [w1526] mode=indexing
              tunnel: w1509 -> [w1525] mode=indexing
              n788 = Empty String/Path?(string/path=w1525) -> (empty?=w1524:bool)
              n789 = case shown="False" w1524 {
                tunnel: w1526 -> [w1532 _]
                tunnel: w1525 -> [w1530 _]
                frame False {
                  n790 = Index Array(array=w1532, index #1=0 ("index"), index #2=1 ("index"), index #3=2 ("index"), index #4=3 ("index")) -> (element #1=w1567:cluster{timestamp[], dbl[]}, element #2=w1561:cluster{timestamp[], dbl[]}, element #3=w1560:cluster{timestamp[], dbl[]}, element #4=w1559:cluster{timestamp[], dbl[]})  [unwired: 1 in, 1 out]
                  n791 = Concatenate Strings(w1530, ".dat" ("string")) -> (w1528:string)
                  n792 = Unbundle(w1567) -> (w1566:timestamp[], w1544:dbl[])
                  n793 = Unbundle(w1561) -> (w1535:dbl[])  [unwired: 1 out]
                  n794 = Unbundle(w1560) -> (w1534:dbl[])  [unwired: 1 out]
                  n795 = Unbundle(w1559) -> (w1533:dbl[])  [unwired: 1 out]
                  n796 = Build Path(base path="save path", name or relative path=w1528) -> (appended path=w1527:path)
                  n797 = for {
                    tunnel: w1566 -> [w1569] mode=indexing
                    tunnel: [w1568] -> w1542 mode=indexing
                    n798 = Format Date/Time String(time format string (%c)="%Y%m%d%H%M%S", seconds (now)=w1569) -> (date/time string=w1568:string)  [unwired: 1 in]
                  }
                  n799 = Array Size(array=w1544) -> (size(s)=w1545:i32)
                  n800 = Number To Fractional String(number=w1544) -> (F-format string=w1541:string[])  [unwired: 3 in]
                  n801 = Number To Fractional String(number=w1535) -> (F-format string=w1538:string[])  [unwired: 3 in]
                  n802 = Number To Fractional String(number=w1534) -> (F-format string=w1537:string[])  [unwired: 3 in]
                  n803 = Number To Fractional String(number=w1533) -> (F-format string=w1536:string[])  [unwired: 3 in]
                  n804 = Initialize Array("", w1545, 5 ("dimension size")) -> (w1543:string[][])
                  n805 = Insert Into Array(array=w1543, index (col)=0 ("disabled index (col)"), new element=w1542) -> (w1553:string[][])  [unwired: 1 in]
                  n806 = Insert Into Array(array=w1553, index (col)=1 ("disabled index (col)"), new element=w1541) -> (w1552:string[][])  [unwired: 1 in]
                  n807 = Insert Into Array(array=w1552, index (col)=2 ("disabled index (col)"), new element=w1538) -> (w1556:string[][])  [unwired: 1 in]
                  n808 = Insert Into Array(array=w1556, index (col)=3 ("disabled index (col)"), new element=w1537) -> (w1557:string[][])  [unwired: 1 in]
                  n809 = Insert Into Array(array=w1557, index (col)=4 ("disabled index (col)"), new element=w1536) -> (w1558:string[][])  [unwired: 1 in]
                  n810 = Insert Into Array(array=w1558, index (row)=0, new element=string[] ["time", "Centroid X", "Centroid Y", "Motor Axis 1", "Motor Axis 2"] ("new element/subarray 2")) -> (w1540:string[][])  [unwired: 1 in]
                  n811 = call-poly <vilib>:"Write To Spreadsheet File.vi"("2D data"=w1540, "file path (dialog if empty)"=w1527) -> ()  [unwired: 6 in, 1 out]
                }
                frame True {
                }
              }
            }
            n812 = call <vilib>:"Add State(s) to Queue__jki_lib_state_machine.vi"("State(s) in (\"\")"=w1523) -> ("States Out"=w1522:string)  [unwired: 14 in]
            n813 = property on="Save Stats" class="Bool (strict)"("Value"=FALSE ("Save Stats")) -> ()  [unwired: 2 in, 2 out]
          }
          frame "tdms" {
            w1596 = 21600.0 ("new tdms")
            # "Your code here.\n(You can make a copy of, or modify, this frame)"
            n814 = Unbundle By Name(w1586) -> ("Data Value Reference out"=w1609:refnum<k34>, "Offset X"=w1611:dbl[][], "Offset Y"=w1606:dbl[][], "active axis refs 2"=w1608:T12)
            n815 = for {
              tunnel: w1611 -> [w1655]
              tunnel: w1606 -> [w1654]
              tunnel: w1610 -> [w1618] mode=indexing
              tunnel: w1609 -> [w1619]
              tunnel: w1608 -> [w1640]
              tunnel: w1607 -> [w1624]
              tunnel: [w1622] -> w1605
              i -> [w1641]
              n816 = Index Array(array=w1655, index (row)=w1641) -> (element=w1653:dbl[])  [unwired: 1 in]
              n817 = Index Array(array=w1654, index (row)=w1641) -> (element=w1652:dbl[])  [unwired: 1 in]
              n818 = Index Array(array=w1640, index=w1641) -> (element=w1639:cluster{"Ref X":refnum<vi>, "Ref Y":refnum<vi>})
              n819 = Reverse 1D Array(array=w1652) -> (reversed array=w1650:dbl[])
              n820 = Reverse 1D Array(array=w1653) -> (reversed array=w1651:dbl[])
              n821 = Unbundle By Name(w1639) -> ("Ref X"=w1638:refnum<vi>, "Ref Y"=w1637:refnum<vi>)
              n822 = Index Array(array=w1651) -> (element=w1649:dbl)  [unwired: 1 in]
              n823 = Index Array(array=w1650) -> (element=w1648:dbl)  [unwired: 1 in]
              n824 = property class="DigNum (strict)"(reference=w1638, error in=w1624) -> (error out=w1623:errorcluster, "Value"=w1632:dbl)  [unwired: 1 out]
              n825 = Build Array(w1649) -> (w1621:dbl[])
              n826 = Build Array(w1648) -> (w1643:dbl[])
              n827 = Get Date/Time In Seconds() -> (seconds since 1Jan1904=w1620:timestamp)
              n828 = Build Array(w1620) -> (w1616:timestamp[])
              n829 = property class="DigNum (strict)"(reference=w1637, error in=w1623) -> (error out=w1614:errorcluster, "Value"=w1626:dbl)  [unwired: 1 out]
              n830 = Build Array(w1632) -> (w1631:dbl[])
              n831 = TDMS Write(0:w1619, 5:w1618, 7:"time", 9:w1616, 11:w1614) -> (4:w1615:refnum<k34>, 15:w1613:errorcluster)  [unwired: 1 in, 2 out]
              n832 = Build Array(w1626) -> (w1625:dbl[])
              n833 = TDMS Write(0:w1615, 5:w1618, 7:"centroid X", 9:w1621, 11:w1613) -> (4:w1646:refnum<k34>, 6:w1645:string, 15:w1644:errorcluster)  [unwired: 1 in, 1 out]
              n834 = TDMS Write(0:w1646, 5:w1645, 7:"centroid Y", 9:w1643, 11:w1644) -> (4:w1635:refnum<k34>, 6:w1634:string, 15:w1636:errorcluster)  [unwired: 1 in, 1 out]
              n835 = TDMS Write(0:w1635, 5:w1634, 7:"Motor Axis 1", 9:w1631, 11:w1636) -> (4:w1630:refnum<k34>, 6:w1629:string, 15:w1627:errorcluster)  [unwired: 1 in, 1 out]
              n836 = TDMS Write(0:w1630, 5:w1629, 7:"Motor Axis 2", 9:w1625, 11:w1627) -> (15:w1622:errorcluster)  [unwired: 1 in, 3 out]
            }
            n837 = Unbundle By Name(w1586) -> ("img to avg"=w1584:i32)
            n838 = property on="millisecond timer value" class="DigNum (strict)"() -> ("Value"=w1573:u32)  [unwired: 2 in, 2 out]
            n839 = local read "millisecond timer 2"() -> (w1602:u32)
            n840 = Tick Count (ms)() -> (millisecond timer value=w1587:u32)
            n841 = call <userlib>:"Tick Count (ms)__ogtk.vi"("error in (no error)"=w1605) -> ("error out"=w1572:errorcluster, "millisecond timer value"=w1604:u32)  [unwired: 9 in]
            n842 = Subtract(x=w1587, y=w1573) -> (x-y=w1601:u32)
            n843 = Subtract(x=w1587, y=w1573) -> (x-y=w1588:u32)
            n844 = Subtract(x=w1604, y=w1602) -> (x-y=→"Waveform Chart":u32)
            n845 = Multiply(x=5.0 ("new tdms"), y=w1584) -> (x*y=w1582:dbl)
            n846 = Divide(x=w1601, y=u32 1000) -> (x/y=w1599:dbl)
            n847 = Divide(x=w1588, y=u32 1000) -> (x/y=w1590:dbl)
            n848 = Quotient & Remainder(x=w1599, y=w1596) -> (x-y*floor(x/y)=w1598:dbl)  [unwired: 1 out]
            n849 = Quotient & Remainder(x=w1590, y=w1582) -> (x-y*floor(x/y)=w1583:dbl)  [unwired: 1 out]
            "x-y*floor(x/y)" <- w1583
            n850 = Subtract(x=w1582, y=2.0) -> (x-y=w1580:dbl)
            n851 = Greater?(x=w1583, y=w1580) -> (0:w1579:bool)
            n852 = call <vilib>:"Clear Errors.vi"("error in (no error)"=w1572) -> ("error out"=w1571:errorcluster)  [unwired: 5 in, 1 out]
            n853 = Subtract(x=w1596, y=20.0) -> (x-y=w1594:dbl)
            n854 = Greater?(x=w1598, y=w1594) -> (0:w1597:bool)
            n855 = Select(t="Device Ini", s=w1579, f="") -> (s? t:f=w1576:string)
            n856 = Select(t="newtdms", s=w1597, f="") -> (s? t:f=w1591:string)
            n857 = call <vilib>:"Add State(s) to Queue__jki_lib_state_machine.vi"("State(s) in (\"\")"=w1612, "State(s) at Back (\"\")"=w1591) -> ("States Out"=w1575:string)  [unwired: 13 in]
            n858 = call <vilib>:"Add State(s) to Queue__jki_lib_state_machine.vi"("State(s) in Front (\"\")"=w1576, "State(s) in (\"\")"=w1575) -> ("States Out"=w1574:string)  [unwired: 13 in]
          }
          frame "Reset History" {
            # "Your code here.\n(You can make a copy of, or modify, this frame)"
            n859 = for {
              N: 1 -> [_]
              shift-right: [w1665] -> w1657
              shift-left: timestamp[][] [] ("Time") -> [w1667]
              n860 = for {
                N: 12 -> [_]
                tunnel: w1667 -> [w1670] mode=indexing
                tunnel: [w1668] -> w1665 mode=indexing
                n861 = Get Date/Time In Seconds() -> (seconds since 1Jan1904=w1669:timestamp)
                n862 = Build Array (concatenate)(w1670, w1669) -> (w1668:timestamp[])
              }
            }
            n863 = local read "Offset X"() -> (w1656:dbl[][])
            n864 = Bundle By Name(cluster=w1661, "Offset X"=w1656, "Offset Y"=w1656, "Time"=w1657, "Motor X"=w1656) -> (w1660:T37)
            n865 = call <vilib>:"Add State(s) to Queue__jki_lib_state_machine.vi"("State(s) in (\"\")"=w1664) -> ("States Out"=w1663:string)  [unwired: 14 in]
          }
          frame "New Category: 2" {
            # "Your code here.\n(You can make a copy of, or modify, this frame)"
            n866 = call <vilib>:"Add State(s) to Queue__jki_lib_state_machine.vi"("State(s) in (\"\")"=w1674) -> ("States Out"=w1673:string)  [unwired: 14 in]
          }
          frame "ImgToAvg" {
            # "Your code here.\n(You can make a copy of, or modify, this frame)"
            n867 = Decimal String To Number(string=w1678) -> (number=w1675:i32)  [unwired: 2 in, 1 out]
            n868 = Bundle By Name(cluster=w1677, "img to avg"=w1675) -> (w1676:T37)
            n869 = call <vilib>:"Add State(s) to Queue__jki_lib_state_machine.vi"("State(s) in (\"\")"=w1681) -> ("States Out"=w1680:string)  [unwired: 14 in]
          }
          frame "newtdms" {
            # "Your code here.\n(You can make a copy of, or modify, this frame)"
            n870 = Unbundle By Name(w1702) -> ("Data Value Reference out"=w1701:refnum<k34>, "active cams"=w1696:string[])
            n871 = TDMS Close(8:w1700, 11:w1701) -> (0:w1683:errorcluster)  [unwired: 1 out]
            n872 = Get Date/Time In Seconds() -> (seconds since 1Jan1904=w1694:timestamp)
            n873 = Format Date/Time String(time format string (%c)="%Y%m%d", seconds (now)=w1694) -> (date/time string=w1692:string)  [unwired: 1 in]
            n874 = Format Date/Time String(time format string (%c)="%Y%m%d%H%M", seconds (now)=w1694) -> (date/time string=w1704:string)  [unwired: 1 in]
            n875 = call <vilib>:"Clear Errors.vi"("error in (no error)"=w1683) -> ("error out"=w1682:errorcluster)  [unwired: 5 in, 1 out]
            n876 = Build Path(base path=w1693, name or relative path=w1692) -> (appended path=w1691:path)
            n877 = Concatenate Strings(w1704, "Beampointing_Pico.tdms" ("string")) -> (w1710:string)
            n878 = String To Path(string=w1710) -> (path=w1711:path)
            n879 = call <vilib>:"Check if File or Folder Exists.vi"("error in (no error)"=w1682, "path"=w1691) -> ("error out"=w1687:errorcluster, "file or folder exists?"=w1690:bool, "dup path"=w1689:path)  [unwired: 7 in]
            n880 = case shown="False" w1690 {
              tunnel: w1689 -> [w1718 w1720]
              tunnel: [w1717 w1720] -> w1688
              tunnel: w1687 -> [w1716 w1719]
              tunnel: [w1715 w1719] -> w1686
              frame False {
                n881 = Create Folder(path (use dialog)=w1718, error in=w1716) -> (created path=w1717:path, error out=w1715:errorcluster)  [unwired: 1 in, 1 out]
              }
              frame True {
              }
            }
            n882 = call <vilib>:"Add State(s) to Queue__jki_lib_state_machine.vi"("State(s) in (\"\")"=w1714) -> ("States Out"=w1713:string)  [unwired: 14 in]
            n883 = Build Path(base path=w1688, name or relative path=w1711) -> (appended path=w1705:path)
            n884 = TDMS Open(6:FALSE ("disable buffering (T)"), 7:enum16{"1.0", "2.0"}."2.0" ("file format version (2.0)"), 8:w1686, 10:T18."create or replace" ("operation"), 11:w1705) -> (0:w1697:errorcluster, 3:w1699:refnum<k34>)  [unwired: 2 in]
            n885 = call "TDMSbuffersize.vi"("error in (no error)"=w1697, "group names"=w1696, "Data Value Reference in"=w1699) -> ("error out"=w1685:errorcluster, "Data Value Reference out"=w1698:refnum<k34>)  [unwired: 7 in]
            n886 = Bundle By Name(cluster=w1702, "Data Value Reference out"=w1698) -> (w1703:T37)
            n887 = call <vilib>:"Clear Errors.vi"("error in (no error)"=w1685) -> ("error out"=w1684:errorcluster)  [unwired: 5 in, 1 out]
          }
          frame "Center" {
            # "Your code here.\n(You can make a copy of, or modify, this frame)"
            n888 = property on="Center" class="Bool (strict)"("Value"=FALSE ("Center")) -> ()  [unwired: 2 in, 2 out]
            n889 = control-ref of="image::1"() -> (w1735:refnum<vi>)
            n890 = control-ref of="image::2"() -> (w1734:refnum<vi>)
            n891 = control-ref of="image::3"() -> (w1733:refnum<vi>)
            n892 = control-ref of="image::4"() -> (w1732:refnum<vi>)
            n893 = control-ref of="image::5"() -> (w1731:refnum<vi>)
            n894 = control-ref of="image::6"() -> (w1730:refnum<vi>)
            n895 = control-ref of="image::7"() -> (w1729:refnum<vi>)
            n896 = control-ref of="image::8"() -> (w1728:refnum<vi>)
            n897 = control-ref of="image::9"() -> (w1727:refnum<vi>)
            n898 = control-ref of="image::10"() -> (w1726:refnum<vi>)
            n899 = control-ref of="image::11"() -> (w1725:refnum<vi>)
            n900 = control-ref of="image::12"() -> (w1724:refnum<vi>)
            n901 = for {
              tunnel: w1721 -> [w1748] mode=indexing
              tunnel: [w1743] -> w1736 mode=indexing
              n902 = Unbundle By Name(w1748) -> ("Target.X::12"=w1747:refnum<vi>, "Target.Y::12"=w1746:refnum<vi>)
              n903 = property class="DigNum (strict)"(reference=w1747) -> ("Value"=w1745:dbl)  [unwired: 1 in, 2 out]
              n904 = property class="DigNum (strict)"(reference=w1746) -> ("Value"=w1744:dbl)  [unwired: 1 in, 2 out]
              n905 = Bundle("Value"=w1745, "Value"=w1744) -> (w1743:cluster{"Value":dbl, "Value":dbl})  [unwired: 1 in]
            }
            n906 = call <vilib>:"Add State(s) to Queue__jki_lib_state_machine.vi"("State(s) in (\"\")"=w1740) -> ("States Out"=w1739:string)  [unwired: 14 in]
            n907 = Build Array(w1735, w1734, w1733, w1732, w1731, w1730, w1729, w1728, w1727, w1726, w1725, w1724) -> (w1723:refnum<vi>[])
            n908 = for {
              tunnel: w1723 -> [w1742] mode=indexing
              tunnel: w1736 -> [w1741] mode=indexing
              n909 = property class="ImageControl"(reference=w1742, "Image Center Position"=w1741) -> ()  [unwired: 1 in, 2 out]
            }
          }
          frame "history" {
            # "Your code here.\n(You can make a copy of, or modify, this frame)"
            n910 = Unbundle By Name(w1758) -> ("Offset X"=w1764:dbl[][], "Offset Y"=w1763:dbl[][], "Mean Centroid X"=w1762:dbl[][], "Mean Centroid Y"=w1761:dbl[][], "Motor X"=w1760:dbl[][], "Motor Y"=w1759:dbl[][], "Time"=w1750:timestamp[][])
            n911 = for {
              tunnel: w1764 -> [w1782] mode=indexing
              tunnel: w1763 -> [w1780] mode=indexing
              tunnel: w1762 -> [w1779] mode=indexing
              tunnel: w1761 -> [w1778] mode=indexing
              tunnel: w1760 -> [w1777] mode=indexing
              tunnel: w1759 -> [w1776] mode=indexing
              tunnel: [w1781] -> w1756 mode=indexing
              tunnel: [w1775] -> w1755 mode=indexing
              tunnel: [w1771] -> w1754 mode=indexing
              tunnel: [w1774] -> w1753 mode=indexing
              tunnel: [w1773] -> w1752 mode=indexing
              tunnel: [w1772] -> w1751 mode=indexing
              tunnel: w1750 -> [w1770] mode=indexing
              tunnel: [w1768] -> w1749 mode=indexing
              w1769 = 0
              n912 = Delete From Array(array=w1777, index=w1769) -> (array with subset deleted=w1773:dbl[])  [unwired: 1 in, 1 out]
              n913 = Delete From Array(array=w1776, index=w1769) -> (array with subset deleted=w1772:dbl[])  [unwired: 1 in, 1 out]
              n914 = Delete From Array(array=w1770, index=w1769) -> (array with subset deleted=w1768:timestamp[])  [unwired: 1 in, 1 out]
              n915 = Delete From Array(array=w1779, index=w1769) -> (array with subset deleted=w1771:dbl[])  [unwired: 1 in, 1 out]
              n916 = Delete From Array(array=w1778, index=w1769) -> (array with subset deleted=w1774:dbl[])  [unwired: 1 in, 1 out]
              n917 = Delete From Array(array=w1780, index=w1769) -> (array with subset deleted=w1775:dbl[])  [unwired: 1 in, 1 out]
              n918 = Delete From Array(array=w1782, index=w1769) -> (array with subset deleted=w1781:dbl[])  [unwired: 1 in, 1 out]
            }
            n919 = call <vilib>:"Add State(s) to Queue__jki_lib_state_machine.vi"("State(s) in (\"\")"=w1767) -> ("States Out"=w1766:string)  [unwired: 14 in]
            n920 = Bundle By Name(cluster=w1758, "Offset X"=w1756, "Offset Y"=w1755, "Mean Centroid X"=w1754, "Mean Centroid Y"=w1753, "Motor X"=w1752, "Motor Y"=w1751, "Time"=w1749) -> (w1757:T37)
          }
        }
        n921 = property on="Box" class="Arr (strict)"() -> ("Value"=w264:T6)  [unwired: 2 in, 2 out]
        n922 = for {
          tunnel: w266 -> [w292]
          tunnel: w265 -> [w293]
          tunnel: w257 -> [w287] mode=indexing
          tunnel: w264 -> [w288] mode=indexing
          tunnel: w254 -> [w284]
          (unwired) cluster{"xhair size":dbl, "xhair size 2":dbl} {"xhair size"=25.0, "xhair size 2"=25.0} ("size")
          (unwired) u32 16774656 ("Color")
          n923 = call-poly <userlib>:"Filter 1D Array__ogtk.vi"("items to filter"=w287, "array"=w293) -> ("filtered item indices"=w294:i32[])  [unwired: 4 in, 1 out]
          n924 = Index Array(array=w294) -> (element=w290:i32)  [unwired: 1 in]
          n925 = Index Array(array=w292, index=w290) -> (element=w291:T31)
          n926 = Unbundle By Name(w291) -> ("Target.X::12"=w296:refnum<vi>, "Target.Y::12"=w295:refnum<vi>)
          n927 = property class="DigNum (strict)"(reference=w296) -> ("Value"=w283:dbl)  [unwired: 1 in, 2 out]
          n928 = property class="DigNum (strict)"(reference=w295) -> ("Value"=w281:dbl)  [unwired: 1 in, 2 out]
          n929 = Bundle By Name(cluster=w284, "Target.x"=w283, "Target.y"=w281) -> (w282:T14)
          n930 = call "draw crosshair imaq.vi"("Crosshair"=w282, "Bounding Rectangle"=T16 {"Left"=0, "Top"=0, "Right"=0, "Bottom"=0}, "image in"=w287) -> ("error out"=→"error out":errorcluster, "image out"=w286:T9)  [unwired: 7 in]
          n931 = call "draw box imaq.vi"("Color"=u32 1244928, "Rectangle"=w288, "image in"=w286) -> ()  [unwired: 7 in, 2 out]
        }
        n932 = property on="ActiveMotor" class="Ring (strict)"() -> ("Strings []"=w259:string[])  [unwired: 2 in, 2 out]
        n933 = Index Array(array=w259, index="ActiveMotor") -> (element=w260:string)
        n934 = Not Equal?(x="ActiveMotorName::99", y=w260) -> (x != y?=w261:bool)
        n935 = case shown="True" w261 {
          tunnel: w259 -> [_ w280]
          tunnel: "ActiveMotorName::99" -> [_ w279]
          frame False {
          }
          frame True {
            n936 = Search 1D Array(1D array=w280, element=w279) -> (index of element=w278:i32)  [unwired: 1 in]
            n937 = property on="ActiveMotor" class="Ring (strict)"("Value"=w278) -> ()  [unwired: 2 in, 2 out]
          }
        }
      }
      n938 = control-ref of="This Application"() -> (w245:refnum<vi>)
      n939 = control-ref of="This VI"() -> (w249:refnum<vi>)
      n940 = Current VI's Menubar() -> (w248:refnum<k9>)
      n941 = call "GUI_Master_subvi_reentrant_queues.vi"("STOP Queue in"=w32, "This Application"=w245, "error in (no error)"=w246, "tcp data event"=w244, "Caller menu reference"=w248, "Caller VI ref"=w249) -> ("error out"=→"error IO 2":errorcluster)  [unwired: 5 in]
      n942 = Unbundle By Name(w134) -> ("Data Value Reference out"=w133:refnum<k34>)
      n943 = for {
        tunnel: w163 -> [w253] mode=indexing
        tunnel: w162 -> [w252]
        tunnel: [w251] -> w132
        n944 = call "IMAQ Dispose"("Image"=w253, "error in (no error)"=w252) -> ("error out"=w251:errorcluster)  [unwired: 4 in]
      }
      n945 = TDMS Close(8:w132, 11:w133) -> (0:→"error out 2":errorcluster)  [unwired: 1 out]
    }
  }
